vi "COD主界面（列队使用）.vi"() -> (8 "多列列表框":i32(listbox))   [LabVIEW 2016, in "斯坦道CODMn.lvlib"]
uses:
  <vilib>/Analysis/6fits.llb/Curve Fitting Criteria.ctl
  <vilib>/Utility/miscctls.llb/LVPointTypeDef.ctl
  <vilib>/Utility/config.llb/Read Key (I32).vi
  <vilib>/Utility/config.llb/Read Key (Double).vi
  <vilib>/Utility/config.llb/Read Key (Boolean).vi
  <vilib>/Utility/config.llb/Write Key (I32).vi
  <vilib>/Utility/config.llb/Write Key (Double).vi
  <vilib>/Utility/config.llb/Write Key (Boolean).vi
  <vilib>/Waveform/WDTFileIO.llb/Read Waveform from File.vi
  <vilib>/ptbypt/NI_PtbyPt.lvlib
  <vilib>/Utility/config.llb/NI_LVConfig.lvlib
  <vilib>/Analysis/NI_AALPro.lvlib
panel:
  out "氢氧化钠":dbl
  in  "序列号变更":bool
  out "模块版本号":string
  in  "更新程序":bool
  out "进样无液体告警":bool
  out "校准内容显示":string
  out "60分钟超时报警":bool
  in  "远程校准量程":enum16{"L", "H"}(ring)
  in  "远程自动校准浓度":dbl
  in  "仪器参数":bool
  out "CODMn序列号":string
  out "CODMn软件版本：":string
  in  "标样核查量程选择":enum32{"H", "L", "AUTO"}(ring)=enum."AUTO"
  in  "标样浓度":dbl
  in  "零点核查量程选择":enum32{"H", "L", "AUTO"}(ring)=enum."AUTO"
  in  "零点核查浓度":dbl
  out "序列号":string
  in  "采水泵排液时间/s:":i32
  in  "采水泵润洗时间/s:":i32
  in  "采水泵沉淀时间/s:":i32
  in  "采水泵进样时间/s:":i32
  in  "常规版/认证版":enum16{"常规版-酸性", "常规版-碱性", "认证版", "浮台版"}(ring)
  in  "释放串口":bool
  in  "打开串口":bool
  in  "保存参数":dbl[](array[numeric])
  out "报警数字":i16
  out "CODMn工作状态":T1(ring)
  out "ORP-K":string
  out "ORP-B":string
  out "ORP-A":string
  out "x = y?":bool
  out "稀释倍数解释":string
  in  "跨度量程选择":enum32{"H", "L", "AUTO"}(ring)=enum."AUTO"
  in  "跨度液浓度":dbl
  in  "水样：":dbl
  in  "蒸馏水：":dbl
  in  "标液：":dbl
  in  "零点核查样：":dbl
  in  "加标回收样：":dbl
  in  "草酸钠":dbl
  in  "高锰酸钾":dbl
  in  "硫酸":dbl
  out "量程解释说明":string
  in  "高切低阈值:":dbl
  in  "低切高阈值:":dbl
  in  "水样量程选择:":enum16{"L", "H", "自动切换测一次", "自动切换测两次"}(ring)
  in  "氢氧化钠：":dbl
  in  "标准液浓度":dbl
  in  "温度":dbl
  in  "恒温时间":dbl
  in  "当前量程：":enum16{"L", "H"}(ring)
  in  "CODMn零点核查选择":enum16{"零点核查走纯水管", "零点核查走零漂管"}(ring)
  in  "锁定按钮":bool
  in  "低量程稀释倍数:":i8=1
  in  "高量程稀释倍数:":i8=2
  in  "一键写入":bool
  in  "测量模式(公式)":u16(ring)=1 items=["水样测试"=1, "标样核查"=2, "零点核查"=3, "跨度核查"=4, "空白测试"=5, "平行样"=6, "加标回收"=7]
  out "基本量程(显示)":string
  out "测量模式(显示)":string
  out "数据时间":string
  out "断电排液标记":bool
  out "COM":string
  in  "启用5":bool
  in  "校准5":bool
  in  "泵滴定数5":dbl
  in  "浓度5":dbl
  in  "启用4":bool
  in  "校准4":bool
  in  "泵滴定数4":dbl
  in  "浓度4":dbl
  out "波形时间":timestamp
  in  "历史波形":bool
  out "滴定数-ORP值":u16[](array[numeric]) caption="数组"
  in  "关闭 3":bool
  in  "滴定曲线":bool
  out "ORP滴定曲线":u16[](graph)
  out "空白测试标记":bool
  out "跨度核查标记":bool
  in  "量程选择":enum16{"低量程", "高量程", "0-2量程"}(ring)
  in  "手动控制":bool
  in  "选用水样":enum16{"葡萄糖", "草酸钠"}(ring)
  in  "方程系数":cluster{"K":dbl, "b":dbl, "X^2":dbl} {"X^2" format="%#.6g"; "b" format="%#.6g"; "K" format="%#.6g"}
  out "多项式系数":dbl[](array[numeric])
  out "XY图":cluster{"X Values":dbl[], "Y Values":dbl[]}[](graph)
  in  "模型":enum32{"线性", "多项式"}(ring)
  out "启动时间":timestamp format="%<%Y/%m/%d %H:%M:%S>T"
  in  "关闭 2":bool
  out "r^2":dbl format="%.8g"
  out "拟合公式":string
  out "b":dbl format="%#.4g"
  out "K":dbl format="%#.4f"
  in  "启用3":bool
  in  "启用2":bool
  in  "启用1":bool
  in  "校准3":bool
  in  "校准2":bool
  in  "校准1":bool
  in  "泵滴定数3":dbl
  in  "泵滴定数2":dbl
  in  "泵滴定数1":dbl
  in  "浓度3":dbl
  in  "浓度2":dbl
  in  "浓度1":dbl
  in  "写入":bool
  out "零点核查标记":bool
  out "排液故障":bool
  out "进水样超量程":bool
  out "标样核查标记":bool
  out "平行样测量":bool
  out "加标回收测量":bool
  out "质控样测量":bool
  out "待机":bool
  out "校标错误":bool
  out "校零错误":bool
  out "测量错误":bool
  out "草酸钠报警":bool
  out "高锰酸钾报警":bool
  out "加热故障":bool
  out "温控器故障":bool
  out "ORP故障":bool
  out "排液标记":bool
  out "故障标记":bool
  out "校标标记":bool
  out "校零标记":bool
  out "通讯状态":bool
  out "水样测量":bool
  in  "读取":bool
  in  "返回":bool
  in  "校准配置":bool
  in  "零点泵计量数 2":dbl
  in  "标度泵计量数 2":dbl
  out "标度滴定值":dbl
  out "零点滴定值":dbl
  in  "保存":bool
  in  "关闭":bool
  out "仪器时间":timestamp format="%<%Y/%m/%d %H:%M:%S>T"
  out "秒":u16
  out "分":u16
  out "COD浓度（mg/L)":dbl format="%.2g"
  out "进样管":dbl
  out "高锰酸钾":dbl
  out "草酸钠":dbl
  out "硫酸":dbl
  out "实时ORP":dbl
  out "温度℃":dbl
  out "加热":bool
  out "搅拌":bool
  out "进硫酸":bool
  out "进加标回收样":bool
  out "进零点核查样":bool
  out "进标液":bool
  out "进蒸馏水":bool
  out "进水样":bool
  out "进草酸钠":bool
  out "进高锰酸钾":bool
  out "定时启动":bool
  in  "启动":bool
  in  "故障清除":bool
  in  "参数配置":bool
  in  "停止":bool
  in  "单步启动":bool
  out "系统时间":timestamp
  in  "时间校准":bool
  out "模式（受控）":u16
  # "测试时长："
  # "注：遇到加热故障和排液故障时仪器不能正常启动，\n必须排查故障并点击报警清除按钮方可运行。"
  # "mg/L"
  # "基本参数设置"
  # "校零校标结果"
  # "泵计量参数设置"
  # "校零结果："
  # "校零滴定值："
  # "加热恒温温度(℃):"
  # "高锰酸钾："
  # "校标结果："
  # "标度滴定值："
  # "恒温时间(分钟):"
  # "草酸钠："
  # "零点泵计量值："
  # "标准液浓度(mg/L):"
  # "硫酸："
  # "标度泵计量值："
  # "跨度核查浓度："
  # "跨度量程选择："
  # "零点核查浓度："
  # "标样浓度："
  # "零点量程选择："
  # "标样量程选择："
  # "远程校准配置区"
  # "公式读取写入区"
  # "mg/L"
  # "是否启用"
  # "泵滴定数"
  # "浓度"
  # "辅\n助\n计\n算\n区"
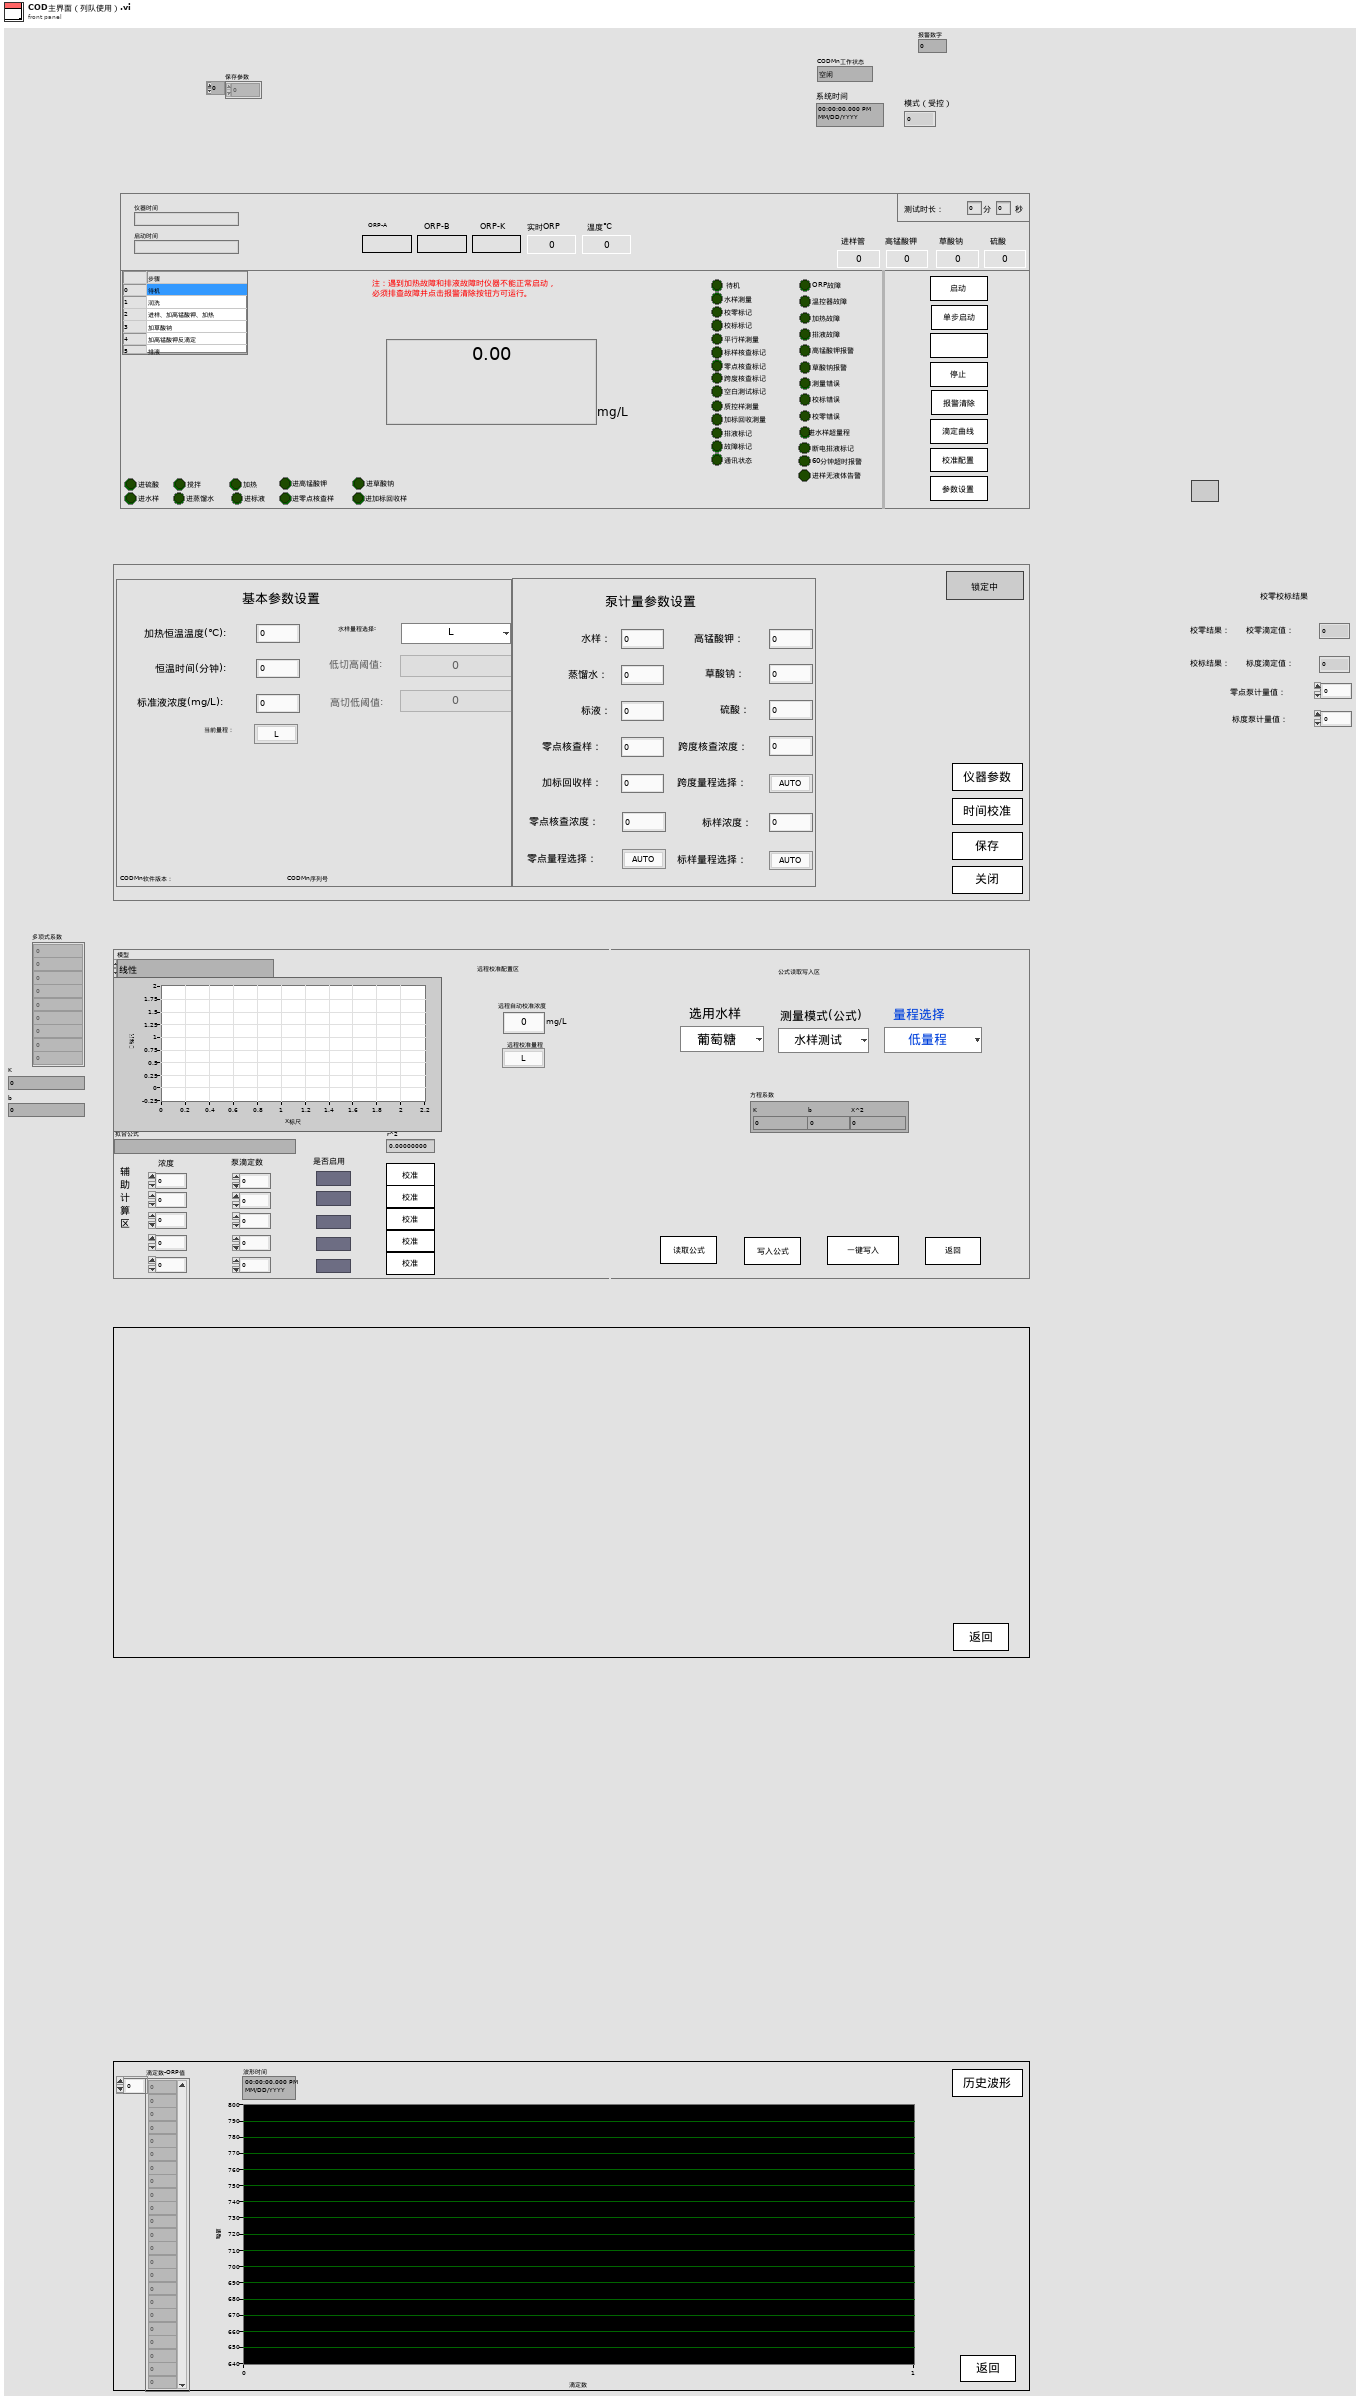
[diagram p1: front panel]
types:
  T1 = enum16{"空闲", "水样测试", "标样核查", "零点核查", "跨度核查", "空白测试", "平行样测试", "质控样", "空白校准", "标样校准", "加标回收"}
  T2 = typedef "LVPointTypeDef.ctl" = cluster{"Horizontal":i16, "Vertical":i16}
  T3 = cluster{"Major":u16, "Minor":u16, "Fix":u16, "Build":u16}
  T4 = typedef "NI_LVConfig.lvlib/Config Data RefNum.ctl" = refnum<k1>
  T5 = cluster{"时间标识":timestamp, "参数":string, "日志信息":string, "流程参数":string}
  T6 = cluster{"时间标识":timestamp, "设备":string, "日志信息":string, "流程参数":string}
  T7 = enum8{"Enabled", "Disabled", "Disabled and Grayed Out"}
  T8 = cluster{"时间":timestamp, "测量模式":string, "数据类型":string, "检测值":sgl, "单位":string, "数据标识":string, "因子编码":string, "标样参考值":sgl, "ORP-A":sgl, "ORP-B":sgl, "ORP-K":sgl, "COD滴定值":sgl, "高锰酸钾滴定数":sgl, "温度":sgl, "量程":sgl, "LastTime":timestamp, "序列号:":string}
  T9 = cluster{"因子编码":u32, "单位":u16, "标样参考值":sgl, "水样数据时间":timestamp, "水样实测值":sgl, "水样数据标识":string, "标样数据时间":timestamp, "标样实测值":sgl, "标样数据标识":string, "空白数据时间":timestamp, "空白实测值":sgl, "空白数据标识":string, "零点核查数据时间":timestamp, "零点核查实测值":sgl, "零点核查数据标识":string, "跨度核查数据时间":timestamp, "跨度核查实测值":sgl, "跨度核查数据标识":string, "加标回收数据时间":timestamp, "加标回收实测值":sgl, "加标回收数据标识":string, "平行样数据时间":timestamp, "平行样实测值":sgl, "平行样数据标识":string}
  T10 = cluster{"控制命令":enum16{"启动测量", "标样核查", "零点核查", "跨度核查", "空白测试", "平行样测试", "加标回收", "空白校准", "标样校准", "初始化（清洗）", "停止测试", "仪器重启", "校时", "模式设置", "测量间隔设置"}, "周期设置类型":enum16{"定点启动", "间隔启动"}, "定时功能启用":bool, "定时间隔":dbl, "24H周期设置":bool[], "零点核查时间":u16, "跨度核查时间":u16, "质控频次":enum16{"关闭", "每天", "星期一", "星期二", "星期三", "星期四", "星期五", "星期六", "星期日"}}
  T11 = cluster{"数组 2[0]":sgl, "数组 2[1]":sgl, "数组 2[2]":sgl, "数组 2[3]":sgl, "数组 2[4]":sgl, "数组 2[5]":sgl, "数组 2[6]":sgl, "数组 2[7]":sgl, "数组 2[8]":sgl, "数组 2[9]":sgl, "数组 2[10]":sgl, "数组 2[11]":sgl, "数组 2[12]":sgl, "数组 2[13]":sgl, "数组 2[14]":sgl, "数组 2[15]":sgl, "数组 2[16]":sgl, "数组 2[17]":sgl, "数组 2[18]":sgl, "数组 2[19]":sgl, "数组 2[20]":sgl, "数组 2[21]":sgl, "数组 2[22]":sgl, "数组 2[23]":sgl, "数组 2[24]":sgl, "数组 2[25]":sgl, "数组 2[26]":sgl, "数组 2[27]":sgl, "数组 2[28]":sgl, "数组 2[29]":sgl, "数组 2[30]":sgl, "数组 2[31]":sgl, "数组 2[32]":sgl, "数组 2[33]":sgl, "数组 2[34]":sgl, "数组 2[35]":sgl, "数组 2[36]":sgl, "数组 2[37]":sgl, "数组 2[38]":sgl, "数组 2[39]":sgl, "数组 2[40]":sgl, "数组 2[41]":sgl}
  T12 = cluster{"ORP故障":bool, "温控器故障":bool, "加热故障":bool, "高锰酸钾报警":bool, "草酸钠报警":bool, "测量错误":bool, "校零错误":bool, "校标错误":bool, " 进水样超量程":bool, "排液阀故障":bool, "60分钟超时报警":bool, "进样无液体报警":bool}
  T13 = cluster{"控制命令":enum16{"启动测量", "标样核查", "零点核查", "跨度核查", "空白测试", "平行样测试", "加标回收", "空白校准", "标样校准", "初始化（清洗）", "停止测试", "仪器重启", "校时", "模式设置", "测量间隔设置"}, "周期设置类型":enum16{"定点启动", "间隔启动"}, "定时功能启用":bool, "定时间隔":dbl, "24H周期设置":bool[], "空白核查时间":u16, "跨度核查时间":u16, "质控频次":enum16{"关闭", "每天", "星期一", "星期二", "星期三", "星期四", "星期五", "星期六", "星期日"}}
  T14 = cluster{"测量量程":dbl, "测量精度":dbl, "测量间隔":dbl, "消解温度":dbl, "消解时长":dbl, "空白校准时间":timestamp, "曲线截距":dbl, "曲线斜率":dbl, "测量检出限":dbl, "测量信号值":dbl, "线性相关系数":dbl, "二次多项式系数":dbl, "标样校准时间":timestamp, "稀释倍数":dbl, "三项式系数":dbl, "空白标定系数":dbl, "量程系数":dbl, "F0/ORPA":dbl, "F1/ORPB":dbl, "F2/ORPK":dbl, "F3":dbl, "F4":dbl, "F5":dbl, "F6":dbl, "F7":dbl, "X0/滴定数":dbl, "量程":dbl}
  T15 = cluster{"确定":bool, "测量量程":dbl, "测量精度":dbl, "测量间隔":dbl, "消解温度":dbl, "消解时长":dbl, "空白校准时间":timestamp, "曲线截距":dbl, "曲线斜率":dbl, "测量检出限":dbl, "测量信号值":dbl, "线性相关系数":dbl, "二次多项式系数":dbl, "标样校准时间":timestamp, "稀释倍数":dbl, "三项式系数":dbl, "空白标定系数":dbl, "量程系数":dbl, "F0/ORPA":dbl, "F1/ORPB":dbl, "F2/ORPK":dbl, "F3":dbl, "F4":dbl, "F5":dbl, "F6":dbl, "F7":dbl, "X0/滴定数":dbl, "量程":dbl}
  T16 = typedef "NI_AALPro.lvlib/Curve Fitting Criteria.ctl" = u16
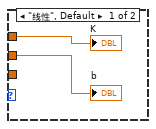
[diagram p5: hidden frame]
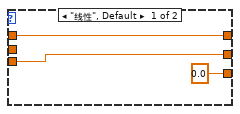
[diagram p7: hidden frame]
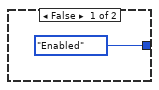
[diagram p8: hidden frame]
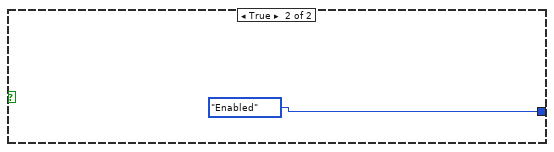
[diagram p9: hidden frame]
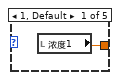
[diagram p14: hidden frame]
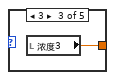
[diagram p15: hidden frame]
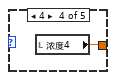
[diagram p16: hidden frame]
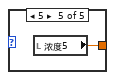
[diagram p17: hidden frame]
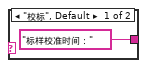
[diagram p18: hidden frame]
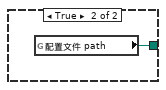
[diagram p19: hidden frame]
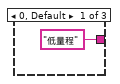
[diagram p20: hidden frame]
diagram:
  n1 = flat-sequence {
    tunnel: w1 -> [_]
    frame #0 {
      w18 = u16 1 items=["水样测试"=1, "标样核查"=2, "零点核查"=3, "跨度核查"=4, "空白测试"=5, "平行样"=6, "加标回收"=7] ("测量模式(公式)")
      n2 = vi-ref "斯坦道CODMn.lvlib:待机状态数据存储写入和切换量程(子VI).vi"() -> (w63:refnum<vi>)
      n3 = vi-ref "斯坦道CODMn.lvlib:定时启动 (子VI).vi"() -> (w50:refnum<vi>)
      n4 = vi-ref "斯坦道CODMn.lvlib:日志报警状态存储 (子VI).vi"() -> (w49:refnum<vi>)
      n5 = vi-ref "斯坦道CODMn.lvlib:高锰酸钾-ORP滴定曲线(子VI).vi"() -> (w36:refnum<vi>)
      n6 = property class="VI"(reference=w50, error in=errorcluster {"status"=FALSE, "code"=0, "source"=""} ("错误输出")) -> ("Name"=w51:string)  [unwired: 2 out]
      n7 = property class="VI"(reference=w49, error in=errorcluster {"status"=FALSE, "code"=0, "source"=""} ("错误输出")) -> ("Name"=w48:string)  [unwired: 2 out]
      n8 = property class="VI"(reference=w36, error in=errorcluster {"status"=FALSE, "code"=0, "source"=""} ("错误输出")) -> ("Name"=w37:string)  [unwired: 2 out]
      n9 = Open VI Reference(type specifier VI Refnum (for type only)=refnum<vi> refnum, vi path=w51, options=128 ("选项")) -> (vi reference=w31:refnum<vi>, error out=w53:errorcluster)  [unwired: 3 in]
      n10 = property class="VI"(reference=w63, error in=errorcluster {"status"=FALSE, "code"=0, "source"=""} ("错误输出")) -> ("Name"=w62:string)  [unwired: 2 out]
      n11 = call-by-ref "?"(reference=w31, error in=w53) -> (reference out=w55:refnum<vi>, error out=w54:errorcluster)  [unwired: 12 in]
      n12 = Open VI Reference(type specifier VI Refnum (for type only)=refnum<vi> refnum, vi path=w48, options=128 ("选项")) -> (vi reference=w32:refnum<vi>, error out=w46:errorcluster)  [unwired: 3 in]
      n13 = Open VI Reference(type specifier VI Refnum (for type only)=refnum<vi> refnum, vi path=w37, options=128 ("选项")) -> (vi reference=w35:refnum<vi>, error out=w39:errorcluster)  [unwired: 3 in]
      n14 = call-by-ref "?"(reference=w32, error in=w46) -> (reference out=w44:refnum<vi>, error out=w45:errorcluster)  [unwired: 12 in]
      n15 = Close Reference(reference=w55, error in (no error)=w54) -> ()  [unwired: 1 out]
      n16 = call-by-ref "?"(reference=w35, error in=w39) -> (reference out=w41:refnum<vi>, error out=w40:errorcluster)  [unwired: 12 in]
      n17 = Open VI Reference(type specifier VI Refnum (for type only)=refnum<vi> refnum, vi path=w62, options=128 ("选项")) -> (vi reference=w28:refnum<vi>, error out=w60:errorcluster)  [unwired: 3 in]
      n18 = Close Reference(reference=w44, error in (no error)=w45) -> ()  [unwired: 1 out]
      n19 = call-by-ref "?"(reference=w28, error in=w60) -> (reference out=w58:refnum<vi>, error out=w59:errorcluster)  [unwired: 12 in]
      n20 = Close Reference(reference=w41, error in (no error)=w40) -> ()  [unwired: 1 out]
      n21 = Close Reference(reference=w58, error in (no error)=w59) -> ()  [unwired: 1 out]
      n22 = vi-ref "斯坦道CODMn.lvlib:关键参数交互.vi"() -> (w25:refnum<vi>)
      n23 = property class="VI"(reference=w25, error in=errorcluster {"status"=FALSE, "code"=0, "source"=""} ("错误输出")) -> ("Name"=w24:string)  [unwired: 2 out]
      n24 = Open VI Reference(type specifier VI Refnum (for type only)=refnum<vi> refnum, vi path=w24, options=128 ("选项")) -> (vi reference=w26:refnum<vi>, error out=w22:errorcluster)  [unwired: 3 in]
      n25 = call-by-ref "?"(reference=w26, error in=w22, "量程选择"=enum16{"低量程", "高量程", "0-2量程"}."低量程", "测量模式(公式)"=w18, "模型"=enum32{"线性", "多项式"}."线性") -> (reference out=w20:refnum<vi>, error out=w21:errorcluster)  [unwired: 9 in]
      n26 = Close Reference(reference=w20, error in (no error)=w21) -> ()  [unwired: 1 out]
    }
  }
  n27 = flat-sequence {
    tunnel: [w66] -> w3
    tunnel: [errorcluster {"status"=FALSE, "code"=0, "source"=""} ("错误输出")] -> w1
    tunnel: [w68] -> w2
    frame #0 {
      w90 = "192.168.1.100" ("名称")
      n28 = global write "COD内部交互全局.vi" "量程切换次数"(u8 0 ("量程切换次数")) -> ()
      n29 = global write "COD内部交互全局.vi" "切换量程连续测两次"(FALSE ("切换量程连续测两次")) -> ()
      n30 = global read "COD内部交互全局.vi" "序列号:"() -> (w97:string)
      n31 = property on="窗格" class="Pane"("Origin"=T2 {"Horizontal"=0, "Vertical"=0} ("原点")) -> ()  [unwired: 2 in, 2 out]
      n32 = Empty String/Path?(string/path=w97) -> (empty?=w65:bool)
      n33 = case shown="真" w65 {
        tunnel: w97 -> [w112 _]
        tunnel: [w111 "data\\CODMnSet.ini" ("名称或相对路径")] -> w78
        frame False {
          # "与生产用上位机交互"
          n34 = Concatenate Strings("data\\" ("字符串"), "序列号" ("字符串"), w112, "Set.ini" ("名称或相对路径")) -> (w111:string)
        }
        frame True {
        }
      }
      n35 = String To IP(1:w90) -> (0:w83:u32)
      n36 = IP To String(2:w83) -> (0:w86:string)  [unwired: 1 in]
      n37 = Not Equal?(x=w90, y=w86) -> (x != y?=w91:bool)
      n38 = Concatenate Strings("\\\\" ("字符串"), w86) -> (w85:string)
      n39 = global write "CODMN外部API.vi" "ping"(w91) -> ()
      n40 = String To Path(string=w85) -> (path=w92:path)
      n41 = Build Path(base path=w92, name or relative path=w78) -> (appended path=w87:path)
      n42 = local write "量程选择"(enum16{"低量程", "高量程", "0-2量程"}."低量程" ("量程选择")) -> ()
      n43 = local write "选用水样"(enum16{"葡萄糖", "草酸钠"}."葡萄糖" ("选用水样")) -> ()
      n44 = global write "COD内部交互全局.vi" "配置文件ini"(w78) -> ()
      n45 = case shown="真" w91 {
        tunnel: w87 -> [w102 w106]
        tunnel: [w102 w105] -> w88
        tunnel: [FALSE w104] -> w89
        frame False {
        }
        frame True {
          n46 = call <vilib>:"Check if File or Folder Exists.vi"("path"=w106) -> ("file or folder exists?"=w104:bool, "dup path"=w105:path)  [unwired: 8 in, 1 out]
        }
      }
      n47 = control-ref of="本VI"() -> (w77:refnum<vi>)
      n48 = case shown="假" w89 {
        tunnel: w88 -> [_ w110]
        tunnel: [w108 w110] -> w69
        tunnel: w78 -> [w107 _]
        frame False {
          # "本地文件地址"
          n49 = call <vilib>:"Application Directory.vi"() -> ("Application Directory"=w109:path)
          n50 = Build Path(base path=w109, name or relative path=w107) -> (appended path=w108:path)
        }
        frame True {
          # "网络共享地址"
        }
      }
      n51 = property class="VI"(reference=w77) -> ("Library.Version"=w76:T3)  [unwired: 1 in, 2 out]
      n52 = Unbundle By Name(w76) -> ("Major"=w74:u16, "Minor"=w73:u16, "Fix"=w72:u16, "Build"=w71:u16)
      n53 = Format Into String(format string="模块版本号：%d.%d.%d.%d" ("格式字符串"), w74, w73, w72, w71) -> (resulting string=→"模块版本号":string)  [unwired: 2 in, 1 out]
      n54 = global write "CODMN外部API.vi" "配置文件 path"(w69) -> ()
      n55 = call <vilib>:"Open Config Data.vi"("configuration file path"=w69) -> ("error out"=w79:errorcluster, "refnum"=w80:T4)  [unwired: 8 in, 1 out]
      n56 = vi-ref "斯坦道CODMn.lvlib:CODMn断电保存全局变量.vi"() -> (w93:refnum<vi>)
      n57 = call <userlib>:"Read Panel from INI__ogtk.vi"("error in (no error)"=w79, "VI ref"=w93, "refnum"=w80) -> ("error out"=w81:errorcluster, "refnum out"=w82:T4)  [unwired: 7 in]
      n58 = call <vilib>:"Close Config Data.vi"("error in (no error)"=w81, "refnum"=w82) -> ("error out"=w67:errorcluster)  [unwired: 8 in, 1 out]
      n59 = call <vilib>:"Clear Errors.vi"("error in (no error)"=w67) -> ("error out"=w64:errorcluster)  [unwired: 5 in, 1 out]
      n60 = Read from Text File(file (use dialog)=w69, error in=w64) -> (text=w68:string, error out=w66:errorcluster)  [unwired: 2 in, 2 out]
      "稀释倍数解释" <- "稀释倍数解释：\n稀释倍数选择1，表示不稀释\n默认低量程系数倍数1，高量程系数倍数2\n则低量程为0~8，高量程为0~16" ("稀释倍数解释")
    }
  }
  n61 = Obtain Queue(name (unnamed)="CODMn" ("名称（未命名）"), element data type=cluster{"命令":string} {"命令"="启用模块"} ("元素")) -> (queue out=w13:refnum<queue>, error out=w12:errorcluster)  [unwired: 3 in, 1 out]
  n62 = while {
    tunnel: [w123] -> _
    shift-right: [w121] -> _
    shift-left: w2 -> [w120]
    tunnel: w3 -> [_]
    stop <- FALSE stop-if-true
    n63 = global read "CODMN外部API.vi" "配置文件 path"() -> (w117:path)
    n64 = Wait (ms)(milliseconds to wait=u32 1000 ("等待时间（毫秒）")) -> ()  [unwired: 1 out]
    n65 = Read from Text File(file (use dialog)=w117) -> (text=w121:string, error out=w118:errorcluster)  [unwired: 3 in, 2 out]
    n66 = Not Equal?(x=w121, y=w120) -> (x != y?=w119:bool)
    n67 = case shown="真" w119 {
      tunnel: [w125 w132] -> w123
      tunnel: w117 -> [_ w126]
      tunnel: w118 -> [w125 _]
      frame False {
      }
      frame True {
        # "文件发生改变进行更新，远端和本地都更新"
        n68 = vi-ref "斯坦道CODMn.lvlib:CODMn断电保存全局变量.vi"() -> (w127:refnum<vi>)
        n69 = call <vilib>:"Open Config Data.vi"("configuration file path"=w126) -> ("error out"=w131:errorcluster, "refnum"=w130:T4)  [unwired: 8 in, 1 out]
        n70 = call <userlib>:"Read Panel from INI__ogtk.vi"("error in (no error)"=w131, "VI ref"=w127, "refnum"=w130) -> ("error out"=w129:errorcluster, "refnum out"=w128:T4)  [unwired: 7 in]
        n71 = call <vilib>:"Close Config Data.vi"("error in (no error)"=w129, "refnum"=w128) -> ("error out"=w132:errorcluster)  [unwired: 8 in, 1 out]
      }
    }
  }
  n72 = vi-ref "CODMn通讯.vi"() -> (w4:refnum<vi>)
  n73 = while {
    stop <- FALSE stop-if-true
    # "相差60秒自动校时"
    n74 = global read "运行时序全局变量.vi" "多列列表框"() -> (w134:i32)
    n75 = local read "仪器时间"() -> (w141:timestamp)
    n76 = local read "系统时间"() -> (w142:timestamp)
    n77 = Wait (ms)(milliseconds to wait=u32 1000 ("等待时间（毫秒）")) -> ()  [unwired: 1 out]
    n78 = Build Array(w141) -> (w140:timestamp[])
    n79 = Build Array(w142) -> (w159:timestamp[])
    n80 = Equal?(x=w134, y=u16 5) -> (x = y?=w136:bool)
    n81 = call <vilib>:"Boolean Crossing PtByPt.vi"("direction"=enum16{"either", "false-true", "true-false"}."false-true", "input"=w136) -> ("crossing"=w133:bool)  [unwired: 1 in]
    n82 = call "DateToHex.vi"("DATE"=w140) -> ("数组"=w153:u16[])  [unwired: 10 in]
    n83 = call "DateToHex.vi"("DATE"=w159) -> ("数组"=w158:u16[])  [unwired: 10 in]
    n84 = case shown="真" w133 {
      frame False {
      }
      frame True {
        # "校准结束后自动更新曲线泵滴定数"
        n85 = global read "COD测量模式全局.vi" "测量模式文字实时"() -> (w160:string)
        n86 = global read "COD测量模式全局.vi" "测量模式文字实时"() -> (w165:string)
        n87 = global read "CODMN外部API.vi" "远程反控校准CODMn"() -> (w164:bool)
        n88 = global read "COD内部交互全局.vi" "高锰酸钾"() -> (w168:dbl)
        n89 = Equal?(x=w160, y="校零") -> (x = y?=w161:bool)
        n90 = Equal?(x=w165, y="校标") -> (x = y?=w167:bool)
        n91 = Or(x=w161, y=w167) -> (x .or. y?=w163:bool)
        n92 = case shown="真" w163 {
          tunnel: w168 -> [_ w175]
          tunnel: w160 -> [_ w172]
          frame False {
          }
          frame True {
            w199 = "量程选择" ("section")
            n93 = global read "CODMN外部API.vi" "ping"() -> (w210:bool)
            n94 = case shown="\"校零\"" w172 {
              tunnel: ["标样校准时间：" "空白校准时间："] -> w178
              frame "校标", Default {
              }
              frame "校零" {
              }
            }
            n95 = case shown="假" w210 {
              tunnel: [w219 w222] -> w211
              frame False {
                n96 = global read "COD内部交互全局.vi" "配置文件ini"() -> (w221:string)
                n97 = call <vilib>:"Application Directory.vi"() -> ("Application Directory"=w220:path)
                n98 = Build Path(base path=w220, name or relative path=w221) -> (appended path=w219:path)
              }
              frame True {
                n99 = global read "CODMN外部API.vi" "配置文件 path"() -> (w222:path)
              }
            }
            n100 = Number To Fractional String(number=w175) -> (F-format string=w180:string)  [unwired: 3 in]
            n101 = call <vilib>:"Open Config Data.vi"("configuration file path"=w211) -> ("error out"=w198:errorcluster, "refnum"=w197:T4)  [unwired: 8 in, 1 out]
            n102 = Get Date/Time In Seconds() -> (seconds since 1Jan1904=w176:timestamp)
            n103 = Format Date/Time String(time format string (%c)="%Y/%m/%d %H:%M:%S" ("时间格式字符串(%c)"), seconds (now)=w176) -> (date/time string=w177:string)  [unwired: 1 in]
            n104 = call-poly <vilib>:"Read Key.vi"("section"="标线选择", "error in (no error)"=w198, "key"="选用水样", "refnum"=w197) -> ("error out"=w200:errorcluster, "value"=w193:i32, "refnum out"=w201:T4)  [unwired: 4 in, 1 out]
            n105 = local write "选用水样"(w193) -> ()
            n106 = call-poly <vilib>:"Read Key.vi"("section"=w199, "error in (no error)"=w200, "key"=w199, "refnum"=w201) -> ("error out"=w194:errorcluster, "value"=w196:i32, "refnum out"=w195:T4)  [unwired: 4 in, 1 out]
            n107 = case shown="1" w193 {
              tunnel: ["葡萄糖标线" ("section") "草酸钠标线" ("section")] -> w208
              frame 0, Default {
              }
              frame 1 {
              }
            }
            n108 = local write "量程选择"(w196) -> ()
            n109 = case shown="2" w196 {
              tunnel: ["低量程" "高量程" "0-2量程"] -> w207
              frame 0, Default {
              }
              frame 1 {
              }
              frame 2 {
              }
            }
            n110 = Concatenate Strings(w208, w207) -> (w209:string)
            n111 = call-poly <vilib>:"Read Key.vi"("section"=w209, "error in (no error)"=w194, "key"="当前选用的校准" ("section"), "refnum"=w195) -> ("error out"=w206:errorcluster, "value"=w171:i32, "refnum out"=w205:T4)  [unwired: 4 in, 1 out]
            n112 = call <vilib>:"Close Config Data.vi"("error in (no error)"=w206, "refnum"=w205) -> ()  [unwired: 8 in, 2 out]
            n113 = case shown="2" w171 {
              tunnel: [w212 w213 w214 w215 w216] -> w170
              frame 1, Default {
                n114 = local read "浓度1"() -> (w212:dbl)
              }
              frame 2 {
                n115 = local read "浓度2"() -> (w213:dbl)
              }
              frame 3 {
                n116 = local read "浓度3"() -> (w214:dbl)
              }
              frame 4 {
                n117 = local read "浓度4"() -> (w215:dbl)
              }
              frame 5 {
                n118 = local read "浓度5"() -> (w216:dbl)
              }
            }
            n119 = Number To Fractional String(number=w170) -> (F-format string=w182:string)  [unwired: 3 in]
            n120 = Concatenate Strings("信息：校准结果：\n", "校准浓度：", w182, "滴定数：", w180, w178, w177) -> (w174:string)
            n121 = Bundle(cluster=T5 {"时间标识"=timestamp(0 s since 1904-01-01), "参数"="", "日志信息"="", "流程参数"=""} ("data in"), "时间标识"=w176, "参数"="CODMn" ("table输入"), "日志信息"=w174, "流程参数"="" ("table输入")) -> (w186:T5)
            n122 = call "流程日志字段定义.vi"("table输入"="校准记录", "data in"=w186) -> ("table输出"=w190:string, "columns"=w191:string[], "data out"=w192:T6)  [unwired: 7 in]
            n123 = call "插入数据.vi"("data"=w192, "columns"=w191, "database"="database3.mdb", "table"=w190) -> ()  [unwired: 7 in, 1 out]
            n124 = global write "COD内部交互全局.vi" "当前校准"(w171) -> ()
            n125 = case shown="1, 默认" w171 {
              tunnel: w175 -> [w228 w229 w230 w231 w232]
              frame 1, Default {
                n126 = property on="泵滴定数1" class="DigNum (严格)"("Val(Sgnl)"=w228) -> ()  [unwired: 2 in, 2 out]
              }
              frame 2 {
                n127 = property on="泵滴定数2" class="DigNum (严格)"("Val(Sgnl)"=w229) -> ()  [unwired: 2 in, 2 out]
              }
              frame 3 {
                n128 = property on="泵滴定数3" class="DigNum (严格)"("Val(Sgnl)"=w230) -> ()  [unwired: 2 in, 2 out]
              }
              frame 4 {
                n129 = property on="泵滴定数4" class="DigNum (严格)"("Val(Sgnl)"=w231) -> ()  [unwired: 2 in, 2 out]
              }
              frame 5 {
                n130 = property on="泵滴定数5" class="DigNum (严格)"("Val(Sgnl)"=w232) -> ()  [unwired: 2 in, 2 out]
              }
            }
          }
        }
        n131 = case shown="真" w164 {
          frame False {
          }
          frame True {
            # "校准完自动写入公式"
            n132 = global write "CODMN外部API.vi" "远程反控校准CODMn"(FALSE ("远程反控校准CODMn")) -> ()
          }
        }
      }
    }
    n133 = Index Array(array=w153, index=2 ("索引")) -> (element=w155:u16)
    n134 = Index Array(array=w158, index=2 ("索引")) -> (element=w156:u16)
    n135 = Split Number(x=w155) -> (hi(x)=w149:u8)  [unwired: 1 out]
    n136 = Split Number(x=w156) -> (hi(x)=w152:u8)  [unwired: 1 out]
    n137 = To Byte Integer(number=w149) -> (8bit integer=w148:i8)
    n138 = To Byte Integer(number=w152) -> (8bit integer=w151:i8)
    n139 = Subtract(x=w148, y=w151) -> (x-y=w150:i8)
    n140 = Absolute Value(x=w150) -> (abs(x)=w147:i8)
    n141 = local read "通讯状态"() -> (w144:bool)
    n142 = Greater Or Equal?(x=w147, y=i8 5) -> (x >= y?=w145:bool)
    n143 = And(x=w145, y=w144) -> (x .and. y?=w143:bool)
    n144 = case shown="真" w143 {
      frame False {
      }
      frame True {
        # "相差60秒时间自动校准"
        n145 = flat-sequence {
          frame #0 {
            n146 = property on="时间校准" class="Bool (严格)"("Val(Sgnl)"=TRUE ("值(信号)")) -> ()  [unwired: 2 in, 2 out]
          }
          frame #1 {
            n147 = Wait (ms)(milliseconds to wait=u32 500 ("等待时间（毫秒）")) -> ()  [unwired: 1 out]
          }
          frame #2 {
            n148 = property on="时间校准" class="Bool (严格)"("Val(Sgnl)"=FALSE ("值(信号)")) -> ()  [unwired: 2 in, 2 out]
          }
        }
      }
    }
  }
  n149 = while {
    tunnel: w3 -> [_]
    stop <- FALSE stop-if-true
    # "赋值循环"
    n150 = flat-sequence {
      frame #0 {
        # "测量数据区"
        n151 = global read "COD内部交互全局.vi" "data"() -> (w480:T8)
        n152 = global read "COD测量模式全局.vi" "测量模式文字实时"() -> (w466:string)
        "测量模式(显示)" <- w466
        n153 = global read "CODMn断电保存全局变量.vi" "测量数据区"() -> (w475:T9)
        n154 = Unbundle By Name(w480) -> ("时间"=w479:timestamp, "检测值"=w478:sgl, "数据标识"=w477:string)
        n155 = case shown="\"水样测试\"" w466 {
          tunnel: w475 -> [w481 w486 w491 w496 w501 w506 w511 w516 w521 w526]
          tunnel: [w481 w485 w490 w492 w500 w505 w510 w515 w517 w525] -> w476
          tunnel: w479 -> [_ w484 w489 w495 w499 w504 w509 w514 w520 w524]
          tunnel: w478 -> [_ w483 w488 w494 w498 w503 w508 w513 w519 w523]
          tunnel: w477 -> [_ w482 w487 w493 w497 w502 w507 w512 w518 w522]
          frame "", Default {
          }
          frame "水样测试" {
            n156 = Bundle By Name(cluster=w486, "水样数据时间"=w484, "水样实测值"=w483, "水样数据标识"=w482) -> (w485:T9)
          }
          frame "标样核查" {
            n157 = Bundle By Name(cluster=w491, "标样数据时间"=w489, "标样实测值"=w488, "标样数据标识"=w487) -> (w490:T9)
          }
          frame "跨度核查" {
            n158 = Bundle By Name(cluster=w496, "跨度核查数据时间"=w495, "跨度核查实测值"=w494, "跨度核查数据标识"=w493) -> (w492:T9)
          }
          frame "零点核查" {
            n159 = Bundle By Name(cluster=w501, "零点核查数据时间"=w499, "零点核查实测值"=w498, "零点核查数据标识"=w497) -> (w500:T9)
          }
          frame "空白测试" {
            n160 = Bundle By Name(cluster=w506, "空白数据时间"=w504, "空白实测值"=w503, "空白数据标识"=w502) -> (w505:T9)
          }
          frame "加标回收" {
            n161 = Bundle By Name(cluster=w511, "加标回收数据时间"=w509, "加标回收实测值"=w508, "加标回收数据标识"=w507) -> (w510:T9)
          }
          frame "平行样" {
            n162 = Bundle By Name(cluster=w516, "平行样数据时间"=w514, "平行样实测值"=w513, "平行样数据标识"=w512) -> (w515:T9)
          }
          frame "校零" {
            n163 = Bundle By Name(cluster=w521, "空白数据时间"=w520, "空白实测值"=w519, "空白数据标识"=w518) -> (w517:T9)
          }
          frame "校标" {
            n164 = Bundle By Name(cluster=w526, "标样数据时间"=w524, "标样实测值"=w523, "标样数据标识"=w522) -> (w525:T9)
          }
        }
        n165 = Unbundle By Name(w475) -> ("水样实测值"=w472:sgl)
        n166 = feedback-in #1(w475) -> ()
        n167 = feedback #1(w475) -> (w474:T9)
        n168 = global read "CODMn断电保存全局变量.vi" "水样测试量程"() -> (w468:enum16{"L", "H"})
        n169 = Unbundle By Name(w474) -> ("水样实测值"=w473:sgl)
        n170 = feedback #2(w468) -> (w469:enum16{"L", "H"})
        n171 = feedback-in #2(w468) -> ()
        n172 = Not Equal?(x=w469, y=w468) -> (x != y?=w467:bool)
        n173 = Not Equal?(x=w472, y=w473) -> (x != y?=w471:bool)
        n174 = global write "CODMn断电保存全局变量.vi" "测量数据区"(w476) -> ()
        n175 = Or(x=w471, y=w467) -> (x .or. y?=w470:bool)
        n176 = case shown="真" w470 {
          frame False {
          }
          frame True {
            # "水样值发送改变存储本地"
            n177 = call "配置文件保存.vi"() -> ()  [unwired: 12 in]
          }
        }
      }
    }
    n178 = flat-sequence {
      frame #0 {
        # "局部变量给内部交互用全局变量"
        n179 = local read "温度℃"() -> (w262:dbl)
        n180 = local read "COD浓度（mg/L)"() -> (w268:dbl)
        n181 = local read "CODMn工作状态"() -> (w271:T1)
        n182 = local read "多列列表框"() -> (w269:i32)
        n183 = local read "标准液浓度"() -> (w267:dbl)
        n184 = local read "高锰酸钾报警"() -> (w265:bool)
        n185 = local read "断电排液标记"() -> (w264:bool)
        n186 = local read "实时ORP"() -> (w261:dbl)
        n187 = local read "故障标记"() -> (w270:bool)
        n188 = local read "高锰酸钾"() -> (w263:dbl)
        n189 = global write "COD内部交互全局.vi" "实时温度"(w262) -> ()
        n190 = local read "待机"() -> (w266:bool)
        n191 = global write "运行时序全局变量.vi" "多列列表框"(w269) -> ()
        n192 = global write "COD内部交互全局.vi" "故障标记"(w270) -> ()
        n193 = global write "COD内部交互全局.vi" "ORP显示"(w261) -> ()
        n194 = global write "COD浓度全局变量.vi" "标准液浓度"(w267) -> ()
        n195 = global write "COD内部交互全局.vi" "高锰酸钾"(w263) -> ()
        n196 = global write "COD内部交互全局.vi" "待机"(w266) -> ()
        n197 = global write "COD测量模式全局.vi" "CODMn工作状态"(w271) -> ()
        n198 = global write "COD内部交互全局.vi" "高锰酸钾报警"(w265) -> ()
        n199 = global write "COD内部交互全局.vi" "断电排液标记"(w264) -> ()
        n200 = global write "COD浓度全局变量.vi" "COD浓度（mg/L)"(w268) -> ()
      }
    }
    n201 = flat-sequence {
      frame #0 {
        # "断电保存全局给局部变量"
        n202 = global read "CODMn断电保存全局变量.vi" "高切低阈值:"() -> (w541:dbl)
        n203 = global read "CODMn断电保存全局变量.vi" "低切高阈值:"() -> (w540:dbl)
        n204 = global read "CODMn断电保存全局变量.vi" "跨度液浓度"() -> (w538:dbl)
        n205 = global read "COD内部交互全局.vi" "波形时间"() -> (→"波形时间":timestamp)
        n206 = global read "CODMn断电保存全局变量.vi" "启动时间"() -> (→"启动时间":timestamp)
        n207 = global read "CODMn断电保存全局变量.vi" "标样浓度"() -> (w536:dbl)
        n208 = global read "CODMn断电保存全局变量.vi" "定时控制"() -> (w531:T10)
        n209 = global read "CODMn断电保存全局变量.vi" "CODMn跨度量程选择"() -> (w542:enum32{"H", "L", "AUTO"})
        n210 = global read "CODMn断电保存全局变量.vi" "标样核查量程选择"() -> (w533:enum32{"H", "L", "AUTO"})
        n211 = global read "CODMn断电保存全局变量.vi" "零点核查量程选择"() -> (w535:enum32{"H", "L", "AUTO"})
        n212 = global read "CODMn断电保存全局变量.vi" "测量模式(公式)"() -> (w543:u16)
        n213 = global read "COD内部交互全局.vi" "滴定数-ORP值"() -> (→"滴定数-ORP值":u16[])
        n214 = global read "CODMn断电保存全局变量.vi" "常规版/认证版"() -> (w537:enum16{"常规版-酸性", "常规版-碱性", "认证版", "浮台版"})
        n215 = global read "CODMn断电保存全局变量.vi" "自动切换量程:"() -> (w539:enum16{"L", "H", "自动切换测一次", "自动切换测两次"})
        n216 = global read "CODMn断电保存全局变量.vi" "零点核查浓度"() -> (w534:dbl)
        n217 = global read "COD内部交互全局.vi" "ORP滴定曲线"() -> (→"ORP滴定曲线":u16[])
        n218 = local write "高切低阈值:"(w541) -> ()
        n219 = local write "标样浓度"(w536) -> ()
        n220 = Unbundle By Name(w531) -> ("定时功能启用"=→"定时启动":bool)
        n221 = local write "跨度液浓度"(w538) -> ()
        n222 = local write "低切高阈值:"(w540) -> ()
        n223 = local write "标样核查量程选择"(w533) -> ()
        n224 = local write "水样量程选择:"(w539) -> ()
        n225 = local write "常规版/认证版"(w537) -> ()
        n226 = local write "零点核查浓度"(w534) -> ()
        n227 = local write "零点核查量程选择"(w535) -> ()
        n228 = local write "测量模式(公式)"(w543) -> ()
        n229 = local write "跨度量程选择"(w542) -> ()
      }
    }
    n230 = flat-sequence {
      frame #0 {
        # "保存参数赋值"
        n231 = Multiply(x="温度", y=10.0) -> (x*y=w246:dbl)
        n232 = Multiply(x="标准液浓度", y=100.0) -> (x*y=w243:dbl)
        n233 = Build Array(w246, "恒温时间", w243, "氢氧化钠：", "当前量程：", "水样：", "蒸馏水：", "标液：", "零点核查样：", "加标回收样：", "高锰酸钾", "草酸钠", "硫酸", "零点泵计量数 2", "标度泵计量数 2", "高量程稀释倍数:", "低量程稀释倍数:", "CODMn零点核查选择") -> (w240:dbl[])
        n234 = local write "保存参数"(w240) -> ()
      }
    }
    n235 = flat-sequence {
      frame #0 {
        # "显示量程说明"
        n236 = global read "COD内部交互全局.vi" "通讯状态"() -> (→"通讯状态":bool)
        n237 = global read "CODMn断电保存全局变量.vi" "MB通信方式选择"() -> (w544:enum16{"串口", "TCP"})
        n238 = local read "低量程稀释倍数:"() -> (w558:i8)
        n239 = local read "高量程稀释倍数:"() -> (w548:i8)
        n240 = case shown="\"TCP\"" w544 {
          tunnel: [w561 w562] -> w549
          frame "串口", Default {
            n241 = global read "CODMn断电保存全局变量.vi" "VISA resource name"() -> (w561:refnum<visa-resource-name>)
          }
          frame "TCP" {
            n242 = global read "CODMn断电保存全局变量.vi" "IP"() -> (w562:string)
          }
        }
        "COM" <- w549
        n243 = Multiply(x=w558, y=i8 8) -> (x*y=w550:i8)
        n244 = Multiply(x=w548, y=i8 8) -> (x*y=w546:i8)
        n245 = Number To Decimal String(number=w550) -> (decimal integer string=w555:string)  [unwired: 1 in]
        n246 = Number To Decimal String(number=w546) -> (decimal integer string=w553:string)  [unwired: 1 in]
        n247 = Concatenate Strings("L低量程范围:0~" ("量程解释说明"), w555, "(mg/L)\n\nH高量程范围:" ("量程解释说明"), "0" ("字符串"), "~" ("量程解释说明"), w553, "(mg/L)" ("量程解释说明")) -> (→"量程解释说明":string)
      }
    }
    n248 = flat-sequence {
      frame #0 {
        # "参数赋值（只在读取参数时候改变一次）"
        n249 = global read "COD内部交互全局.vi" "读取浮台参数显示"() -> (w273:bool)
        n250 = global read "COD内部交互全局.vi" "读取浮台参数"() -> (w272:u16[])
        n251 = global read "COD内部交互全局.vi" "读取参数显示"() -> (w274:bool)
        n252 = global read "COD内部交互全局.vi" "读取参数"() -> (w275:u16[])
        n253 = case shown="真" w273 {
          tunnel: w272 -> [_ w281]
          frame False {
          }
          frame True {
            n254 = Index Array(array=w281) -> (element #1=w280:u16, element #2=w279:u16, element #3=w278:u16, element #4=w277:u16)  [unwired: 4 in]
            n255 = global write "COD内部交互全局.vi" "读取浮台参数显示"(FALSE ("读取参数显示")) -> ()
            n256 = local write "采水泵进样时间/s:"(w280) -> ()
            n257 = local write "采水泵润洗时间/s:"(w279) -> ()
            n258 = local write "采水泵沉淀时间/s:"(w278) -> ()
            n259 = local write "采水泵排液时间/s:"(w277) -> ()
          }
        }
        n260 = case shown="真" w274 {
          tunnel: w275 -> [_ w299]
          frame False {
          }
          frame True {
            n261 = Index Array(array=w299) -> (element #1=w308:u16, element #2=w320:u16, element #3=w304:u16, element #4=w282:u16, element #5=w307:u16, element #6=w306:u16, element #7=w319:u16, element #8=w318:u16, element #9=w317:u16, element #10=w316:u16, element #11=w315:u16, element #12=w314:u16, element #13=w313:u16, element #14=w312:u16, element #15=w311:u16, element #16=w302:u16, element #17=w301:u16, element #18=w300:u16, element #19=w297:u16, element #20=w296:u16, element #21=w295:u16, element #22=w294:u16, element #23=w293:u16, element #27=w289:u16, element #28=w288:u16, element #29=w287:u16, element #30=w286:u16, element #31=w285:u16)  [unwired: 31 in, 3 out]
            n262 = global write "COD内部交互全局.vi" "读取参数显示"(FALSE ("读取参数显示")) -> ()
            n263 = local write "水样："(w306) -> ()
            n264 = local write "标液："(w318) -> ()
            n265 = local write "硫酸"(w313) -> ()
            n266 = local write "零点核查样："(w317) -> ()
            n267 = local write "加标回收样："(w316) -> ()
            n268 = local write "当前量程："(w307) -> ()
            n269 = local write "蒸馏水："(w319) -> ()
            n270 = local write "恒温时间"(w320) -> ()
            n271 = local write "高锰酸钾"(w315) -> ()
            n272 = local write "草酸钠"(w314) -> ()
            n273 = local write "零点泵计量数 2"(w312) -> ()
            n274 = local write "标度泵计量数 2"(w311) -> ()
            n275 = local write "高量程稀释倍数:"(w302) -> ()
            n276 = local write "低量程稀释倍数:"(w301) -> ()
            n277 = local write "CODMn零点核查选择"(w300) -> ()
            n278 = Build Array(w297, w296, w295, w294, w293) -> (w292:u16[])
            n279 = Build Array(w289, w288, w287, w286, w285) -> (w284:u16[])
            n280 = Divide(x=w308, y=u16 10) -> (x/y=w309:dbl)
            n281 = Divide(x=w304, y=u16 100) -> (x/y=w303:dbl)
            n282 = local write "氢氧化钠："(w282) -> ()
            n283 = local write "温度"(w309) -> ()
            n284 = local write "标准液浓度"(w303) -> ()
            n285 = call "HexToString.vi"("数组"=w284) -> ("字符串"=w283:string)  [unwired: 10 in]
            "CODMn序列号" <- w283
            "序列号" <- w283
            n286 = call "FATEK_HexToString.vi"("数组"=w292) -> ("STRING"=w291:string[])  [unwired: 10 in]
            n287 = Index Array(array=w291) -> (element=→"CODMn软件版本：":string)  [unwired: 1 in]
            n288 = global write "COD内部交互全局.vi" "序列号:"(w283) -> ()
          }
        }
      }
    }
    n289 = flat-sequence {
      frame #0 {
        # "权限隐藏和显示功能"
        n290 = local read "x = y?"() -> (w564:bool)
        n291 = property on="更新程序" class="Bool (严格)"("Visible"=w564) -> ()  [unwired: 2 in, 2 out]
        n292 = property on="释放串口" class="Bool"("Visible"=w564) -> ()  [unwired: 2 in, 2 out]
        n293 = property on="打开串口" class="Bool"("Visible"=w564) -> ()  [unwired: 2 in, 2 out]
        n294 = property on="序列号变更" class="Bool"("Visible"=w564) -> ()  [unwired: 2 in, 2 out]
        n295 = property on="常规版/认证版" class="Enum (严格)"("Visible"=w564) -> ()  [unwired: 2 in, 2 out]
        n296 = property on="CODMn零点核查选择" class="Enum (严格)"("Visible"=w564) -> ()  [unwired: 2 in, 2 out]
        n297 = property on="低量程稀释倍数:" class="DigNum (严格)"("Visible"=w564) -> ()  [unwired: 2 in, 2 out]
        n298 = property on="稀释倍数解释" class="Str"("Visible"=w564) -> ()  [unwired: 2 in, 2 out]
        n299 = property on="高量程稀释倍数:" class="DigNum (严格)"("Visible"=w564) -> ()  [unwired: 2 in, 2 out]
        n300 = local read "常规版/认证版"() -> (w579:enum16{"常规版-酸性", "常规版-碱性", "认证版", "浮台版"})
        n301 = case shown="\"浮台版\"" w579 {
          tunnel: [T7."Enabled" ("禁用") T7."Enabled" ("禁用") T7."Disabled and Grayed Out" ("禁用") T7."Enabled" ("禁用")] -> w578
          tunnel: [i32[] [2] ("禁用项[]") i32[] [2] ("禁用项[]") i32[] [] ("禁用项[]") i32[] [2] ("禁用项[]")] -> w577
          tunnel: [w588 w593 T7."Disabled and Grayed Out" ("禁用") w604] -> w576
          tunnel: [w587 FALSE FALSE TRUE] -> w575
          tunnel: [w588 w593 T7."Disabled and Grayed Out" ("禁用") w604] -> w565
          tunnel: [w587 TRUE FALSE FALSE] -> w563
          frame "常规版-酸性", Default {
            w587 = FALSE
            w588 = T7."Enabled" ("禁用")
          }
          frame "常规版-碱性" {
            w593 = T7."Enabled" ("禁用")
          }
          frame "认证版" {
            w599 = u16 1 items=["水样测试"=1, "标样核查"=2, "零点核查"=3, "跨度核查"=4, "空白测试"=5, "平行样"=6, "加标回收"=7] ("测量模式(公式)")
            n302 = global write "CODMn断电保存全局变量.vi" "测量模式(公式)"(w599) -> ()
          }
          frame "浮台版" {
            w604 = T7."Enabled" ("禁用")
          }
        }
        n303 = control-ref of="水样："() -> (w574:refnum<vi>)
        n304 = control-ref of="蒸馏水："() -> (w573:refnum<vi>)
        n305 = control-ref of="标液："() -> (w572:refnum<vi>)
        n306 = control-ref of="零点核查样："() -> (w571:refnum<vi>)
        n307 = control-ref of="加标回收样："() -> (w570:refnum<vi>)
        n308 = local read "水样量程选择:"() -> (w581:enum16{"L", "H", "自动切换测一次", "自动切换测两次"})
        n309 = control-ref of="量程解释说明"() -> (w568:refnum<vi>)
        n310 = control-ref of="氢氧化钠："() -> (w569:refnum<vi>)
        n311 = Not Equal To 0?(x=w581) -> (x != 0?=w580:bool)
        n312 = control-ref of="进样管"() -> (w566:refnum<vi>)
        n313 = Build Array(w574, w573, w572, w571, w570, w568, w569, w566) -> (w567:refnum<vi>[])
        n314 = Select(t=T7."Enabled" ("禁用"), s=w580, f=T7."Disabled and Grayed Out" ("禁用")) -> (s? t:f=w582:T7)
        n315 = for {
          tunnel: w567 -> [w586] mode=indexing
          tunnel: w565 -> [w585]
          n316 = property class="Ctl"(reference=w586, "DisabledEnum"=w585) -> ()  [unwired: 1 in, 2 out]
        }
        n317 = property on="低切高阈值:" class="DigNum (严格)"("DisabledEnum"=w582) -> ()  [unwired: 2 in, 2 out]
        n318 = property on="高切低阈值:" class="DigNum (严格)"("DisabledEnum"=w582) -> ()  [unwired: 2 in, 2 out]
        n319 = property on="采水泵润洗时间/s:" class="DigNum (严格)"("Visible"=w575) -> ()  [unwired: 2 in, 2 out]
        n320 = property on="采水泵沉淀时间/s:" class="DigNum (严格)"("Visible"=w575) -> ()  [unwired: 2 in, 2 out]
        n321 = property on="采水泵排液时间/s:" class="DigNum (严格)"("Visible"=w575) -> ()  [unwired: 2 in, 2 out]
        n322 = property on="采水泵进样时间/s:" class="DigNum (严格)"("Visible"=w575) -> ()  [unwired: 2 in, 2 out]
        n323 = property on="一键写入" class="Bool (严格)"("DisabledEnum"=w576) -> ()  [unwired: 2 in, 2 out]
        n324 = property on="量程选择" class="Enum (严格)"("Disabled Items []"=w577) -> ()  [unwired: 2 in, 2 out]
        n325 = property on="测量模式(公式)" class="Ring (严格)"("DisabledEnum"=w578) -> ()  [unwired: 2 in, 2 out]
        n326 = property on="氢氧化钠：" class="DigNum (严格)"("Visible"=w563) -> ()  [unwired: 2 in, 2 out]
        n327 = property on="氢氧化钠" class="DigNum (严格)"("Visible"=w563) -> ()  [unwired: 2 in, 2 out]
      }
    }
    n328 = flat-sequence {
      frame #0 {
        # "公式读取显示（只在读取公式的时候改变一次）"
        n329 = global read "COD内部交互全局.vi" "读取公式显示"() -> (w321:bool)
        n330 = case shown="真" w321 {
          frame False {
          }
          frame True {
            n331 = global write "COD内部交互全局.vi" "读取公式显示"(FALSE ("读取参数显示")) -> ()
            n332 = global read "COD内部交互全局.vi" "读取公式"() -> (w331:u16[])
            n333 = Array Subset(array=w331, index=10 ("索引"), length=84 ("长度")) -> (w326:u16[])
            n334 = One Button Dialog(message="公式读取成功！" ("消息")) -> ()  [unwired: 1 in, 1 out]
            n335 = local read "测量模式(公式)"() -> (w329:u16)
            n336 = call "浮点CDAB转换COD.vi"("数组"=w326) -> ("数组 2"=w327:sgl[])  [unwired: 10 in]
            n337 = Array To Cluster(array=w327) -> (cluster=w330:T11)
            n338 = case shown="6" w329 {
              tunnel: [cluster{"X":dbl, "b":dbl, "X^2":dbl} {"X"=999.0, "b"=999.0, "X^2"=999.0} ("方程系数") w334 w353 w372 w391 w410 w429 w448] -> w328
              tunnel: w330 -> [_ w333 w352 w371 w390 w409 w428 w447]
              frame 0, Default {
              }
              frame 1 {
                n339 = local read "量程选择"() -> (w336:enum16{"低量程", "高量程", "0-2量程"})
                n340 = case shown="\"低量程\", 默认" w336 {
                  tunnel: w333 -> [w343 w347 w351]
                  tunnel: [w342 w346 w350] -> w339
                  tunnel: [w341 w345 w349] -> w338
                  tunnel: [w340 w344 w348] -> w337
                  frame "低量程", Default {
                    n341 = Unbundle By Name(w343) -> ("数组 2[0]"=w342:sgl, "数组 2[1]"=w341:sgl, "数组 2[2]"=w340:sgl)
                  }
                  frame "高量程" {
                    n342 = Unbundle By Name(w347) -> ("数组 2[3]"=w346:sgl, "数组 2[4]"=w345:sgl, "数组 2[5]"=w344:sgl)
                  }
                  frame "0-2量程" {
                    n343 = Unbundle By Name(w351) -> ("数组 2[6]"=w350:sgl, "数组 2[7]"=w349:sgl, "数组 2[8]"=w348:sgl)
                  }
                }
                n344 = Bundle By Name(cluster=cluster{"X":dbl, "b":dbl, "X^2":dbl} {"X"=0.0, "b"=0.0, "X^2"=0.0} ("方程系数"), "X"=w339, "b"=w338, "X^2"=w337) -> (w334:cluster{"X":dbl, "b":dbl, "X^2":dbl})
              }
              frame 2 {
                n345 = local read "量程选择"() -> (w355:enum16{"低量程", "高量程", "0-2量程"})
                n346 = case shown="\"高量程\"" w355 {
                  tunnel: w352 -> [w362 w366 w370]
                  tunnel: [w361 w365 w369] -> w358
                  tunnel: [w360 w364 w368] -> w357
                  tunnel: [w359 w363 w367] -> w356
                  frame "低量程", Default {
                    n347 = Unbundle By Name(w362) -> ("数组 2[6]"=w361:sgl, "数组 2[7]"=w360:sgl, "数组 2[8]"=w359:sgl)
                  }
                  frame "高量程" {
                    n348 = Unbundle By Name(w366) -> ("数组 2[9]"=w365:sgl, "数组 2[10]"=w364:sgl, "数组 2[11]"=w363:sgl)
                  }
                  frame "0-2量程" {
                    n349 = Unbundle By Name(w370) -> ("数组 2[6]"=w369:sgl, "数组 2[7]"=w368:sgl, "数组 2[8]"=w367:sgl)
                  }
                }
                n350 = Bundle By Name(cluster=cluster{"X":dbl, "b":dbl, "X^2":dbl} {"X"=0.0, "b"=0.0, "X^2"=0.0} ("方程系数"), "X"=w358, "b"=w357, "X^2"=w356) -> (w353:cluster{"X":dbl, "b":dbl, "X^2":dbl})
              }
              frame 3 {
                n351 = local read "量程选择"() -> (w374:enum16{"低量程", "高量程", "0-2量程"})
                n352 = case shown="\"高量程\"" w374 {
                  tunnel: w371 -> [w381 w385 w389]
                  tunnel: [w380 w384 w388] -> w377
                  tunnel: [w379 w383 w387] -> w376
                  tunnel: [w378 w382 w386] -> w375
                  frame "低量程", Default {
                    n353 = Unbundle By Name(w381) -> ("数组 2[12]"=w380:sgl, "数组 2[13]"=w379:sgl, "数组 2[14]"=w378:sgl)
                  }
                  frame "高量程" {
                    n354 = Unbundle By Name(w385) -> ("数组 2[15]"=w384:sgl, "数组 2[16]"=w383:sgl, "数组 2[17]"=w382:sgl)
                  }
                  frame "0-2量程" {
                    n355 = Unbundle By Name(w389) -> ("数组 2[6]"=w388:sgl, "数组 2[7]"=w387:sgl, "数组 2[8]"=w386:sgl)
                  }
                }
                n356 = Bundle By Name(cluster=cluster{"X":dbl, "b":dbl, "X^2":dbl} {"X"=0.0, "b"=0.0, "X^2"=0.0} ("方程系数"), "X"=w377, "b"=w376, "X^2"=w375) -> (w372:cluster{"X":dbl, "b":dbl, "X^2":dbl})
              }
              frame 4 {
                n357 = local read "量程选择"() -> (w393:enum16{"低量程", "高量程", "0-2量程"})
                n358 = case shown="\"高量程\"" w393 {
                  tunnel: w390 -> [w400 w404 w408]
                  tunnel: [w399 w403 w407] -> w396
                  tunnel: [w398 w402 w406] -> w395
                  tunnel: [w397 w401 w405] -> w394
                  frame "低量程", Default {
                    n359 = Unbundle By Name(w400) -> ("数组 2[18]"=w399:sgl, "数组 2[19]"=w398:sgl, "数组 2[20]"=w397:sgl)
                  }
                  frame "高量程" {
                    n360 = Unbundle By Name(w404) -> ("数组 2[21]"=w403:sgl, "数组 2[22]"=w402:sgl, "数组 2[23]"=w401:sgl)
                  }
                  frame "0-2量程" {
                    n361 = Unbundle By Name(w408) -> ("数组 2[6]"=w407:sgl, "数组 2[7]"=w406:sgl, "数组 2[8]"=w405:sgl)
                  }
                }
                n362 = Bundle By Name(cluster=cluster{"X":dbl, "b":dbl, "X^2":dbl} {"X"=0.0, "b"=0.0, "X^2"=0.0} ("方程系数"), "X"=w396, "b"=w395, "X^2"=w394) -> (w391:cluster{"X":dbl, "b":dbl, "X^2":dbl})
              }
              frame 5 {
                n363 = local read "量程选择"() -> (w412:enum16{"低量程", "高量程", "0-2量程"})
                n364 = case shown="\"高量程\"" w412 {
                  tunnel: w409 -> [w419 w423 w427]
                  tunnel: [w418 w422 w426] -> w415
                  tunnel: [w417 w421 w425] -> w414
                  tunnel: [w416 w420 w424] -> w413
                  frame "低量程", Default {
                    n365 = Unbundle By Name(w419) -> ("数组 2[24]"=w418:sgl, "数组 2[25]"=w417:sgl, "数组 2[26]"=w416:sgl)
                  }
                  frame "高量程" {
                    n366 = Unbundle By Name(w423) -> ("数组 2[27]"=w422:sgl, "数组 2[28]"=w421:sgl, "数组 2[29]"=w420:sgl)
                  }
                  frame "0-2量程" {
                    n367 = Unbundle By Name(w427) -> ("数组 2[6]"=w426:sgl, "数组 2[7]"=w425:sgl, "数组 2[8]"=w424:sgl)
                  }
                }
                n368 = Bundle By Name(cluster=cluster{"X":dbl, "b":dbl, "X^2":dbl} {"X"=0.0, "b"=0.0, "X^2"=0.0} ("方程系数"), "X"=w415, "b"=w414, "X^2"=w413) -> (w410:cluster{"X":dbl, "b":dbl, "X^2":dbl})
              }
              frame 6 {
                n369 = local read "量程选择"() -> (w431:enum16{"低量程", "高量程", "0-2量程"})
                n370 = case shown="\"高量程\"" w431 {
                  tunnel: w428 -> [w438 w442 w446]
                  tunnel: [w437 w441 w445] -> w434
                  tunnel: [w436 w440 w444] -> w433
                  tunnel: [w435 w439 w443] -> w432
                  frame "低量程", Default {
                    n371 = Unbundle By Name(w438) -> ("数组 2[30]"=w437:sgl, "数组 2[31]"=w436:sgl, "数组 2[32]"=w435:sgl)
                  }
                  frame "高量程" {
                    n372 = Unbundle By Name(w442) -> ("数组 2[33]"=w441:sgl, "数组 2[34]"=w440:sgl, "数组 2[35]"=w439:sgl)
                  }
                  frame "0-2量程" {
                    n373 = Unbundle By Name(w446) -> ("数组 2[6]"=w445:sgl, "数组 2[7]"=w444:sgl, "数组 2[8]"=w443:sgl)
                  }
                }
                n374 = Bundle By Name(cluster=cluster{"X":dbl, "b":dbl, "X^2":dbl} {"X"=0.0, "b"=0.0, "X^2"=0.0} ("方程系数"), "X"=w434, "b"=w433, "X^2"=w432) -> (w429:cluster{"X":dbl, "b":dbl, "X^2":dbl})
              }
              frame 7 {
                n375 = local read "量程选择"() -> (w450:enum16{"低量程", "高量程", "0-2量程"})
                n376 = case shown="\"高量程\"" w450 {
                  tunnel: w447 -> [w457 w461 w465]
                  tunnel: [w456 w460 w464] -> w453
                  tunnel: [w455 w459 w463] -> w452
                  tunnel: [w454 w458 w462] -> w451
                  frame "低量程", Default {
                    n377 = Unbundle By Name(w457) -> ("数组 2[36]"=w456:sgl, "数组 2[37]"=w455:sgl, "数组 2[38]"=w454:sgl)
                  }
                  frame "高量程" {
                    n378 = Unbundle By Name(w461) -> ("数组 2[39]"=w460:sgl, "数组 2[40]"=w459:sgl, "数组 2[41]"=w458:sgl)
                  }
                  frame "0-2量程" {
                    n379 = Unbundle By Name(w465) -> ("数组 2[6]"=w464:sgl, "数组 2[7]"=w463:sgl, "数组 2[8]"=w462:sgl)
                  }
                }
                n380 = Bundle By Name(cluster=cluster{"X":dbl, "b":dbl, "X^2":dbl} {"X"=0.0, "b"=0.0, "X^2"=0.0} ("方程系数"), "X"=w453, "b"=w452, "X^2"=w451) -> (w448:cluster{"X":dbl, "b":dbl, "X^2":dbl})
              }
            }
            n381 = local write "方程系数"(w328) -> ()
          }
        }
      }
    }
    n382 = Wait (ms)(milliseconds to wait=u32 1000 ("等待时间（毫秒）")) -> ()  [unwired: 1 out]
  }
  n383 = while {
    tunnel: w13 -> [w617]
    tunnel: w12 -> [w616]
    tunnel: w3 -> [_]
    stop <- FALSE stop-if-true
    # "主循环界面显示"
    n384 = flat-sequence {
      frame #0 {
        # "A，B，K"
        # "CODMn读取状态"
        n385 = global read "COD内部交互全局.vi" "ORP、时间"() -> (w746:u16[])
        n386 = To Word Integer(number=w746) -> (16bit integer=w767:i16[])
        n387 = Split 1D Array(array=w767, index=3 ("索引")) -> (first subarray=w748:i16[], second subarray=w766:i16[])
        n388 = Index Array(array=w748) -> (element #1=w752:i16, element #2=w751:i16, element #3=w750:i16)  [unwired: 3 in]
        n389 = Index Array(array=w766) -> (element #1=w761:i16, element #2=w765:i16, element #3=w764:i16, element #4=w763:i16)  [unwired: 4 in]
        n390 = To Single Precision Float(number=w763) -> (single precision float=w754:sgl)
        n391 = Build Array(w752, w751, w750) -> (w749:i16[])
        n392 = To Single Precision Float(number=w761) -> (single precision float=w760:sgl)
        n393 = To Single Precision Float(number=w765) -> (single precision float=w759:sgl)
        n394 = To Single Precision Float(number=w764) -> (single precision float=w755:sgl)
        n395 = call "HexToDate.vi"("数组"=w749) -> ("DATE"=w753:timestamp[])  [unwired: 10 in]
        n396 = Number To Decimal String(number=w759) -> (decimal integer string=→"ORP-A":string)  [unwired: 1 in]
        n397 = Number To Decimal String(number=w755) -> (decimal integer string=→"ORP-B":string)  [unwired: 1 in]
        n398 = Number To Decimal String(number=w754) -> (decimal integer string=→"ORP-K":string)  [unwired: 1 in]
        n399 = Divide(x=w760, y=sgl 100.0) -> (x/y=→"COD浓度（mg/L)":sgl)
        n400 = Index Array(array=w753) -> (element=w747:timestamp)  [unwired: 1 in]
        n401 = Format Date/Time String(seconds (now)=w747) -> (date/time string=→"数据时间":string)  [unwired: 2 in]
      }
    }
    n402 = flat-sequence {
      frame #0 {
        # "测量状态显示"
        n403 = global read "COD内部交互全局.vi" "测量状态"() -> (w666:u16[])
        n404 = To Word Integer(number=w666) -> (16bit integer=w676:i16[])
        n405 = Index Array(array=w676, index #1=0 ("索引"), index #4=3 ("索引"), index #14=13 ("索引"), index #15=14 ("索引"), index #21=20 ("索引"), index #32=31 ("索引")) -> (element #1=w680:i16, element #2=w679:i16, element #3=w678:i16, element #4=w662:i16, element #5=→"模式（受控）":i16, element #6=→"进样管":i16, element #7=→"高锰酸钾":i16, element #8=→"草酸钠":i16, element #9=→"硫酸":i16, element #10=w675:i16, element #11=w695:i16, element #12=w671:i16, element #13=→"报警数字":i16, element #14=w701:i16, element #15=w686:i16, element #16=→"多列列表框":i16, element #20=→"氢氧化钠":i16, element #21=w659:i16, element #33=→"分":i16, element #34=→"秒":i16)  [unwired: 28 in, 14 out]
        "CODMn工作状态" <- w662
        n406 = global write "COD内部交互全局.vi" "基本量程实时读取"(w659) -> ()
        n407 = Build Array(w680, w679, w678) -> (w681:i16[])
        n408 = To Single Precision Float(number=w675) -> (single precision float=→"实时ORP":sgl)
        n409 = Number To Decimal String(number=w659) -> (decimal integer string=→"基本量程(显示)":string)  [unwired: 1 in]
        n410 = Equal?(x=w671, y=u16 1) -> (x = y?=→"排液标记":bool)
        n411 = Equal?(x=w671, y=u16 2) -> (x = y?=→"断电排液标记":bool)
        n412 = Divide(x=w695, y=u16 10) -> (x/y=→"温度℃":dbl)
        n413 = Divide(x=w701, y=u16 1000) -> (x/y=→"零点滴定值":dbl)
        n414 = Divide(x=w686, y=u16 1000) -> (x/y=→"标度滴定值":dbl)
        n415 = Equal?(x=w662, y=T1."水样测试" ("CODMn工作状态")) -> (x = y?=w660:bool)
        n416 = call "HexToDate.vi"("数组"=w681) -> ("DATE"=w677:timestamp[])  [unwired: 10 in]
        n417 = case shown="真" w660 {
          tunnel: w659 -> [_ w704]
          frame False {
          }
          frame True {
            n418 = global write "CODMn断电保存全局变量.vi" "水样测试量程"(w704) -> ()
          }
        }
        n419 = Index Array(array=w677) -> (element=→"仪器时间":timestamp)  [unwired: 1 in]
      }
    }
    n420 = flat-sequence {
      frame #0 {
        # "报警状态显示"
        n421 = global read "COD内部交互全局.vi" "报警点位"() -> (w719:bool[])
        n422 = Index Array(array=w719, index #1=0 ("索引")) -> (element #1=w716:bool, element #2=w715:bool, element #3=w714:bool, element #4=w713:bool, element #5=w712:bool, element #6=w711:bool, element #7=w710:bool, element #8=w709:bool, element #9=w708:bool, element #11=w707:bool, element #13=w706:bool, element #14=w705:bool)  [unwired: 13 in, 2 out]
        "ORP故障" <- w716
        "温控器故障" <- w715
        "加热故障" <- w708
        "高锰酸钾报警" <- w710
        "草酸钠报警" <- w709
        "测量错误" <- w714
        "校零错误" <- w713
        "校标错误" <- w712
        "进水样超量程" <- w711
        "排液故障" <- w707
        "60分钟超时报警" <- w706
        "进样无液体告警" <- w705
        n423 = Compound Arithmetic op=OR ("复合运算")(w716, w715, w708, w710, w709, w714, w712, w713, w711, w707, w706) -> (→"故障标记":bool)
        n424 = Bundle By Name(cluster=T12 {"ORP故障"=FALSE, "温控器故障"=FALSE, "加热故障"=FALSE, "高锰酸钾报警"=FALSE, "草酸钠报警"=FALSE, "测量错误"=FALSE, "校零错误"=FALSE, "校标错误"=FALSE, " 进水样超量程"=FALSE, "排液阀故障"=FALSE, "60分钟超时报警"=FALSE, "进样无液体报警"=FALSE} ("报警簇"), "ORP故障"=w716, "温控器故障"=w715, "加热故障"=w708, "高锰酸钾报警"=w710, "草酸钠报警"=w709, "测量错误"=w714, "校零错误"=w713, "校标错误"=w712, "进水样超量程"=w711, "排液阀故障"=w707, "60分钟超时报警"=w706, "进样无液体报警"=w705) -> (w717:T12)
        n425 = global write "COD内部交互全局.vi" "报警簇"(w717) -> ()
      }
    }
    n426 = flat-sequence {
      frame #0 {
        # "CODMn读取状态"
        n427 = global read "COD内部交互全局.vi" "温度"() -> (w743:bool[])
        n428 = global read "COD内部交互全局.vi" "M输出点"() -> (w742:bool[])
        n429 = Index Array(array=w743) -> (element=→"加热":bool)  [unwired: 1 in]
        n430 = Index Array(array=w742) -> (element #1=→"搅拌":bool, element #4=→"进水样":bool, element #5=→"进蒸馏水":bool, element #6=→"进标液":bool, element #7=→"进零点核查样":bool, element #8=→"进加标回收样":bool, element #9=→"进高锰酸钾":bool, element #10=→"进草酸钠":bool, element #11=→"进硫酸":bool)  [unwired: 11 in, 2 out]
      }
    }
    n431 = flat-sequence {
      frame #0 {
        # "工作状态显示"
        n432 = local read "CODMn工作状态"() -> (w627:T1)
        n433 = case shown="\"标样校准\"" w627 {
          tunnel: [_ u16 0 ("y") u16 1 ("y") u16 2 ("y") u16 3 ("y") u16 4 ("y") u16 6 ("y") _ u16 7 ("y") u16 8 ("y") u16 5 ("y")] -> w626
          frame "空闲", Default {
          }
          frame "水样测试" {
          }
          frame "标样核查" {
          }
          frame "零点核查" {
          }
          frame "跨度核查" {
          }
          frame "空白测试" {
          }
          frame "平行样测试" {
          }
          frame "质控样" {
          }
          frame "空白校准" {
          }
          frame "标样校准" {
          }
          frame "加标回收" {
          }
        }
        n434 = Equal?(x=w627, y=u16 8) -> (x = y?=→"校零标记":bool)
        n435 = Equal?(x=w627, y=u16 4) -> (x = y?=→"跨度核查标记":bool)
        n436 = Equal?(x=w627, y=u16 0) -> (x = y?=→"待机":bool)
        n437 = Equal?(x=w627, y=u16 3) -> (x = y?=→"零点核查标记":bool)
        n438 = Equal?(x=w627, y=u16 7) -> (x = y?=→"质控样测量":bool)
        n439 = Equal?(x=w627, y=u16 1) -> (x = y?=→"水样测量":bool)
        n440 = Equal?(x=w627, y=u16 2) -> (x = y?=→"标样核查标记":bool)
        n441 = Equal?(x=w627, y=u16 6) -> (x = y?=→"平行样测量":bool)
        n442 = Equal?(x=w627, y=u16 9) -> (x = y?=→"校标标记":bool)
        n443 = Equal?(x=w627, y=u16 5) -> (x = y?=→"空白测试标记":bool)
        n444 = Equal?(x=w627, y=u16 10) -> (x = y?=→"加标回收测量":bool)
        n445 = global write "COD内部交互全局.vi" "测量模式数字"(w626) -> ()
      }
    }
    n446 = Get Date/Time In Seconds() -> (seconds since 1Jan1904=→"系统时间":timestamp)
    n447 = First Call?() -> (First Call?: T/F=w615:bool)
    n448 = Wait (ms)(milliseconds to wait=u32 1000 ("等待时间（毫秒）")) -> ()  [unwired: 1 out]
    n449 = case shown="真" w615 {
      tunnel: w617 -> [w723 w728]
      tunnel: w616 -> [w722 w727]
      tunnel: [w723 w726] -> w613
      tunnel: [w722 w725] -> w612
      frame False {
      }
      frame True {
        n450 = Bundle By Name(cluster=cluster{"命令":string} {"命令"=""} ("元素"), "命令"="CODMn读取参数" ("名称（未命名）")) -> (w731:cluster{"命令":string})
        n451 = Enqueue Element(queue=w728, element=w731, timeout in ms (-1)=1000 ("超时毫秒(-1)"), error in (no error)=w727) -> (queue out=w726:refnum<queue>, error out=w725:errorcluster)  [unwired: 1 out]
      }
    }
    n452 = Get Queue Status(queue=w613, error in (no error)=w612) -> (queue out=w609:refnum<queue>, error out=w608:errorcluster, # elements in queue=w611:i32)  [unwired: 1 in, 5 out]
    n453 = Equal To 0?(x=w611) -> (x = 0?=w610:bool)
    n454 = case shown="真" w610 {
      tunnel: w609 -> [_ w621]
      tunnel: w608 -> [_ w620]
      frame False {
      }
      frame True {
        n455 = Bundle By Name(cluster=cluster{"命令":string} {"命令"=""} ("元素"), "命令"="CODMn读取" ("名称（未命名）")) -> (w623:cluster{"命令":string})
        n456 = Enqueue Element(queue=w621, element=w623, timeout in ms (-1)=1000 ("超时毫秒(-1)"), error in (no error)=w620) -> ()  [unwired: 3 out]
      }
    }
  }
  n457 = while {
    stop <- FALSE stop-if-true
    # "数字键盘输入"
    n458 = event shown="[23] \"泵滴定数1\": 鼠标按下" {
      selector: _ -> [_ _ _ _ _ _ _ _ _ _ _ _ _ _ _ _ _ _ _ _ _ _ _ _ _ _ _ _ _ _]
      dyn-events: _ -> [_ _ _ _ _ _ _ _ _ _ _ _ _ _ _ _ _ _ _ _ _ _ _ _ _ _ _ _ _ _]
      timeout: _ -> [_ _ _ _ _ _ _ _ _ _ _ _ _ _ _ _ _ _ _ _ _ _ _ _ _ _ _ _ _ _]
      event Timeout {
        n459 = event-data() -> ()  [unwired: 1 in, 3 out]
      }
      event "温度": Mouse Down {
        n460 = event-data() -> ()  [unwired: 1 in, 8 out]
        n461 = local read "温度"() -> (w771:dbl)
        n462 = call "数字键盘.vi"("OldNumber"=w771) -> ("NewNumber"=w770:sgl)
        n463 = local write "温度"(w770) -> ()
      }
      event "恒温时间": Mouse Down {
        n464 = event-data() -> ()  [unwired: 1 in, 8 out]
        n465 = local read "恒温时间"() -> (w772:dbl)
        n466 = call "数字键盘.vi"("OldNumber"=w772) -> ("NewNumber"=w773:sgl)
        n467 = local write "恒温时间"(w773) -> ()
      }
      event "标准液浓度": Mouse Down {
        n468 = event-data() -> ()  [unwired: 1 in, 8 out]
        n469 = local read "标准液浓度"() -> (w775:dbl)
        n470 = call "数字键盘.vi"("OldNumber"=w775) -> ("NewNumber"=w774:sgl)
        n471 = local write "标准液浓度"(w774) -> ()
      }
      event "氢氧化钠：": Mouse Down {
        n472 = event-data() -> ()  [unwired: 1 in, 8 out]
        n473 = local read "氢氧化钠："() -> (w776:dbl)
        n474 = call "数字键盘.vi"("OldNumber"=w776) -> ("NewNumber"=w777:sgl)
        n475 = local write "氢氧化钠："(w777) -> ()
      }
      event "水样：": Mouse Down {
        n476 = event-data() -> ()  [unwired: 1 in, 8 out]
        n477 = local read "水样："() -> (w778:dbl)
        n478 = call "数字键盘.vi"("OldNumber"=w778) -> ("NewNumber"=w779:sgl)
        n479 = local write "水样："(w779) -> ()
      }
      event "蒸馏水：": Mouse Down {
        n480 = event-data() -> ()  [unwired: 1 in, 8 out]
        n481 = local read "蒸馏水："() -> (w780:dbl)
        n482 = call "数字键盘.vi"("OldNumber"=w780) -> ("NewNumber"=w781:sgl)
        n483 = local write "蒸馏水："(w781) -> ()
      }
      event "标液：": Mouse Down {
        n484 = event-data() -> ()  [unwired: 1 in, 8 out]
        n485 = local read "标液："() -> (w782:dbl)
        n486 = call "数字键盘.vi"("OldNumber"=w782) -> ("NewNumber"=w783:sgl)
        n487 = local write "标液："(w783) -> ()
      }
      event "零点核查样：": Mouse Down {
        n488 = event-data() -> ()  [unwired: 1 in, 8 out]
        n489 = local read "零点核查样："() -> (w784:dbl)
        n490 = call "数字键盘.vi"("OldNumber"=w784) -> ("NewNumber"=w785:sgl)
        n491 = local write "零点核查样："(w785) -> ()
      }
      event "加标回收样：": Mouse Down {
        n492 = event-data() -> ()  [unwired: 1 in, 8 out]
        n493 = local read "加标回收样："() -> (w786:dbl)
        n494 = call "数字键盘.vi"("OldNumber"=w786) -> ("NewNumber"=w787:sgl)
        n495 = local write "加标回收样："(w787) -> ()
      }
      event "草酸钠": Mouse Down {
        n496 = event-data() -> ()  [unwired: 1 in, 8 out]
        n497 = local read "草酸钠"() -> (w788:dbl)
        n498 = call "数字键盘.vi"("OldNumber"=w788) -> ("NewNumber"=w789:sgl)
        n499 = local write "草酸钠"(w789) -> ()
      }
      event "高锰酸钾": Mouse Down {
        n500 = event-data() -> ()  [unwired: 1 in, 8 out]
        n501 = local read "高锰酸钾"() -> (w790:dbl)
        n502 = call "数字键盘.vi"("OldNumber"=w790) -> ("NewNumber"=w791:sgl)
        n503 = local write "高锰酸钾"(w791) -> ()
      }
      event "硫酸": Mouse Down {
        n504 = event-data() -> ()  [unwired: 1 in, 8 out]
        n505 = local read "硫酸"() -> (w792:dbl)
        n506 = call "数字键盘.vi"("OldNumber"=w792) -> ("NewNumber"=w793:sgl)
        n507 = local write "硫酸"(w793) -> ()
      }
      event "零点泵计量数 2": Mouse Down {
        n508 = event-data() -> ()  [unwired: 1 in, 8 out]
        n509 = local read "零点泵计量数 2"() -> (w794:dbl)
        n510 = call "数字键盘.vi"("OldNumber"=w794) -> ("NewNumber"=w795:sgl)
        n511 = local write "零点泵计量数 2"(w795) -> ()
      }
      event "标度泵计量数 2": Mouse Down {
        n512 = event-data() -> ()  [unwired: 1 in, 8 out]
        n513 = local read "标度泵计量数 2"() -> (w796:dbl)
        n514 = call "数字键盘.vi"("OldNumber"=w796) -> ("NewNumber"=w797:sgl)
        n515 = local write "标度泵计量数 2"(w797) -> ()
      }
      event "高量程稀释倍数:": Mouse Down {
        n516 = event-data() -> ()  [unwired: 1 in, 8 out]
        n517 = local read "高量程稀释倍数:"() -> (w799:i8)
        n518 = call "数字键盘.vi"("OldNumber"=w799) -> ("NewNumber"=w798:sgl)
        n519 = local write "高量程稀释倍数:"(w798) -> ()
      }
      event "低量程稀释倍数:": Mouse Down {
        n520 = event-data() -> ()  [unwired: 1 in, 8 out]
        n521 = local read "低量程稀释倍数:"() -> (w801:i8)
        n522 = call "数字键盘.vi"("OldNumber"=w801) -> ("NewNumber"=w800:sgl)
        n523 = local write "低量程稀释倍数:"(w800) -> ()
      }
      event "浓度1": Mouse Down {
        n524 = event-data() -> ()  [unwired: 1 in, 8 out]
        n525 = local read "浓度1"() -> (w803:dbl)
        n526 = call "数字键盘.vi"("OldNumber"=w803) -> ("NewNumber"=w802:sgl)
        n527 = property on="浓度1" class="DigNum (严格)"("Val(Sgnl)"=w802) -> ()  [unwired: 2 in, 2 out]
      }
      event "浓度2": Mouse Down {
        n528 = event-data() -> ()  [unwired: 1 in, 8 out]
        n529 = local read "浓度2"() -> (w805:dbl)
        n530 = call "数字键盘.vi"("OldNumber"=w805) -> ("NewNumber"=w804:sgl)
        n531 = property on="浓度2" class="DigNum (严格)"("Val(Sgnl)"=w804) -> ()  [unwired: 2 in, 2 out]
      }
      event "浓度3": Mouse Down {
        n532 = event-data() -> ()  [unwired: 1 in, 8 out]
        n533 = local read "浓度3"() -> (w807:dbl)
        n534 = call "数字键盘.vi"("OldNumber"=w807) -> ("NewNumber"=w806:sgl)
        n535 = property on="浓度3" class="DigNum (严格)"("Val(Sgnl)"=w806) -> ()  [unwired: 2 in, 2 out]
      }
      event "浓度4": Mouse Down {
        n536 = event-data() -> ()  [unwired: 1 in, 8 out]
        n537 = local read "浓度4"() -> (w809:dbl)
        n538 = call "数字键盘.vi"("OldNumber"=w809) -> ("NewNumber"=w808:sgl)
        n539 = property on="浓度4" class="DigNum (严格)"("Val(Sgnl)"=w808) -> ()  [unwired: 2 in, 2 out]
      }
      event "浓度5": Mouse Down {
        n540 = event-data() -> ()  [unwired: 1 in, 8 out]
        n541 = local read "浓度5"() -> (w811:dbl)
        n542 = call "数字键盘.vi"("OldNumber"=w811) -> ("NewNumber"=w810:sgl)
        n543 = property on="浓度5" class="DigNum (严格)"("Val(Sgnl)"=w810) -> ()  [unwired: 2 in, 2 out]
      }
      event "跨度液浓度", "零点核查浓度", "标样浓度": Mouse Down {
        n544 = event-data() -> ("CtlRef"=w815:refnum<vi>)  [unwired: 1 in, 7 out]
        n545 = property class="DigNum (严格)"(reference=w815) -> (reference out=w812:refnum<vi>, "Value"=w814:dbl)  [unwired: 1 in, 1 out]
        n546 = call "数字键盘.vi"("OldNumber"=w814) -> ("NewNumber"=w813:sgl)
        n547 = property class="DigNum (严格)"(reference=w812, "Val(Sgnl)"=w813) -> ()  [unwired: 1 in, 2 out]
      }
      event "泵滴定数1": Mouse Down {
        n548 = event-data() -> ()  [unwired: 1 in, 8 out]
        n549 = local read "泵滴定数1"() -> (w817:dbl)
        n550 = call "数字键盘.vi"("OldNumber"=w817) -> ("NewNumber"=w816:sgl)
        n551 = property on="泵滴定数1" class="DigNum (严格)"("Val(Sgnl)"=w816) -> ()  [unwired: 2 in, 2 out]
      }
      event "泵滴定数2": Mouse Down {
        n552 = event-data() -> ()  [unwired: 1 in, 8 out]
        n553 = local read "泵滴定数2"() -> (w819:dbl)
        n554 = call "数字键盘.vi"("OldNumber"=w819) -> ("NewNumber"=w818:sgl)
        n555 = property on="泵滴定数2" class="DigNum (严格)"("Val(Sgnl)"=w818) -> ()  [unwired: 2 in, 2 out]
      }
      event "泵滴定数3": Mouse Down {
        n556 = event-data() -> ()  [unwired: 1 in, 8 out]
        n557 = local read "泵滴定数3"() -> (w821:dbl)
        n558 = call "数字键盘.vi"("OldNumber"=w821) -> ("NewNumber"=w820:sgl)
        n559 = property on="泵滴定数3" class="DigNum (严格)"("Val(Sgnl)"=w820) -> ()  [unwired: 2 in, 2 out]
      }
      event "泵滴定数4": Mouse Down {
        n560 = event-data() -> ()  [unwired: 1 in, 8 out]
        n561 = local read "泵滴定数4"() -> (w823:dbl)
        n562 = call "数字键盘.vi"("OldNumber"=w823) -> ("NewNumber"=w822:sgl)
        n563 = property on="泵滴定数4" class="DigNum (严格)"("Val(Sgnl)"=w822) -> ()  [unwired: 2 in, 2 out]
      }
      event "泵滴定数5": Mouse Down {
        n564 = event-data() -> ()  [unwired: 1 in, 8 out]
        n565 = local read "泵滴定数5"() -> (w825:dbl)
        n566 = call "数字键盘.vi"("OldNumber"=w825) -> ("NewNumber"=w824:sgl)
        n567 = property on="泵滴定数5" class="DigNum (严格)"("Val(Sgnl)"=w824) -> ()  [unwired: 2 in, 2 out]
      }
      event "低切高阈值:", "高切低阈值:": Mouse Down {
        n568 = event-data() -> ("CtlRef"=w829:refnum<vi>)  [unwired: 1 in, 7 out]
        n569 = property class="DigNum (严格)"(reference=w829) -> (reference out=w828:refnum<vi>, "Value"=w827:dbl)  [unwired: 1 in, 1 out]
        n570 = call "数字键盘.vi"("OldNumber"=w827) -> ("NewNumber"=w826:sgl)
        n571 = property class="DigNum (严格)"(reference=w828, "Val(Sgnl)"=w826) -> ()  [unwired: 1 in, 2 out]
      }
      event "远程自动校准浓度": Mouse Down {
        n572 = event-data() -> ("CtlRef"=w830:refnum<vi>)  [unwired: 1 in, 7 out]
        n573 = One Button Dialog(message="请输入其中一个在拟合公式中的非零浓度，用于远程校标！" ("消息")) -> (true=w832:bool)  [unwired: 1 in]
        n574 = case shown="真" w832 {
          tunnel: w830 -> [_ w839]
          frame False {
          }
          frame True {
            n575 = property class="DigNum (严格)"(reference=w839) -> (reference out=w834:refnum<vi>, "Value"=w840:dbl)  [unwired: 1 in, 1 out]
            n576 = global read "COD内部交互全局.vi" "启用的浓度数组"() -> (w836:dbl[])
            n577 = call "数字键盘.vi"("OldNumber"=w840) -> ("NewNumber"=w833:sgl)
            n578 = Search 1D Array(1D array=w836, element=w833) -> (index of element=w837:i32)  [unwired: 1 in]
            n579 = Equal?(x=w837, y=-1) -> (x = y?=w835:bool)
            n580 = case shown="真" w835 {
              tunnel: w834 -> [w842 _]
              tunnel: w833 -> [w841 _]
              frame False {
                n581 = property class="DigNum (严格)"(reference=w842, "Val(Sgnl)"=w841) -> ()  [unwired: 1 in, 2 out]
              }
              frame True {
                n582 = One Button Dialog(message="该浓度不属于校准浓度范围，请重新输入！" ("消息")) -> ()  [unwired: 1 in, 1 out]
              }
            }
          }
        }
      }
    }
  }
  n583 = while {
    tunnel: w13 -> [w845]
    tunnel: w12 -> [w844]
    stop <- FALSE stop-if-true
    # "主线事件"
    n584 = event shown="[27] \"一键写入\": 值改变" {
      selector: _ -> [_ _ _ _ _ _ _ _ _ _ _ _ _ _ _ _ _ _ _ _ _ _ _ _ _ _ _ _ _ _ _ _ _ _ _]
      dyn-events: _ -> [_ _ _ _ _ _ _ _ _ _ _ _ _ _ _ _ _ _ _ _ _ _ _ _ _ _ _ _ _ _ _ _ _ _ _]
      timeout: _ -> [_ _ _ _ _ _ _ _ _ _ _ _ _ _ _ _ _ _ _ _ _ _ _ _ _ _ _ _ _ _ _ _ _ _ _]
      tunnel: w845 -> [_ _ _ _ _ w934 _ _ _ _ _ _ _ _ _ _ _ _ _ _ _ w1376 _ _ _ w1588 _ _ _ _ w1878 w1885 w1907 w1950 _]
      tunnel: w844 -> [_ _ _ _ _ w933 _ _ _ _ _ _ _ _ _ _ _ _ _ _ _ w1373 _ _ _ w1587 _ _ _ _ w1877 w1884 w1906 w1949 _]
      event "单步启动": Value Change {
        n585 = event-data() -> ()  [unwired: 1 in, 6 out]
        n586 = call "CODMn手动控制框.vi"() -> ()  [unwired: 12 in]
      }
      event "启动": Mouse Down {
        n587 = event-data() -> ()  [unwired: 1 in, 8 out]
        n588 = global read "COD内部交互全局.vi" "基本量程实时读取"() -> (w849:enum16{"L", "H", "AUTO"})
        n589 = call "启动测量模式选择对话框.vi"("量程选择"=w849) -> ("标样浓度输出"=w847:dbl, "量程选择输出"=w848:enum16{"L", "H", "AUTO"}, "启动选择输出"=w853:u16)  [unwired: 8 in]
        n590 = Not Equal?(x=w853, y=u16 8) -> (x != y?=w850:bool)
        n591 = Not Equal?(x=w853, y=u16 7) -> (x != y?=w851:bool)
        n592 = And(x=w851, y=w850) -> (x .and. y?=w855:bool)
        n593 = case shown="真" w855 {
          tunnel: w853 -> [_ w868]
          tunnel: w848 -> [_ w859]
          tunnel: w847 -> [_ w857]
          frame False {
            n594 = One Button Dialog(message="请到校准配置里面进行校准操作！" ("消息")) -> ()  [unwired: 1 in, 1 out]
          }
          frame True {
            n595 = Not Equal?(x=w868, y=u16 9) -> (x != y?=w863:bool)
            n596 = case shown="\"AUTO\"" w859 {
              tunnel: [w869 w873 errorcluster {"status"=FALSE, "code"=0, "source"=""} ("error out")] -> w858
              frame "L", Default {
                n597 = call "CODMnMB_api.vi"("STEP"=enum16{"open", "read", "write", "close"}."write", "values"=u16[] [0], "starting address"=u16 4276) -> ("error out"=w869:errorcluster)  [unwired: 6 in, 2 out]
              }
              frame "H" {
                n598 = call "CODMnMB_api.vi"("STEP"=enum16{"open", "read", "write", "close"}."write", "values"=u16[] [1], "starting address"=u16 4276) -> ("error out"=w873:errorcluster)  [unwired: 6 in, 2 out]
              }
              frame "AUTO" {
              }
            }
            n599 = global write "CODMN外部API.vi" "手动启动CODMn"(w863) -> ()
            n600 = case shown="1" w868 {
              tunnel: [u16 4608 ("address") u16 4608 ("address") u16 4608 ("address") u16 4608 ("address") u16 4608 ("address") u16 4608 ("address") u16 4608 ("address") u16 4608 ("address") u16 4608 ("address") u16 4608 ("address")] -> w861
              tunnel: [u16 1 ("address") u16 2 ("address") u16 3 ("address") u16 4 ("address") u16 5 ("address") u16 7 ("address") u16 6 ("address") u16 8 ("address") u16 9 ("address") u16 0 ("address")] -> w865
              tunnel: w857 -> [_ w881 _ _ _ _ _ _ _ _]
              frame 0 {
              }
              frame 1 {
                n601 = property on="标样浓度" class="DigNum (严格)"("Val(Sgnl)"=w881) -> ()  [unwired: 2 in, 2 out]
              }
              frame 2 {
              }
              frame 3 {
              }
              frame 4 {
              }
              frame 5 {
              }
              frame 6 {
              }
              frame 7 {
              }
              frame 8 {
              }
              frame 9, Default {
              }
            }
            n602 = Insert Into Array(array=u16[] [] ("values"), index=0 ("索引"), new element=w865) -> (w860:u16[])
            n603 = call "CODMnMB_api.vi"("STEP"=enum16{"open", "read", "write", "close"}."write", "Error in"=w858, "values"=w860, "starting address"=w861) -> ()  [unwired: 5 in, 3 out]
          }
        }
      }
      event "停止": Value Change {
        n604 = event-data() -> ()  [unwired: 1 in, 6 out]
        n605 = Two Button Dialog(message="确认是否停止？" ("消息"), 1:"否" ("F按钮名称（“取消”）"), 2:"是" ("T按钮名称（“确定”）")) -> (T button?=w901:bool)
        n606 = case shown="真" w901 {
          frame False {
          }
          frame True {
            n607 = Obtain Notifier(name (unnamed)="CODMn" ("名称（未命名）"), notification data type=FALSE) -> (notifier out=w907:refnum<notifier>, error out=w905:errorcluster)  [unwired: 2 in, 1 out]
            n608 = Send Notification(notification=TRUE ("通知"), notifier=w907, error in (no error)=w905) -> (notifier out=w904:refnum<notifier>, error out=w903:errorcluster)
            n609 = Release Notifier(notifier=w904, error in (no error)=w903) -> ()  [unwired: 1 in, 3 out]
            n610 = call "CODMnMB_api.vi"("STEP"=enum16{"open", "read", "write", "close"}."write", "values"=u16[] [11], "starting address"=u16 4608) -> ()  [unwired: 6 in, 3 out]
          }
        }
      }
      event "手动控制": Value Change {
        n611 = event-data() -> ()  [unwired: 1 in, 6 out]
        n612 = call "数字密码键盘.vi"() -> ("NewNumber"=w913:sgl)  [unwired: 1 in]
        n613 = Equal?(x=w913, y=8.0) -> (x = y?=w914:bool)
        n614 = case shown="假" w914 {
          frame False {
            n615 = call "窗口弹出对话框(子VI).vi"("消息"="密码错误") -> ()  [unwired: 10 in, 1 out]
          }
          frame True {
          }
        }
      }
      event "锁定按钮": Mouse Down {
        n616 = event-data() -> ("CtlRef"=w919:refnum<vi>)  [unwired: 1 in, 7 out]
        n617 = property class="Bool (严格)"(reference=w919) -> ("Value"=w918:bool)  [unwired: 1 in, 2 out]
        n618 = case shown="真" w918 {
          selector: w918 -> [w920 _]
          tunnel: [w920 w924] -> w917
          frame False {
          }
          frame True {
            n619 = call "数字密码键盘.vi"() -> ("NewNumber"=w921:sgl)  [unwired: 1 in]
            n620 = Equal?(x=w921, y=23506.0) -> (x = y?=w925:bool)
            n621 = Equal?(x=w921, y=8.0) -> (x = y?=w922:bool)
            n622 = Or(x=w925, y=w922) -> (x .or. y?=w924:bool)
            n623 = case shown="假" w924 {
              selector: w924 -> [w928 _]
              frame False {
                n624 = local write "锁定按钮"(w928) -> ()
                n625 = One Button Dialog(message="密码错误!" ("消息")) -> ()  [unwired: 1 in, 1 out]
              }
              frame True {
                n626 = One Button Dialog(message="解锁成功!" ("消息")) -> ()  [unwired: 1 in, 1 out]
              }
            }
          }
        }
        "x = y?" <- w917
      }
      event "参数配置": Value Change {
        (unwired) u16 20 ("number of holding registers")
        (unwired) u16 4272 ("starting address")
        n627 = event-data() -> ()  [unwired: 1 in, 6 out]
        n628 = global read "CODMN外部API.vi" "ping"() -> (w932:bool)
        n629 = property on="窗格" class="Pane"("Origin"=T2 {"Horizontal"=0, "Vertical"=650} ("原点")) -> ()  [unwired: 2 in, 2 out]
        n630 = case shown="假" w932 {
          tunnel: [w944 w947] -> w931
          frame False {
            n631 = global read "COD内部交互全局.vi" "配置文件ini"() -> (w946:string)
            n632 = call <vilib>:"Application Directory.vi"() -> ("Application Directory"=w945:path)
            n633 = Build Path(base path=w945, name or relative path=w946) -> (appended path=w944:path)
          }
          frame True {
            n634 = global read "CODMN外部API.vi" "配置文件 path"() -> (w947:path)
          }
        }
        n635 = Bundle By Name(cluster=cluster{"命令":string} {"命令"=""} ("元素"), "命令"="CODMn读取参数" ("名称（未命名）")) -> (w935:cluster{"命令":string})
        n636 = call <vilib>:"Open Config Data.vi"("configuration file path"=w931) -> ("error out"=w941:errorcluster, "refnum"=w938:T4)  [unwired: 8 in, 1 out]
        n637 = Enqueue Element(queue=w934, element=w935, error in (no error)=w933) -> ()  [unwired: 1 in, 3 out]
        n638 = vi-ref "斯坦道CODMn.lvlib:CODMn断电保存全局变量.vi"() -> (w939:refnum<vi>)
        n639 = call <userlib>:"Read Panel from INI__ogtk.vi"("error in (no error)"=w941, "VI ref"=w939, "refnum"=w938) -> ("error out"=w942:errorcluster, "refnum out"=w940:T4)  [unwired: 7 in]
        n640 = call <vilib>:"Close Config Data.vi"("error in (no error)"=w942, "refnum"=w940) -> ("error out"=w930:errorcluster)  [unwired: 8 in, 1 out]
        n641 = call <vilib>:"Clear Errors.vi"("error in (no error)"=w930) -> ()  [unwired: 5 in, 2 out]
      }
      event "保存": Mouse Down {
        n642 = event-data() -> ()  [unwired: 1 in, 8 out]
        n643 = local read "通讯状态"() -> (w948:bool)
        n644 = Two Button Dialog(message="确定保存参数，保存参数将会替换原有参数！" ("消息")) -> (T button?=w950:bool)  [unwired: 2 in]
        n645 = case shown="真" w950 {
          tunnel: w948 -> [_ w951]
          frame False {
          }
          frame True {
            n646 = case shown="真" w951 {
              frame False {
                n647 = One Button Dialog(message="保存失败，当前无通讯！" ("消息")) -> ()  [unwired: 1 in, 1 out]
              }
              frame True {
                n648 = One Button Dialog(message="参数保存成功！" ("消息")) -> ()  [unwired: 1 in, 1 out]
                n649 = Build Array("采水泵进样时间/s:", "采水泵润洗时间/s:", "采水泵沉淀时间/s:", "采水泵排液时间/s:") -> (w954:i32[])
                n650 = call "CODMnMB_api.vi"("STEP"=enum16{"open", "read", "write", "close"}."write", "values"="保存参数", "starting address"=u16 4272) -> ("error out"=w960:errorcluster)  [unwired: 6 in, 2 out]
                n651 = call "CODMnMB_api.vi"("STEP"=enum16{"open", "read", "write", "close"}."write", "Error in"=w960, "values"=w954, "starting address"=u16 5596) -> ()  [unwired: 5 in, 3 out]
              }
            }
          }
        }
      }
      event "常规版/认证版": Value Change {
        n652 = event-data() -> ()  [unwired: 1 in, 6 out]
        n653 = flat-sequence {
          frame #0 {
            n654 = global write "CODMn断电保存全局变量.vi" "常规版/认证版"("常规版/认证版") -> ()
          }
          frame #1 {
            n655 = call "配置文件保存.vi"() -> ()  [unwired: 12 in]
          }
        }
      }
      event "校准配置": Value Change {
        w975 = "量程选择" ("section")
        n656 = event-data() -> ()  [unwired: 1 in, 6 out]
        n657 = global read "CODMN外部API.vi" "ping"() -> (w979:bool)
        n658 = property on="窗格" class="Pane"("Origin"=T2 {"Horizontal"=0, "Vertical"=1300} ("原点")) -> ()  [unwired: 2 in, 2 out]
        n659 = case shown="假" w979 {
          tunnel: [w1057 w1060] -> w978
          frame False {
            n660 = global read "COD内部交互全局.vi" "配置文件ini"() -> (w1059:string)
            n661 = call <vilib>:"Application Directory.vi"() -> ("Application Directory"=w1058:path)
            n662 = Build Path(base path=w1058, name or relative path=w1059) -> (appended path=w1057:path)
          }
          frame True {
            n663 = global read "CODMN外部API.vi" "配置文件 path"() -> (w1060:path)
          }
        }
        n664 = call <vilib>:"Open Config Data.vi"("configuration file path"=w978) -> ("error out"=w996:errorcluster, "refnum"=w997:T4)  [unwired: 8 in, 1 out]
        n665 = call-poly <vilib>:"Read Key.vi"("section"="CODMn模型选择" ("key"), "error in (no error)"=w996, "key"="线性和多项式", "refnum"=w997) -> ("error out"=w993:errorcluster, "value"=w995:i32, "refnum out"=w994:T4)  [unwired: 4 in, 1 out]
        n666 = local write "模型"(w995) -> ()
        n667 = call-poly <vilib>:"Read Key.vi"("section"="标线选择", "error in (no error)"=w993, "key"="选用水样", "refnum"=w994) -> ("error out"=w976:errorcluster, "value"=w980:i32, "refnum out"=w977:T4)  [unwired: 4 in, 1 out]
        n668 = local write "选用水样"(w980) -> ()
        n669 = case shown="0, 默认" w980 {
          tunnel: ["葡萄糖标线" ("section") "草酸钠标线" ("section")] -> w1002
          frame 0, Default {
          }
          frame 1 {
          }
        }
        n670 = call-poly <vilib>:"Read Key.vi"("section"=w975, "error in (no error)"=w976, "key"=w975, "refnum"=w977) -> ("error out"=w973:errorcluster, "value"=w972:i32, "refnum out"=w974:T4)  [unwired: 4 in, 1 out]
        n671 = local write "量程选择"(w972) -> ()
        n672 = case shown="2" w972 {
          tunnel: ["低量程" "高量程" "0-2量程"] -> w1001
          frame 0, Default {
          }
          frame 1 {
          }
          frame 2 {
          }
        }
        n673 = Concatenate Strings(w1002, w1001) -> (w1000:string)
        n674 = call-poly <vilib>:"Read Key.vi"("section"=w1000, "error in (no error)"=w973, "key"="浓度1", "refnum"=w974) -> ("error out"=w1027:errorcluster, "value"=w1025:dbl, "refnum out"=w1026:T4)  [unwired: 4 in, 1 out]
        n675 = local write "浓度1"(w1025) -> ()
        n676 = call-poly <vilib>:"Read Key.vi"("section"=w1000, "error in (no error)"=w1027, "key"="浓度2", "refnum"=w1026) -> ("error out"=w1041:errorcluster, "value"=w1028:dbl, "refnum out"=w1040:T4)  [unwired: 4 in, 1 out]
        n677 = local write "浓度2"(w1028) -> ()
        n678 = call-poly <vilib>:"Read Key.vi"("section"=w1000, "error in (no error)"=w1041, "key"="浓度3", "refnum"=w1040) -> ("error out"=w1042:errorcluster, "value"=w1030:dbl, "refnum out"=w1039:T4)  [unwired: 4 in, 1 out]
        n679 = local write "浓度3"(w1030) -> ()
        n680 = call-poly <vilib>:"Read Key.vi"("section"=w1000, "error in (no error)"=w1042, "key"="泵滴定数1", "refnum"=w1039) -> ("error out"=w1043:errorcluster, "value"=w1032:dbl, "refnum out"=w1038:T4)  [unwired: 4 in, 1 out]
        n681 = local write "泵滴定数1"(w1032) -> ()
        n682 = call-poly <vilib>:"Read Key.vi"("section"=w1000, "error in (no error)"=w1043, "key"="泵滴定数2", "refnum"=w1038) -> ("error out"=w1037:errorcluster, "value"=w1035:dbl, "refnum out"=w1044:T4)  [unwired: 4 in, 1 out]
        n683 = local write "泵滴定数2"(w1035) -> ()
        n684 = call-poly <vilib>:"Read Key.vi"("section"=w1000, "error in (no error)"=w1037, "key"="泵滴定数3", "refnum"=w1044) -> ("error out"=w1049:errorcluster, "value"=w1048:dbl, "refnum out"=w1045:T4)  [unwired: 4 in, 1 out]
        n685 = local write "泵滴定数3"(w1048) -> ()
        n686 = call-poly <vilib>:"Read Key.vi"("section"=w1000, "error in (no error)"=w1049, "key"="浓度4", "refnum"=w1045) -> ("error out"=w1050:errorcluster, "value"=w986:dbl, "refnum out"=w1046:T4)  [unwired: 4 in, 1 out]
        n687 = local write "浓度4"(w986) -> ()
        n688 = call-poly <vilib>:"Read Key.vi"("section"=w1000, "error in (no error)"=w1050, "key"="浓度5", "refnum"=w1046) -> ("error out"=w991:errorcluster, "value"=w985:dbl, "refnum out"=w992:T4)  [unwired: 4 in, 1 out]
        n689 = local write "浓度5"(w985) -> ()
        n690 = call-poly <vilib>:"Read Key.vi"("section"=w1000, "error in (no error)"=w991, "key"="泵滴定数4", "refnum"=w992) -> ("error out"=w1051:errorcluster, "value"=w984:dbl, "refnum out"=w1047:T4)  [unwired: 4 in, 1 out]
        n691 = local write "泵滴定数4"(w984) -> ()
        n692 = call-poly <vilib>:"Read Key.vi"("section"=w1000, "error in (no error)"=w1051, "key"="泵滴定数5", "refnum"=w1047) -> ("error out"=w989:errorcluster, "value"=w983:dbl, "refnum out"=w990:T4)  [unwired: 4 in, 1 out]
        n693 = local write "泵滴定数5"(w983) -> ()
        n694 = call-poly <vilib>:"Read Key.vi"("section"=w1000, "error in (no error)"=w989, "key"="当前选用的校准", "refnum"=w990) -> ("error out"=w1021:errorcluster, "refnum out"=w1022:T4)  [unwired: 4 in, 2 out]
        n695 = call-poly <vilib>:"Read Key.vi"("section"=w1000, "error in (no error)"=w1021, "key"="启用1", "refnum"=w1022) -> ("error out"=w1018:errorcluster, "value"=w1007:bool, "refnum out"=w1019:T4)  [unwired: 4 in, 1 out]
        n696 = local write "启用1"(w1007) -> ()
        n697 = call-poly <vilib>:"Read Key.vi"("section"=w1000, "error in (no error)"=w1018, "key"="启用2", "refnum"=w1019) -> ("error out"=w1016:errorcluster, "value"=w1006:bool, "refnum out"=w1017:T4)  [unwired: 4 in, 1 out]
        n698 = local write "启用2"(w1006) -> ()
        n699 = call-poly <vilib>:"Read Key.vi"("section"=w1000, "error in (no error)"=w1016, "key"="启用3", "refnum"=w1017) -> ("error out"=w1014:errorcluster, "value"=w1005:bool, "refnum out"=w1015:T4)  [unwired: 4 in, 1 out]
        n700 = local write "启用3"(w1005) -> ()
        n701 = call-poly <vilib>:"Read Key.vi"("section"=w1000, "error in (no error)"=w1014, "key"="启用4", "refnum"=w1015) -> ("error out"=w1012:errorcluster, "value"=w982:bool, "refnum out"=w1013:T4)  [unwired: 4 in, 1 out]
        n702 = local write "启用4"(w982) -> ()
        n703 = call-poly <vilib>:"Read Key.vi"("section"=w1000, "error in (no error)"=w1012, "key"="启用5", "refnum"=w1013) -> ("error out"=w987:errorcluster, "value"=w981:bool, "refnum out"=w988:T4)  [unwired: 4 in, 1 out]
        n704 = local write "启用5"(w981) -> ()
        n705 = call <vilib>:"Close Config Data.vi"("error in (no error)"=w987, "refnum"=w988) -> ("error out"=w966:errorcluster, "file path"=w967:path)  [unwired: 8 in]
        n706 = Open/Create/Replace File(file path (use dialog)=w967, error in=w966) -> (refnum out=w969:refnum<file>, error out=w968:errorcluster)  [unwired: 4 in, 1 out]
        n707 = Flush File(refnum=w969, error in=w968) -> (refnum out=w970:refnum<file>, error out=w971:errorcluster)
        n708 = Close File(refnum=w970, error in=w971) -> ()  [unwired: 2 out]
      }
      event "选用水样": Value Change {
        (unwired) "浓度6" ("key")
        n709 = event-data() -> ()  [unwired: 1 in, 6 out]
        n710 = local read "量程选择"() -> (w1094:enum16{"低量程", "高量程", "0-2量程"})
        n711 = property on="窗格" class="Pane"("Origin"=T2 {"Horizontal"=0, "Vertical"=1300} ("原点")) -> ()  [unwired: 2 in, 2 out]
        n712 = case shown="\"葡萄糖\", 默认" "选用水样" {
          tunnel: ["葡萄糖标线" ("section") "草酸钠标线" ("section")] -> w1096
          frame "葡萄糖", Default {
          }
          frame "草酸钠" {
          }
        }
        n713 = global read "CODMN外部API.vi" "ping"() -> (w1080:bool)
        n714 = case shown="\"0-2量程\"" w1094 {
          tunnel: ["低量程" "高量程" "0-2量程"] -> w1095
          frame "低量程", Default {
          }
          frame "高量程" {
          }
          frame "0-2量程" {
          }
        }
        n715 = case shown="假" w1080 {
          tunnel: [w1149 w1152] -> w1079
          frame False {
            n716 = global read "COD内部交互全局.vi" "配置文件ini"() -> (w1151:string)
            n717 = call <vilib>:"Application Directory.vi"() -> ("Application Directory"=w1150:path)
            n718 = Build Path(base path=w1150, name or relative path=w1151) -> (appended path=w1149:path)
          }
          frame True {
            n719 = global read "CODMN外部API.vi" "配置文件 path"() -> (w1152:path)
          }
        }
        n720 = Concatenate Strings(w1096, w1095) -> (w1093:string)
        n721 = call <vilib>:"Open Config Data.vi"("configuration file path"=w1079) -> ("error out"=w1075:errorcluster, "refnum"=w1076:T4)  [unwired: 8 in, 1 out]
        n722 = call-poly <vilib>:"Write Key.vi"("section"="标线选择", "error in (no error)"=w1075, "value"="选用水样", "key"="选用水样", "refnum"=w1076) -> ("error out"=w1072:errorcluster, "refnum out"=w1073:T4)  [unwired: 4 in, 1 out]
        n723 = call-poly <vilib>:"Read Key.vi"("section"=w1093, "error in (no error)"=w1072, "key"="浓度1", "refnum"=w1073) -> ("error out"=w1119:errorcluster, "value"=w1117:dbl, "refnum out"=w1118:T4)  [unwired: 4 in, 1 out]
        n724 = local write "浓度1"(w1117) -> ()
        n725 = call-poly <vilib>:"Read Key.vi"("section"=w1093, "error in (no error)"=w1119, "key"="浓度2", "refnum"=w1118) -> ("error out"=w1133:errorcluster, "value"=w1120:dbl, "refnum out"=w1132:T4)  [unwired: 4 in, 1 out]
        n726 = local write "浓度2"(w1120) -> ()
        n727 = call-poly <vilib>:"Read Key.vi"("section"=w1093, "error in (no error)"=w1133, "key"="浓度3", "refnum"=w1132) -> ("error out"=w1134:errorcluster, "value"=w1122:dbl, "refnum out"=w1131:T4)  [unwired: 4 in, 1 out]
        n728 = local write "浓度3"(w1122) -> ()
        n729 = call-poly <vilib>:"Read Key.vi"("section"=w1093, "error in (no error)"=w1134, "key"="泵滴定数1", "refnum"=w1131) -> ("error out"=w1135:errorcluster, "value"=w1124:dbl, "refnum out"=w1130:T4)  [unwired: 4 in, 1 out]
        n730 = local write "泵滴定数1"(w1124) -> ()
        n731 = call-poly <vilib>:"Read Key.vi"("section"=w1093, "error in (no error)"=w1135, "key"="泵滴定数2", "refnum"=w1130) -> ("error out"=w1129:errorcluster, "value"=w1127:dbl, "refnum out"=w1136:T4)  [unwired: 4 in, 1 out]
        n732 = local write "泵滴定数2"(w1127) -> ()
        n733 = call-poly <vilib>:"Read Key.vi"("section"=w1093, "error in (no error)"=w1129, "key"="泵滴定数3", "refnum"=w1136) -> ("error out"=w1141:errorcluster, "value"=w1140:dbl, "refnum out"=w1137:T4)  [unwired: 4 in, 1 out]
        n734 = local write "泵滴定数3"(w1140) -> ()
        n735 = call-poly <vilib>:"Read Key.vi"("section"=w1093, "error in (no error)"=w1141, "key"="浓度4", "refnum"=w1137) -> ("error out"=w1142:errorcluster, "value"=w1088:dbl, "refnum out"=w1138:T4)  [unwired: 4 in, 1 out]
        n736 = local write "浓度4"(w1088) -> ()
        n737 = call-poly <vilib>:"Read Key.vi"("section"=w1093, "error in (no error)"=w1142, "key"="浓度5", "refnum"=w1138) -> ("error out"=w1091:errorcluster, "value"=w1087:dbl, "refnum out"=w1092:T4)  [unwired: 4 in, 1 out]
        n738 = local write "浓度5"(w1087) -> ()
        n739 = call-poly <vilib>:"Read Key.vi"("section"=w1093, "error in (no error)"=w1091, "key"="泵滴定数4", "refnum"=w1092) -> ("error out"=w1143:errorcluster, "value"=w1086:dbl, "refnum out"=w1139:T4)  [unwired: 4 in, 1 out]
        n740 = local write "泵滴定数4"(w1086) -> ()
        n741 = call-poly <vilib>:"Read Key.vi"("section"=w1093, "error in (no error)"=w1143, "key"="泵滴定数5", "refnum"=w1139) -> ("error out"=w1089:errorcluster, "value"=w1085:dbl, "refnum out"=w1090:T4)  [unwired: 4 in, 1 out]
        n742 = local write "泵滴定数5"(w1085) -> ()
        n743 = call-poly <vilib>:"Read Key.vi"("section"=w1093, "error in (no error)"=w1089, "key"="当前选用的校准", "refnum"=w1090) -> ("error out"=w1113:errorcluster, "refnum out"=w1114:T4)  [unwired: 4 in, 2 out]
        n744 = call-poly <vilib>:"Read Key.vi"("section"=w1093, "error in (no error)"=w1113, "key"="启用1", "refnum"=w1114) -> ("error out"=w1110:errorcluster, "value"=w1099:bool, "refnum out"=w1111:T4)  [unwired: 4 in, 1 out]
        n745 = local write "启用1"(w1099) -> ()
        n746 = call-poly <vilib>:"Read Key.vi"("section"=w1093, "error in (no error)"=w1110, "key"="启用2", "refnum"=w1111) -> ("error out"=w1108:errorcluster, "value"=w1098:bool, "refnum out"=w1109:T4)  [unwired: 4 in, 1 out]
        n747 = local write "启用2"(w1098) -> ()
        n748 = call-poly <vilib>:"Read Key.vi"("section"=w1093, "error in (no error)"=w1108, "key"="启用3", "refnum"=w1109) -> ("error out"=w1106:errorcluster, "value"=w1097:bool, "refnum out"=w1107:T4)  [unwired: 4 in, 1 out]
        n749 = local write "启用3"(w1097) -> ()
        n750 = call-poly <vilib>:"Read Key.vi"("section"=w1093, "error in (no error)"=w1106, "key"="启用4", "refnum"=w1107) -> ("error out"=w1104:errorcluster, "value"=w1082:bool, "refnum out"=w1105:T4)  [unwired: 4 in, 1 out]
        n751 = local write "启用4"(w1082) -> ()
        n752 = call-poly <vilib>:"Read Key.vi"("section"=w1093, "error in (no error)"=w1104, "key"="启用5", "refnum"=w1105) -> ("error out"=w1083:errorcluster, "value"=w1081:bool, "refnum out"=w1084:T4)  [unwired: 4 in, 1 out]
        n753 = local write "启用5"(w1081) -> ()
        n754 = call <vilib>:"Close Config Data.vi"("error in (no error)"=w1083, "refnum"=w1084) -> ("error out"=w1066:errorcluster, "file path"=w1067:path)  [unwired: 8 in]
        n755 = Open/Create/Replace File(file path (use dialog)=w1067, error in=w1066) -> (refnum out=w1069:refnum<file>, error out=w1068:errorcluster)  [unwired: 4 in, 1 out]
        n756 = Flush File(refnum=w1069, error in=w1068) -> (refnum out=w1070:refnum<file>, error out=w1071:errorcluster)
        n757 = Close File(refnum=w1070, error in=w1071) -> ()  [unwired: 2 out]
      }
      event "量程选择": Value Change {
        w1169 = "量程选择" ("section")
        n758 = event-data() -> ()  [unwired: 1 in, 6 out]
        n759 = local read "选用水样"() -> (w1187:enum16{"葡萄糖", "草酸钠"})
        n760 = property on="窗格" class="Pane"("Origin"=T2 {"Horizontal"=0, "Vertical"=1300} ("原点")) -> ()  [unwired: 2 in, 2 out]
        n761 = case shown="\"葡萄糖\", 默认" w1187 {
          tunnel: ["葡萄糖标线" ("section") "草酸钠标线" ("section")] -> w1186
          frame "葡萄糖", Default {
          }
          frame "草酸钠" {
          }
        }
        n762 = case shown="\"0-2量程\"" "量程选择" {
          tunnel: ["低量程" "高量程" "0-2量程"] -> w1184
          frame "低量程", Default {
          }
          frame "高量程" {
          }
          frame "0-2量程" {
          }
        }
        n763 = global read "CODMN外部API.vi" "ping"() -> (w1171:bool)
        n764 = case shown="假" w1171 {
          tunnel: [w1240 w1243] -> w1170
          frame False {
            n765 = global read "COD内部交互全局.vi" "配置文件ini"() -> (w1242:string)
            n766 = call <vilib>:"Application Directory.vi"() -> ("Application Directory"=w1241:path)
            n767 = Build Path(base path=w1241, name or relative path=w1242) -> (appended path=w1240:path)
          }
          frame True {
            n768 = global read "CODMN外部API.vi" "配置文件 path"() -> (w1243:path)
          }
        }
        n769 = Concatenate Strings(w1186, w1184) -> (w1185:string)
        n770 = call <vilib>:"Open Config Data.vi"("configuration file path"=w1170) -> ("error out"=w1168:errorcluster, "refnum"=w1167:T4)  [unwired: 8 in, 1 out]
        n771 = call-poly <vilib>:"Write Key.vi"("section"=w1169, "error in (no error)"=w1168, "value"="量程选择", "key"=w1169, "refnum"=w1167) -> ("error out"=w1164:errorcluster, "refnum out"=w1166:T4)  [unwired: 4 in, 1 out]
        n772 = call-poly <vilib>:"Read Key.vi"("section"=w1185, "error in (no error)"=w1164, "key"="浓度1", "refnum"=w1166) -> ("error out"=w1210:errorcluster, "value"=w1208:dbl, "refnum out"=w1209:T4)  [unwired: 4 in, 1 out]
        n773 = local write "浓度1"(w1208) -> ()
        n774 = call-poly <vilib>:"Read Key.vi"("section"=w1185, "error in (no error)"=w1210, "key"="浓度2", "refnum"=w1209) -> ("error out"=w1224:errorcluster, "value"=w1211:dbl, "refnum out"=w1223:T4)  [unwired: 4 in, 1 out]
        n775 = local write "浓度2"(w1211) -> ()
        n776 = call-poly <vilib>:"Read Key.vi"("section"=w1185, "error in (no error)"=w1224, "key"="浓度3", "refnum"=w1223) -> ("error out"=w1225:errorcluster, "value"=w1213:dbl, "refnum out"=w1222:T4)  [unwired: 4 in, 1 out]
        n777 = local write "浓度3"(w1213) -> ()
        n778 = call-poly <vilib>:"Read Key.vi"("section"=w1185, "error in (no error)"=w1225, "key"="泵滴定数1", "refnum"=w1222) -> ("error out"=w1226:errorcluster, "value"=w1215:dbl, "refnum out"=w1221:T4)  [unwired: 4 in, 1 out]
        n779 = local write "泵滴定数1"(w1215) -> ()
        n780 = call-poly <vilib>:"Read Key.vi"("section"=w1185, "error in (no error)"=w1226, "key"="泵滴定数2", "refnum"=w1221) -> ("error out"=w1220:errorcluster, "value"=w1218:dbl, "refnum out"=w1227:T4)  [unwired: 4 in, 1 out]
        n781 = local write "泵滴定数2"(w1218) -> ()
        n782 = call-poly <vilib>:"Read Key.vi"("section"=w1185, "error in (no error)"=w1220, "key"="泵滴定数3", "refnum"=w1227) -> ("error out"=w1232:errorcluster, "value"=w1231:dbl, "refnum out"=w1228:T4)  [unwired: 4 in, 1 out]
        n783 = local write "泵滴定数3"(w1231) -> ()
        n784 = call-poly <vilib>:"Read Key.vi"("section"=w1185, "error in (no error)"=w1232, "key"="浓度4", "refnum"=w1228) -> ("error out"=w1233:errorcluster, "value"=w1175:dbl, "refnum out"=w1229:T4)  [unwired: 4 in, 1 out]
        n785 = local write "浓度4"(w1175) -> ()
        n786 = call-poly <vilib>:"Read Key.vi"("section"=w1185, "error in (no error)"=w1233, "key"="浓度5", "refnum"=w1229) -> ("error out"=w1182:errorcluster, "value"=w1174:dbl, "refnum out"=w1183:T4)  [unwired: 4 in, 1 out]
        n787 = local write "浓度5"(w1174) -> ()
        n788 = call-poly <vilib>:"Read Key.vi"("section"=w1185, "error in (no error)"=w1182, "key"="泵滴定数4", "refnum"=w1183) -> ("error out"=w1234:errorcluster, "value"=w1173:dbl, "refnum out"=w1230:T4)  [unwired: 4 in, 1 out]
        n789 = local write "泵滴定数4"(w1173) -> ()
        n790 = call-poly <vilib>:"Read Key.vi"("section"=w1185, "error in (no error)"=w1234, "key"="泵滴定数5", "refnum"=w1230) -> ("error out"=w1180:errorcluster, "value"=w1172:dbl, "refnum out"=w1181:T4)  [unwired: 4 in, 1 out]
        n791 = local write "泵滴定数5"(w1172) -> ()
        n792 = call-poly <vilib>:"Read Key.vi"("section"=w1185, "error in (no error)"=w1180, "key"="当前选用的校准", "refnum"=w1181) -> ("error out"=w1204:errorcluster, "refnum out"=w1205:T4)  [unwired: 4 in, 2 out]
        n793 = call-poly <vilib>:"Read Key.vi"("section"=w1185, "error in (no error)"=w1204, "key"="启用1", "refnum"=w1205) -> ("error out"=w1201:errorcluster, "value"=w1190:bool, "refnum out"=w1202:T4)  [unwired: 4 in, 1 out]
        n794 = local write "启用1"(w1190) -> ()
        n795 = call-poly <vilib>:"Read Key.vi"("section"=w1185, "error in (no error)"=w1201, "key"="启用2", "refnum"=w1202) -> ("error out"=w1199:errorcluster, "value"=w1189:bool, "refnum out"=w1200:T4)  [unwired: 4 in, 1 out]
        n796 = local write "启用2"(w1189) -> ()
        n797 = call-poly <vilib>:"Read Key.vi"("section"=w1185, "error in (no error)"=w1199, "key"="启用3", "refnum"=w1200) -> ("error out"=w1197:errorcluster, "value"=w1188:bool, "refnum out"=w1198:T4)  [unwired: 4 in, 1 out]
        n798 = local write "启用3"(w1188) -> ()
        n799 = call-poly <vilib>:"Read Key.vi"("section"=w1185, "error in (no error)"=w1197, "key"="启用4", "refnum"=w1198) -> ("error out"=w1195:errorcluster, "value"=w1177:bool, "refnum out"=w1196:T4)  [unwired: 4 in, 1 out]
        n800 = local write "启用4"(w1177) -> ()
        n801 = call-poly <vilib>:"Read Key.vi"("section"=w1185, "error in (no error)"=w1195, "key"="启用5", "refnum"=w1196) -> ("error out"=w1178:errorcluster, "value"=w1176:bool, "refnum out"=w1179:T4)  [unwired: 4 in, 1 out]
        n802 = local write "启用5"(w1176) -> ()
        n803 = call <vilib>:"Close Config Data.vi"("error in (no error)"=w1178, "refnum"=w1179) -> ("error out"=w1158:errorcluster, "file path"=w1159:path)  [unwired: 8 in]
        n804 = Open/Create/Replace File(file path (use dialog)=w1159, error in=w1158) -> (refnum out=w1161:refnum<file>, error out=w1160:errorcluster)  [unwired: 4 in, 1 out]
        n805 = Flush File(refnum=w1161, error in=w1160) -> (refnum out=w1162:refnum<file>, error out=w1163:errorcluster)
        n806 = Close File(refnum=w1162, error in=w1163) -> ()  [unwired: 2 out]
      }
      event "返回": Value Change {
        w1270 = "CODMn" ("section")
        n807 = event-data() -> ()  [unwired: 1 in, 6 out]
        n808 = property on="窗格" class="Pane"("Origin"=T2 {"Horizontal"=0, "Vertical"=0} ("原点")) -> ()  [unwired: 2 in, 2 out]
        n809 = global read "CODMN外部API.vi" "ping"() -> (w1256:bool)
        n810 = case shown="假" w1256 {
          tunnel: [w1321 w1324] -> w1255
          frame False {
            n811 = global read "COD内部交互全局.vi" "配置文件ini"() -> (w1323:string)
            n812 = call <vilib>:"Application Directory.vi"() -> ("Application Directory"=w1322:path)
            n813 = Build Path(base path=w1322, name or relative path=w1323) -> (appended path=w1321:path)
          }
          frame True {
            n814 = global read "CODMN外部API.vi" "配置文件 path"() -> (w1324:path)
          }
        }
        n815 = call <vilib>:"Open Config Data.vi"("configuration file path"=w1255) -> ("error out"=w1319:errorcluster, "refnum"=w1320:T4)  [unwired: 8 in, 1 out]
        n816 = local read "浓度1"() -> (w1317:dbl)
        n817 = call-poly <vilib>:"Write Key.vi"("section"=w1270, "error in (no error)"=w1319, "value"=w1317, "key"="浓度1", "refnum"=w1320) -> ("error out"=w1316:errorcluster, "refnum out"=w1315:T4)  [unwired: 4 in, 1 out]
        n818 = local read "浓度2"() -> (w1301:dbl)
        n819 = call-poly <vilib>:"Write Key.vi"("section"=w1270, "error in (no error)"=w1316, "value"=w1301, "key"="浓度2", "refnum"=w1315) -> ("error out"=w1314:errorcluster, "refnum out"=w1313:T4)  [unwired: 4 in, 1 out]
        n820 = local read "浓度3"() -> (w1297:dbl)
        n821 = local read "泵滴定数1"() -> (w1295:dbl)
        n822 = call-poly <vilib>:"Write Key.vi"("section"=w1270, "error in (no error)"=w1314, "value"=w1297, "key"="浓度3", "refnum"=w1313) -> ("error out"=w1312:errorcluster, "refnum out"=w1311:T4)  [unwired: 4 in, 1 out]
        n823 = local read "泵滴定数2"() -> (w1293:dbl)
        n824 = call-poly <vilib>:"Write Key.vi"("section"=w1270, "error in (no error)"=w1312, "value"=w1295, "key"="泵滴定数1", "refnum"=w1311) -> ("error out"=w1310:errorcluster, "refnum out"=w1309:T4)  [unwired: 4 in, 1 out]
        n825 = local read "泵滴定数3"() -> (w1291:dbl)
        n826 = call-poly <vilib>:"Write Key.vi"("section"=w1270, "error in (no error)"=w1310, "value"=w1293, "key"="泵滴定数2", "refnum"=w1309) -> ("error out"=w1308:errorcluster, "refnum out"=w1307:T4)  [unwired: 4 in, 1 out]
        n827 = call-poly <vilib>:"Write Key.vi"("section"=w1270, "error in (no error)"=w1308, "value"=w1291, "key"="泵滴定数3", "refnum"=w1307) -> ("error out"=w1306:errorcluster, "refnum out"=w1305:T4)  [unwired: 4 in, 1 out]
        n828 = local read "浓度4"() -> (w1258:dbl)
        n829 = call-poly <vilib>:"Write Key.vi"("section"=w1270, "error in (no error)"=w1306, "value"=w1258, "key"="浓度4", "refnum"=w1305) -> ("error out"=w1299:errorcluster, "refnum out"=w1300:T4)  [unwired: 4 in, 1 out]
        n830 = local read "浓度5"() -> (w1257:dbl)
        n831 = local read "泵滴定数4"() -> (w1259:dbl)
        n832 = call-poly <vilib>:"Write Key.vi"("section"=w1270, "error in (no error)"=w1299, "value"=w1257, "key"="浓度5", "refnum"=w1300) -> ("error out"=w1267:errorcluster, "refnum out"=w1268:T4)  [unwired: 4 in, 1 out]
        n833 = local read "泵滴定数5"() -> (w1260:dbl)
        n834 = call-poly <vilib>:"Write Key.vi"("section"=w1270, "error in (no error)"=w1267, "value"=w1259, "key"="泵滴定数4", "refnum"=w1268) -> ("error out"=w1304:errorcluster, "refnum out"=w1303:T4)  [unwired: 4 in, 1 out]
        n835 = call-poly <vilib>:"Write Key.vi"("section"=w1270, "error in (no error)"=w1304, "value"=w1260, "key"="泵滴定数5", "refnum"=w1303) -> ("error out"=w1265:errorcluster, "refnum out"=w1266:T4)  [unwired: 4 in, 1 out]
        n836 = local read "启用1"() -> (w1279:bool)
        n837 = call-poly <vilib>:"Write Key.vi"("section"=w1270, "error in (no error)"=w1265, "value"=w1279, "key"="启用1", "refnum"=w1266) -> ("error out"=w1275:errorcluster, "refnum out"=w1278:T4)  [unwired: 4 in, 1 out]
        n838 = local read "启用2"() -> (w1276:bool)
        n839 = call-poly <vilib>:"Write Key.vi"("section"=w1270, "error in (no error)"=w1275, "value"=w1276, "key"="启用2", "refnum"=w1278) -> ("error out"=w1286:errorcluster, "refnum out"=w1285:T4)  [unwired: 4 in, 1 out]
        n840 = local read "启用3"() -> (w1274:bool)
        n841 = call-poly <vilib>:"Write Key.vi"("section"=w1270, "error in (no error)"=w1286, "value"=w1274, "key"="启用3", "refnum"=w1285) -> ("error out"=w1284:errorcluster, "refnum out"=w1283:T4)  [unwired: 4 in, 1 out]
        n842 = local read "启用4"() -> (w1262:bool)
        n843 = call-poly <vilib>:"Write Key.vi"("section"=w1270, "error in (no error)"=w1284, "value"=w1262, "key"="启用4", "refnum"=w1283) -> ("error out"=w1282:errorcluster, "refnum out"=w1281:T4)  [unwired: 4 in, 1 out]
        n844 = local read "启用5"() -> (w1261:bool)
        n845 = call-poly <vilib>:"Write Key.vi"("section"=w1270, "error in (no error)"=w1282, "value"=w1261, "key"="启用5", "refnum"=w1281) -> ("error out"=w1263:errorcluster, "refnum out"=w1264:T4)  [unwired: 4 in, 1 out]
        n846 = call <vilib>:"Close Config Data.vi"("error in (no error)"=w1263, "refnum"=w1264) -> ("error out"=w1249:errorcluster, "file path"=w1250:path)  [unwired: 8 in]
        n847 = Open/Create/Replace File(file path (use dialog)=w1250, error in=w1249) -> (refnum out=w1252:refnum<file>, error out=w1251:errorcluster)  [unwired: 4 in, 1 out]
        n848 = Flush File(refnum=w1252, error in=w1251) -> (refnum out=w1253:refnum<file>, error out=w1254:errorcluster)
        n849 = Close File(refnum=w1253, error in=w1254) -> ()  [unwired: 2 out]
      }
      event "关闭", "关闭 2", "关闭 3": Value Change {
        n850 = event-data() -> ()  [unwired: 1 in, 6 out]
        n851 = property on="窗格" class="Pane"("Origin"=T2 {"Horizontal"=0, "Vertical"=0} ("原点")) -> ()  [unwired: 2 in, 2 out]
      }
      event Application Instance Close {
        n852 = event-data() -> ()  [unwired: 1 in, 4 out]
      }
      event "时间校准": Value Change {
        n853 = event-data() -> ()  [unwired: 1 in, 6 out]
        n854 = Get Date/Time In Seconds() -> (seconds since 1Jan1904=w1334:timestamp)
        n855 = Build Array(w1334) -> (w1333:timestamp[])
        n856 = call "DateToHex.vi"("DATE"=w1333) -> ("数组"=w1331:u16[])  [unwired: 10 in]
        n857 = Insert Into Array(array=u16[] [1] ("values"), index=1 ("索引"), new element=w1331) -> (w1327:u16[])
        n858 = call "CODMnMB_api.vi"("STEP"=enum16{"open", "read", "write", "close"}."write", "values"=w1327, "starting address"=u16 4612) -> ("error out"=w1326:errorcluster)  [unwired: 6 in, 2 out]
        n859 = call <vilib>:"Clear Errors.vi"("error in (no error)"=w1326) -> ()  [unwired: 5 in, 2 out]
      }
      event "故障清除": Value Change {
        n860 = event-data() -> ()  [unwired: 1 in, 6 out]
        n861 = call "CODMnMB_api.vi"("STEP"=enum16{"open", "read", "write", "close"}."write", "values"=u16[] [1], "starting address"=u16 4611) -> ()  [unwired: 6 in, 3 out]
      }
      event "定时启动": Mouse Down {
        n862 = event-data() -> ()  [unwired: 1 in, 8 out]
        n863 = flat-sequence {
          frame #0 {
            n864 = global read "CODMn断电保存全局变量.vi" "间隔已启动次数"() -> (w1339:dbl)
            n865 = global read "CODMn断电保存全局变量.vi" "间隔设定次数"() -> (w1338:dbl)
            n866 = global read "CODMn断电保存全局变量.vi" "定时控制"() -> (w1341:T10)
            n867 = call "周期设置.vi"("间隔已启动次数"=w1339, "间隔设定启动次数"=w1338, "定时控制输入"=w1341) -> ("定时控制输出"=w1340:T13)  [unwired: 8 in]
            n868 = global write "CODMn断电保存全局变量.vi" "定时控制"(w1340) -> ()
          }
          frame #1 {
            n869 = call "配置文件保存.vi"() -> ()  [unwired: 12 in]
          }
        }
      }
      event "仪器参数": Value Change {
        n870 = event-data() -> ()  [unwired: 1 in, 6 out]
        n871 = global read "CODMn断电保存全局变量.vi" "CODMn仪器参数"() -> (w1342:T14)
        n872 = call "仪器参数设置.vi"("氨氮仪器参数"=w1342) -> ("仪器参数设置输出"=w1343:T15)  [unwired: 10 in]
        n873 = Unbundle By Name(w1343) -> ("确定"=w1344:bool)
        n874 = case shown="真" w1344 {
          tunnel: w1343 -> [_ w1346]
          tunnel: w1342 -> [_ w1345]
          frame False {
          }
          frame True {
            n875 = flat-sequence {
              tunnel: w1346 -> [w1363]
              tunnel: w1345 -> [w1362]
              frame #0 {
                n876 = Unbundle By Name(w1363) -> ("测量量程"=w1361:dbl, "测量精度"=w1360:dbl, "测量间隔"=w1359:dbl, "消解温度"=w1358:dbl, "消解时长"=w1357:dbl, "空白校准时间"=w1356:timestamp, "曲线截距"=w1355:dbl, "曲线斜率"=w1354:dbl, "测量检出限"=w1353:dbl, "测量信号值"=w1352:dbl, "线性相关系数"=w1351:dbl, "二次多项式系数"=w1350:dbl, "标样校准时间"=w1349:timestamp, "稀释倍数"=w1348:dbl)
                n877 = Bundle By Name(cluster=w1362, "测量量程"=w1361, "测量精度"=w1360, "测量间隔"=w1359, "消解温度"=w1358, "消解时长"=w1357, "空白校准时间"=w1356, "曲线截距"=w1355, "曲线斜率"=w1354, "测量检出限"=w1353, "测量信号值"=w1352, "线性相关系数"=w1351, "二次多项式系数"=w1350, "标样校准时间"=w1349, "稀释倍数"=w1348) -> (w1347:T14)
                n878 = global write "CODMn断电保存全局变量.vi" "CODMn仪器参数"(w1347) -> ()
              }
              frame #1 {
                n879 = call "配置文件保存.vi"() -> ()  [unwired: 12 in]
              }
            }
          }
        }
      }
      event "远程自动校准浓度", "远程校准量程": Value Change {
        n880 = event-data() -> ()  [unwired: 1 in, 6 out]
        n881 = flat-sequence {
          frame #0 {
            n882 = global write "CODMn断电保存全局变量.vi" "远程校准量程"("远程校准量程") -> ()
            n883 = global write "CODMn断电保存全局变量.vi" "远程自动校准浓度"("远程自动校准浓度") -> ()
          }
          frame #1 {
            n884 = call "配置文件保存.vi"() -> ()  [unwired: 12 in]
          }
        }
      }
      event "测量模式(公式)": Value Change {
        n885 = event-data() -> ()  [unwired: 1 in, 6 out]
        n886 = flat-sequence {
          frame #0 {
            n887 = global write "CODMn断电保存全局变量.vi" "测量模式(公式)"("测量模式(公式)") -> ()
          }
          frame #1 {
            n888 = call "配置文件保存.vi"() -> ()  [unwired: 12 in]
          }
        }
      }
      event "跨度量程选择", "跨度液浓度", "零点核查量程选择", "零点核查浓度", "标样浓度", "标样核查量程选择": Value Change {
        n889 = event-data() -> ()  [unwired: 1 in, 6 out]
        n890 = flat-sequence {
          frame #0 {
            n891 = global write "CODMn断电保存全局变量.vi" "标样浓度"("标样浓度") -> ()
            n892 = global write "CODMn断电保存全局变量.vi" "零点核查浓度"("零点核查浓度") -> ()
            n893 = global write "CODMn断电保存全局变量.vi" "跨度液浓度"("跨度液浓度") -> ()
            n894 = global write "CODMn断电保存全局变量.vi" "CODMn跨度量程选择"("跨度量程选择") -> ()
            n895 = global write "CODMn断电保存全局变量.vi" "标样核查量程选择"("标样核查量程选择") -> ()
            n896 = global write "CODMn断电保存全局变量.vi" "零点核查量程选择"("零点核查量程选择") -> ()
          }
          frame #1 {
            n897 = call "配置文件保存.vi"() -> ()  [unwired: 12 in]
          }
        }
      }
      event "校准1", "校准2", "校准3", "校准4", "校准5": Value Change {
        n898 = event-data() -> ()  [unwired: 1 in, 6 out]
        n899 = flat-sequence {
          tunnel: w1376 -> [w1385]
          tunnel: [w1385] -> w1378
          tunnel: w1373 -> [w1384]
          tunnel: [w1384] -> w1375
          tunnel: w1378 -> [w1421]
          tunnel: [w1421] -> w1377
          tunnel: w1375 -> [w1420]
          tunnel: [w1420] -> w1374
          tunnel: w1377 -> [w1448]
          tunnel: w1374 -> [w1447]
          frame #0 {
            n900 = Build Array("校准1", "校准2", "校准3", "校准4", "校准5") -> (w1388:bool[])
            n901 = for {
              tunnel: w1388 -> [w1403] mode=indexing
              tunnel: [w1395] -> w1379
              i -> [w1396]
              n902 = case shown="4" w1396 {
                tunnel: ["浓度1" "浓度2" "浓度3" "浓度4" "浓度5"] -> w1399
                frame 0, Default {
                }
                frame 1 {
                }
                frame 2 {
                }
                frame 3 {
                }
                frame 4 {
                }
              }
              n903 = Multiply(x=w1399, y=100.0) -> (x*y=w1397:dbl)
              n904 = Insert Into Array(array=u16[] [] ("values"), index=0 ("索引"), new element=w1397) -> (w1400:u16[])
              n905 = case shown="真" w1403 {
                tunnel: w1400 -> [_ w1412]
                tunnel: w1396 -> [_ w1414]
                tunnel: [_ w1409] -> w1395
                frame False {
                }
                frame True {
                  n906 = Increment(x=w1414) -> (x+1=w1410:i32)
                  n907 = global write "COD内部交互全局.vi" "当前校准"(w1410) -> ()
                  n908 = call "CODMnMB_api.vi"("STEP"=enum16{"open", "read", "write", "close"}."write", "values"=w1412, "starting address"=u16 4274) -> ("error out"=w1409:errorcluster)  [unwired: 6 in, 2 out]
                }
              }
            }
            n909 = local read "量程选择"() -> (w1381:enum16{"低量程", "高量程", "0-2量程"})
            n910 = case shown="\"高量程\"" w1381 {
              tunnel: [u16[] [0] ("values") u16[] [1] ("values") u16[] [0] ("values")] -> w1380
              frame "低量程", Default {
              }
              frame "高量程" {
              }
              frame "0-2量程" {
              }
            }
            n911 = call "CODMnMB_api.vi"("STEP"=enum16{"open", "read", "write", "close"}."write", "Error in"=w1379, "values"=w1380, "starting address"=u16 4276) -> ()  [unwired: 5 in, 3 out]
          }
          frame #1 {
            n912 = global read "COD内部交互全局.vi" "当前校准"() -> (w1422:i32)
            n913 = case shown="5" w1422 {
              tunnel: [w1430 w1431 w1432 w1433 w1434] -> w1418
              frame 1, Default {
                n914 = local read "浓度1"() -> (w1430:dbl)
              }
              frame 2 {
                n915 = local read "浓度2"() -> (w1431:dbl)
              }
              frame 3 {
                n916 = local read "浓度3"() -> (w1432:dbl)
              }
              frame 4 {
                n917 = local read "浓度4"() -> (w1433:dbl)
              }
              frame 5 {
                n918 = local read "浓度5"() -> (w1434:dbl)
              }
            }
            n919 = Number To Decimal String(number=w1418) -> (decimal integer string=w1417:string)  [unwired: 1 in]
            n920 = Concatenate Strings("仪器校准中!\n当前校准浓度为:", w1417, "mg/L" ("字符串")) -> (w1415:string)
            n921 = Not Equal To 0?(x=w1418) -> (x != 0?=w1426:bool)
            n922 = global write "COD内部交互全局.vi" "校准内容显示"(w1415) -> ()
            n923 = case shown="真" w1426 {
              tunnel: [u16 8 ("address") u16 9 ("address")] -> w1429
              tunnel: ["校零" ("测量模式") "校标" ("测量模式")] -> _
              frame False {
              }
              frame True {
              }
            }
            n924 = Insert Into Array(array=u16[] [] ("values"), index=0 ("索引"), new element=w1429) -> (w1423:u16[])
            n925 = call "CODMnMB_api.vi"("STEP"=enum16{"open", "read", "write", "close"}."write", "values"=w1423, "starting address"=u16 4608 ("address")) -> ()  [unwired: 6 in, 3 out]
          }
          frame #2 {
            n926 = local read "选用水样"() -> (w1456:enum16{"葡萄糖", "草酸钠"})
            n927 = global read "CODMN外部API.vi" "ping"() -> (w1446:bool)
            n928 = case shown="假" w1446 {
              tunnel: [w1464 w1467] -> w1445
              frame False {
                n929 = global read "COD内部交互全局.vi" "配置文件ini"() -> (w1466:string)
                n930 = call <vilib>:"Application Directory.vi"() -> ("Application Directory"=w1465:path)
                n931 = Build Path(base path=w1465, name or relative path=w1466) -> (appended path=w1464:path)
              }
              frame True {
                n932 = global read "CODMN外部API.vi" "配置文件 path"() -> (w1467:path)
              }
            }
            n933 = local read "量程选择"() -> (w1455:enum16{"低量程", "高量程", "0-2量程"})
            n934 = case shown="\"葡萄糖\", 默认" w1456 {
              tunnel: ["葡萄糖标线" ("section") "草酸钠标线" ("section")] -> w1457
              frame "葡萄糖", Default {
              }
              frame "草酸钠" {
              }
            }
            n935 = Bundle By Name(cluster=cluster{"命令":string} {"命令"=""} ("元素"), "命令"="CODMn读取参数" ("名称（未命名）")) -> (w1452:cluster{"命令":string})
            n936 = case shown="\"0-2量程\"" w1455 {
              tunnel: ["低量程" "高量程" "0-2量程"] -> w1458
              frame "低量程", Default {
              }
              frame "高量程" {
              }
              frame "0-2量程" {
              }
            }
            n937 = global read "COD内部交互全局.vi" "当前校准"() -> (w1453:i32)
            n938 = Enqueue Element(queue=w1448, element=w1452, timeout in ms (-1)=1000 ("超时毫秒(-1)"), error in (no error)=w1447) -> ()  [unwired: 3 out]
            n939 = Concatenate Strings(w1457, w1458) -> (w1454:string)
            n940 = call <vilib>:"Open Config Data.vi"("configuration file path"=w1445) -> ("error out"=w1462:errorcluster, "refnum"=w1463:T4)  [unwired: 8 in, 1 out]
            n941 = call-poly <vilib>:"Write Key.vi"("section"=w1454, "error in (no error)"=w1462, "value"=w1453, "key"="当前选用的校准" ("section"), "refnum"=w1463) -> ("error out"=w1459:errorcluster, "refnum out"=w1460:T4)  [unwired: 4 in, 1 out]
            n942 = call <vilib>:"Close Config Data.vi"("error in (no error)"=w1459, "refnum"=w1460) -> ("error out"=w1439:errorcluster, "file path"=w1440:path)  [unwired: 8 in]
            n943 = Open/Create/Replace File(file path (use dialog)=w1440, error in=w1439) -> (refnum out=w1442:refnum<file>, error out=w1441:errorcluster)  [unwired: 4 in, 1 out]
            n944 = Flush File(refnum=w1442, error in=w1441) -> (refnum out=w1443:refnum<file>, error out=w1444:errorcluster)
            n945 = Close File(refnum=w1443, error in=w1444) -> ()  [unwired: 2 out]
          }
        }
      }
      event "水样量程选择:", "低切高阈值:", "高切低阈值:": Value Change {
        n946 = event-data() -> ()  [unwired: 1 in, 6 out]
        n947 = flat-sequence {
          frame #0 {
            n948 = global write "CODMn断电保存全局变量.vi" "高切低阈值:"("高切低阈值:") -> ()
            n949 = global write "CODMn断电保存全局变量.vi" "自动切换量程:"("水样量程选择:") -> ()
            n950 = global write "CODMn断电保存全局变量.vi" "低切高阈值:"("低切高阈值:") -> ()
          }
          frame #1 {
            n951 = call "配置文件保存.vi"() -> ()  [unwired: 12 in]
          }
        }
      }
      event "模型": Value Change {
        n952 = event-data() -> ()  [unwired: 1 in, 6 out]
        n953 = global read "CODMN外部API.vi" "ping"() -> (w1483:bool)
        n954 = case shown="假" w1483 {
          tunnel: [w1491 w1494] -> w1482
          frame False {
            n955 = global read "COD内部交互全局.vi" "配置文件ini"() -> (w1493:string)
            n956 = call <vilib>:"Application Directory.vi"() -> ("Application Directory"=w1492:path)
            n957 = Build Path(base path=w1492, name or relative path=w1493) -> (appended path=w1491:path)
          }
          frame True {
            n958 = global read "CODMN外部API.vi" "配置文件 path"() -> (w1494:path)
          }
        }
        n959 = call <vilib>:"Open Config Data.vi"("configuration file path"=w1482) -> ("error out"=w1489:errorcluster, "refnum"=w1490:T4)  [unwired: 8 in, 1 out]
        n960 = local read "模型"() -> (w1484:enum32{"线性", "多项式"})
        n961 = call-poly <vilib>:"Write Key.vi"("section"="CODMn模型选择" ("key"), "error in (no error)"=w1489, "value"=w1484, "key"="线性和多项式", "refnum"=w1490) -> ("error out"=w1485:errorcluster, "refnum out"=w1486:T4)  [unwired: 4 in, 1 out]
        n962 = call <vilib>:"Close Config Data.vi"("error in (no error)"=w1485, "refnum"=w1486) -> ("error out"=w1476:errorcluster, "file path"=w1477:path)  [unwired: 8 in]
        n963 = Open/Create/Replace File(file path (use dialog)=w1477, error in=w1476) -> (refnum out=w1479:refnum<file>, error out=w1478:errorcluster)  [unwired: 4 in, 1 out]
        n964 = Flush File(refnum=w1479, error in=w1478) -> (refnum out=w1480:refnum<file>, error out=w1481:errorcluster)
        n965 = Close File(refnum=w1480, error in=w1481) -> ()  [unwired: 2 out]
      }
      event "浓度1", "浓度2", "浓度3", "泵滴定数1", "泵滴定数2", "泵滴定数3", "启用1", "启用2", "启用3", "浓度4", "浓度5", "泵滴定数4", "泵滴定数5", "启用4", "启用5": Value Change {
        n966 = event-data() -> ()  [unwired: 1 in, 6 out]
        n967 = local read "选用水样"() -> (w1518:enum16{"葡萄糖", "草酸钠"})
        n968 = local read "量程选择"() -> (w1517:enum16{"低量程", "高量程", "0-2量程"})
        n969 = case shown="\"葡萄糖\", 默认" w1518 {
          tunnel: ["葡萄糖标线" ("section") "草酸钠标线" ("section")] -> w1524
          frame "葡萄糖", Default {
          }
          frame "草酸钠" {
          }
        }
        n970 = case shown="\"0-2量程\"" w1517 {
          tunnel: ["低量程" "高量程" "0-2量程"] -> w1515
          frame "低量程", Default {
          }
          frame "高量程" {
          }
          frame "0-2量程" {
          }
        }
        n971 = global read "CODMN外部API.vi" "ping"() -> (w1502:bool)
        n972 = case shown="假" w1502 {
          tunnel: [w1575 w1578] -> w1501
          frame False {
            n973 = global read "COD内部交互全局.vi" "配置文件ini"() -> (w1577:string)
            n974 = call <vilib>:"Application Directory.vi"() -> ("Application Directory"=w1576:path)
            n975 = Build Path(base path=w1576, name or relative path=w1577) -> (appended path=w1575:path)
          }
          frame True {
            n976 = global read "CODMN外部API.vi" "配置文件 path"() -> (w1578:path)
          }
        }
        n977 = Concatenate Strings(w1524, w1515) -> (w1516:string)
        n978 = call <vilib>:"Open Config Data.vi"("configuration file path"=w1501) -> ("error out"=w1573:errorcluster, "refnum"=w1574:T4)  [unwired: 8 in, 1 out]
        n979 = local read "浓度1"() -> (w1571:dbl)
        n980 = call-poly <vilib>:"Write Key.vi"("section"=w1516, "error in (no error)"=w1573, "value"=w1571, "key"="浓度1", "refnum"=w1574) -> ("error out"=w1570:errorcluster, "refnum out"=w1569:T4)  [unwired: 4 in, 1 out]
        n981 = local read "浓度2"() -> (w1555:dbl)
        n982 = call-poly <vilib>:"Write Key.vi"("section"=w1516, "error in (no error)"=w1570, "value"=w1555, "key"="浓度2", "refnum"=w1569) -> ("error out"=w1568:errorcluster, "refnum out"=w1567:T4)  [unwired: 4 in, 1 out]
        n983 = local read "浓度3"() -> (w1551:dbl)
        n984 = local read "泵滴定数1"() -> (w1549:dbl)
        n985 = call-poly <vilib>:"Write Key.vi"("section"=w1516, "error in (no error)"=w1568, "value"=w1551, "key"="浓度3", "refnum"=w1567) -> ("error out"=w1566:errorcluster, "refnum out"=w1565:T4)  [unwired: 4 in, 1 out]
        n986 = local read "泵滴定数2"() -> (w1547:dbl)
        n987 = call-poly <vilib>:"Write Key.vi"("section"=w1516, "error in (no error)"=w1566, "value"=w1549, "key"="泵滴定数1", "refnum"=w1565) -> ("error out"=w1564:errorcluster, "refnum out"=w1563:T4)  [unwired: 4 in, 1 out]
        n988 = local read "泵滴定数3"() -> (w1545:dbl)
        n989 = call-poly <vilib>:"Write Key.vi"("section"=w1516, "error in (no error)"=w1564, "value"=w1547, "key"="泵滴定数2", "refnum"=w1563) -> ("error out"=w1562:errorcluster, "refnum out"=w1561:T4)  [unwired: 4 in, 1 out]
        n990 = call-poly <vilib>:"Write Key.vi"("section"=w1516, "error in (no error)"=w1562, "value"=w1545, "key"="泵滴定数3", "refnum"=w1561) -> ("error out"=w1560:errorcluster, "refnum out"=w1559:T4)  [unwired: 4 in, 1 out]
        n991 = local read "浓度4"() -> (w1514:dbl)
        n992 = call-poly <vilib>:"Write Key.vi"("section"=w1516, "error in (no error)"=w1560, "value"=w1514, "key"="浓度4", "refnum"=w1559) -> ("error out"=w1553:errorcluster, "refnum out"=w1554:T4)  [unwired: 4 in, 1 out]
        n993 = local read "浓度5"() -> (w1513:dbl)
        n994 = local read "泵滴定数4"() -> (w1510:dbl)
        n995 = call-poly <vilib>:"Write Key.vi"("section"=w1516, "error in (no error)"=w1553, "value"=w1513, "key"="浓度5", "refnum"=w1554) -> ("error out"=w1511:errorcluster, "refnum out"=w1512:T4)  [unwired: 4 in, 1 out]
        n996 = local read "泵滴定数5"() -> (w1509:dbl)
        n997 = call-poly <vilib>:"Write Key.vi"("section"=w1516, "error in (no error)"=w1511, "value"=w1510, "key"="泵滴定数4", "refnum"=w1512) -> ("error out"=w1558:errorcluster, "refnum out"=w1557:T4)  [unwired: 4 in, 1 out]
        n998 = call-poly <vilib>:"Write Key.vi"("section"=w1516, "error in (no error)"=w1558, "value"=w1509, "key"="泵滴定数5", "refnum"=w1557) -> ("error out"=w1507:errorcluster, "refnum out"=w1508:T4)  [unwired: 4 in, 1 out]
        n999 = local read "启用1"() -> (w1533:bool)
        n1000 = call-poly <vilib>:"Write Key.vi"("section"=w1516, "error in (no error)"=w1507, "value"=w1533, "key"="启用1", "refnum"=w1508) -> ("error out"=w1529:errorcluster, "refnum out"=w1532:T4)  [unwired: 4 in, 1 out]
        n1001 = local read "启用2"() -> (w1530:bool)
        n1002 = call-poly <vilib>:"Write Key.vi"("section"=w1516, "error in (no error)"=w1529, "value"=w1530, "key"="启用2", "refnum"=w1532) -> ("error out"=w1540:errorcluster, "refnum out"=w1539:T4)  [unwired: 4 in, 1 out]
        n1003 = local read "启用3"() -> (w1528:bool)
        n1004 = call-poly <vilib>:"Write Key.vi"("section"=w1516, "error in (no error)"=w1540, "value"=w1528, "key"="启用3", "refnum"=w1539) -> ("error out"=w1538:errorcluster, "refnum out"=w1537:T4)  [unwired: 4 in, 1 out]
        n1005 = local read "启用4"() -> (w1503:bool)
        n1006 = call-poly <vilib>:"Write Key.vi"("section"=w1516, "error in (no error)"=w1538, "value"=w1503, "key"="启用4", "refnum"=w1537) -> ("error out"=w1536:errorcluster, "refnum out"=w1535:T4)  [unwired: 4 in, 1 out]
        n1007 = local read "启用5"() -> (w1504:bool)
        n1008 = local read "选用水样"() -> (w1523:enum16{"葡萄糖", "草酸钠"})
        n1009 = call-poly <vilib>:"Write Key.vi"("section"=w1516, "error in (no error)"=w1536, "value"=w1504, "key"="启用5", "refnum"=w1535) -> ("error out"=w1505:errorcluster, "refnum out"=w1506:T4)  [unwired: 4 in, 1 out]
        n1010 = call-poly <vilib>:"Write Key.vi"("section"="标线选择", "error in (no error)"=w1505, "value"=w1523, "key"="选用水样", "refnum"=w1506) -> ("error out"=w1520:errorcluster, "refnum out"=w1521:T4)  [unwired: 4 in, 1 out]
        n1011 = call <vilib>:"Close Config Data.vi"("error in (no error)"=w1520, "refnum"=w1521) -> ("error out"=w1495:errorcluster, "file path"=w1496:path)  [unwired: 8 in]
        n1012 = Open/Create/Replace File(file path (use dialog)=w1496, error in=w1495) -> (refnum out=w1498:refnum<file>, error out=w1497:errorcluster)  [unwired: 4 in, 1 out]
        n1013 = Flush File(refnum=w1498, error in=w1497) -> (refnum out=w1499:refnum<file>, error out=w1500:errorcluster)
        n1014 = Close File(refnum=w1499, error in=w1500) -> ()  [unwired: 2 out]
      }
      event "读取": Value Change {
        (unwired) u16 94 ("number of holding registers")
        (unwired) u16 4616 ("starting address")
        n1015 = event-data() -> ()  [unwired: 1 in, 6 out]
        n1016 = Bundle By Name(cluster=cluster{"命令":string} {"命令"=""} ("元素"), "命令"="CODMn读取公式" ("名称（未命名）")) -> (w1584:cluster{"命令":string})
        n1017 = Enqueue Element(queue=w1588, element=w1584, error in (no error)=w1587) -> ()  [unwired: 1 in, 3 out]
      }
      event "写入": Mouse Down {
        n1018 = event-data() -> ()  [unwired: 1 in, 8 out]
        n1019 = Two Button Dialog(message="是否将上方方程系数K、B、X^2的值写入，写入会覆盖原有公式！" ("消息")) -> (T button?=w1589:bool)  [unwired: 2 in]
        n1020 = case shown="真" w1589 {
          frame False {
          }
          frame True {
            n1021 = local read "测量模式(公式)"() -> (w1592:u16)
            n1022 = local read "量程选择"() -> (w1591:enum16{"低量程", "高量程", "0-2量程"})
            n1023 = local read "模型"() -> (w1602:enum32{"线性", "多项式"})
            n1024 = case shown="\"线性\", 默认" w1602 {
              tunnel: [w1645 w1688] -> w1600
              tunnel: [w1644 w1687] -> w1599
              tunnel: w1592 -> [w1643 _]
              tunnel: w1591 -> [w1642 _]
              frame "线性", Default {
                (unwired) "线性" ("table输入")
                n1025 = case shown="1" w1643 {
                  tunnel: [u16 4626 ("starting address") w1652 w1657 w1662 w1667 w1672 w1677 w1682] -> w1645
                  tunnel: w1642 -> [_ w1651 _ _ _ _ _ _]
                  frame 0, Default {
                  }
                  frame 1 {
                    n1026 = case shown="\"低量程\", 默认" w1651 {
                      tunnel: [u16 4626 ("starting address") u16 4632 ("starting address") u16 4638 ("starting address")] -> w1652
                      frame "低量程", Default {
                      }
                      frame "高量程" {
                      }
                      frame "0-2量程" {
                      }
                    }
                  }
                  frame 2 {
                    n1027 = local read "量程选择"() -> (w1656:enum16{"低量程", "高量程", "0-2量程"})
                    n1028 = case shown="\"低量程\", 默认" w1656 {
                      tunnel: [u16 4638 ("starting address") u16 4644 ("starting address") u16 4638 ("starting address")] -> w1657
                      frame "低量程", Default {
                      }
                      frame "高量程" {
                      }
                      frame "0-2量程" {
                      }
                    }
                  }
                  frame 3 {
                    n1029 = local read "量程选择"() -> (w1661:enum16{"低量程", "高量程", "0-2量程"})
                    n1030 = case shown="\"低量程\", 默认" w1661 {
                      tunnel: [u16 4650 ("starting address") u16 4656 ("starting address") u16 4638 ("starting address")] -> w1662
                      frame "低量程", Default {
                      }
                      frame "高量程" {
                      }
                      frame "0-2量程" {
                      }
                    }
                  }
                  frame 4 {
                    n1031 = local read "量程选择"() -> (w1666:enum16{"低量程", "高量程", "0-2量程"})
                    n1032 = case shown="\"低量程\", 默认" w1666 {
                      tunnel: [u16 4662 ("starting address") u16 4668 ("starting address") u16 4638 ("starting address")] -> w1667
                      frame "低量程", Default {
                      }
                      frame "高量程" {
                      }
                      frame "0-2量程" {
                      }
                    }
                  }
                  frame 5 {
                    n1033 = local read "量程选择"() -> (w1671:enum16{"低量程", "高量程", "0-2量程"})
                    n1034 = case shown="\"低量程\", 默认" w1671 {
                      tunnel: [u16 4674 ("starting address") u16 4680 ("starting address") u16 4638 ("starting address")] -> w1672
                      frame "低量程", Default {
                      }
                      frame "高量程" {
                      }
                      frame "0-2量程" {
                      }
                    }
                  }
                  frame 6 {
                    n1035 = local read "量程选择"() -> (w1676:enum16{"低量程", "高量程", "0-2量程"})
                    n1036 = case shown="\"低量程\", 默认" w1676 {
                      tunnel: [u16 4686 ("starting address") u16 4692 ("starting address") u16 4638 ("starting address")] -> w1677
                      frame "低量程", Default {
                      }
                      frame "高量程" {
                      }
                      frame "0-2量程" {
                      }
                    }
                  }
                  frame 7 {
                    n1037 = local read "量程选择"() -> (w1681:enum16{"低量程", "高量程", "0-2量程"})
                    n1038 = case shown="\"低量程\", 默认" w1681 {
                      tunnel: [u16 4698 ("starting address") u16 4704 ("starting address") u16 4638 ("starting address")] -> w1682
                      frame "低量程", Default {
                      }
                      frame "高量程" {
                      }
                      frame "0-2量程" {
                      }
                    }
                  }
                }
                n1039 = local read "K"() -> (w1649:dbl)
                n1040 = local read "b"() -> (w1648:dbl)
                n1041 = Build Array(w1649, w1648, 0.0 ("元素")) -> (w1647:dbl[])
                n1042 = call "浮点转CDAB整形cod.vi"("浮点数"=w1647) -> ("CDAB整形输出"=w1644:u16[])  [unwired: 10 in]
              }
              frame "多项式" {
                (unwired) "多项式" ("table输入")
                # "b,k,c"
                n1043 = local read "多项式系数"() -> (w1693:dbl[])
                n1044 = local read "测量模式(公式)"() -> (w1689:u16)
                n1045 = Index Array(array=w1693) -> (element #1=w1691:dbl, element #2=w1686:dbl, element #3=w1690:dbl)  [unwired: 3 in]
                n1046 = case shown="1" w1689 {
                  tunnel: [u16 4626 ("starting address") w1696 w1701 w1706 w1711 w1716 w1721 w1726] -> w1688
                  frame 0, Default {
                  }
                  frame 1 {
                    n1047 = local read "量程选择"() -> (w1695:enum16{"低量程", "高量程", "0-2量程"})
                    n1048 = case shown="\"低量程\", 默认" w1695 {
                      tunnel: [u16 4626 ("starting address") u16 4632 ("starting address") u16 4638 ("starting address")] -> w1696
                      frame "低量程", Default {
                      }
                      frame "高量程" {
                      }
                      frame "0-2量程" {
                      }
                    }
                  }
                  frame 2 {
                    n1049 = local read "量程选择"() -> (w1700:enum16{"低量程", "高量程", "0-2量程"})
                    n1050 = case shown="\"低量程\", 默认" w1700 {
                      tunnel: [u16 4638 ("starting address") u16 4644 ("starting address") u16 4638 ("starting address")] -> w1701
                      frame "低量程", Default {
                      }
                      frame "高量程" {
                      }
                      frame "0-2量程" {
                      }
                    }
                  }
                  frame 3 {
                    n1051 = local read "量程选择"() -> (w1705:enum16{"低量程", "高量程", "0-2量程"})
                    n1052 = case shown="\"低量程\", 默认" w1705 {
                      tunnel: [u16 4650 ("starting address") u16 4656 ("starting address") u16 4638 ("starting address")] -> w1706
                      frame "低量程", Default {
                      }
                      frame "高量程" {
                      }
                      frame "0-2量程" {
                      }
                    }
                  }
                  frame 4 {
                    n1053 = local read "量程选择"() -> (w1710:enum16{"低量程", "高量程", "0-2量程"})
                    n1054 = case shown="\"低量程\", 默认" w1710 {
                      tunnel: [u16 4662 ("starting address") u16 4668 ("starting address") u16 4638 ("starting address")] -> w1711
                      frame "低量程", Default {
                      }
                      frame "高量程" {
                      }
                      frame "0-2量程" {
                      }
                    }
                  }
                  frame 5 {
                    n1055 = local read "量程选择"() -> (w1715:enum16{"低量程", "高量程", "0-2量程"})
                    n1056 = case shown="\"低量程\", 默认" w1715 {
                      tunnel: [u16 4674 ("starting address") u16 4680 ("starting address") u16 4638 ("starting address")] -> w1716
                      frame "低量程", Default {
                      }
                      frame "高量程" {
                      }
                      frame "0-2量程" {
                      }
                    }
                  }
                  frame 6 {
                    n1057 = local read "量程选择"() -> (w1720:enum16{"低量程", "高量程", "0-2量程"})
                    n1058 = case shown="\"低量程\", 默认" w1720 {
                      tunnel: [u16 4686 ("starting address") u16 4692 ("starting address") u16 4638 ("starting address")] -> w1721
                      frame "低量程", Default {
                      }
                      frame "高量程" {
                      }
                      frame "0-2量程" {
                      }
                    }
                  }
                  frame 7 {
                    n1059 = local read "量程选择"() -> (w1725:enum16{"低量程", "高量程", "0-2量程"})
                    n1060 = case shown="\"低量程\", 默认" w1725 {
                      tunnel: [u16 4698 ("starting address") u16 4704 ("starting address") u16 4638 ("starting address")] -> w1726
                      frame "低量程", Default {
                      }
                      frame "高量程" {
                      }
                      frame "0-2量程" {
                      }
                    }
                  }
                }
                n1061 = Build Array(w1686, w1691, w1690) -> (w1692:dbl[])
                n1062 = call "浮点转CDAB整形cod.vi"("浮点数"=w1692) -> ("CDAB整形输出"=w1687:u16[])  [unwired: 10 in]
              }
            }
            n1063 = local read "多项式系数"() -> (w1596:dbl[])
            n1064 = call "CODMnMB_api.vi"("STEP"=enum16{"open", "read", "write", "close"}."write", "values"=w1599, "starting address"=w1600) -> ("error out"=w1598:errorcluster)  [unwired: 6 in, 2 out]
            n1065 = Index Array(array=w1596) -> (element #1=w1595:dbl, element #2=w1594:dbl, element #3=w1593:dbl)  [unwired: 3 in]
            n1066 = case shown="无错误" w1598 {
              tunnel: ["写入成功！" "写入失败！"] -> w1597
              tunnel: w1595 -> [w1603 _]
              tunnel: w1594 -> [w1604 _]
              tunnel: w1593 -> [w1605 _]
              tunnel: w1592 -> [w1610 _]
              tunnel: w1591 -> [w1609 _]
              frame No Error {
                w1612 = u16 1 items=["水样测试"=1, "标样核查"=2, "零点核查"=3, "跨度核查"=4, "空白测试"=5, "平行样"=6, "加标回收"=7] ("测量模式(公式)")
                n1067 = Number To Fractional String(number=w1603) -> (F-format string=w1614:string)  [unwired: 3 in]
                n1068 = Number To Fractional String(number=w1604) -> (F-format string=w1615:string)  [unwired: 3 in]
                n1069 = Number To Fractional String(number=w1605) -> (F-format string=w1613:string)  [unwired: 3 in]
                n1070 = property on="模型" class="Enum (严格)"() -> ("RingText.Text"=w1625:string)  [unwired: 2 in, 2 out]
                n1071 = property on="测量模式(公式)" class="Ring (严格)"() -> ("RingText.Text"=w1624:string)  [unwired: 2 in, 2 out]
                n1072 = property on="量程选择" class="Enum (严格)"() -> ("RingText.Text"=w1623:string)  [unwired: 2 in, 2 out]
                n1073 = Concatenate Strings("变更后:" ("table输入"), "K:" ("字符串"), w1615, "B:" ("字符串"), w1614, "X^2:" ("字符串"), w1613) -> (w1616:string)
                n1074 = Concatenate Strings(w1625, w1624, w1623, "公式改变" ("日志信息")) -> (w1617:string)
                n1075 = Equal?(x=w1610, y=w1612) -> (x = y?=w1608:bool)
                n1076 = Equal?(x=w1609, y=enum16{"低量程", "高量程", "0-2量程"}."低量程" ("量程选择")) -> (x = y?=w1607:bool)
                n1077 = Compound Arithmetic op=AND ("复合运算")(w1608, w1607) -> (w1606:bool)
                n1078 = case shown="真" w1606 {
                  tunnel: w1604 -> [_ w1638]
                  tunnel: w1603 -> [_ w1637]
                  tunnel: w1605 -> [_ w1636]
                  frame False {
                  }
                  frame True {
                    n1079 = global read "CODMn断电保存全局变量.vi" "CODMn仪器参数"() -> (w1639:T14)
                    n1080 = Bundle By Name(cluster=w1639, "曲线截距"=w1637, "曲线斜率"=w1638, "二次多项式系数"=w1636) -> (w1640:T14)
                    n1081 = global write "CODMn断电保存全局变量.vi" "CODMn仪器参数"(w1640) -> ()
                  }
                }
                n1082 = Get Date/Time In Seconds() -> (seconds since 1Jan1904=w1629:timestamp)
                n1083 = Bundle(cluster=T5 {"时间标识"=timestamp(0 s since 1904-01-01), "参数"="", "日志信息"="", "流程参数"=""} ("data in"), "时间标识"=w1629, "参数"="CODMn" ("table输入"), "日志信息"=w1617, "流程参数"=w1616) -> (w1627:T5)
                n1084 = call "流程日志字段定义.vi"("table输入"="操作日志", "data in"=w1627) -> ("table输出"=w1632:string, "columns"=w1633:string[], "data out"=w1634:T6)  [unwired: 7 in]
                n1085 = call "插入数据.vi"("data"=w1634, "columns"=w1633, "database"="database3.mdb", "table"=w1632) -> ()  [unwired: 7 in, 1 out]
              }
              frame Error {
              }
            }
            n1086 = One Button Dialog(message=w1597) -> ()  [unwired: 1 in, 1 out]
          }
        }
      }
      event "一键写入": Value Change {
        n1087 = event-data() -> ()  [unwired: 1 in, 6 out]
        n1088 = Two Button Dialog(message="确认是否写入公式，写入会覆盖原有公式！" ("消息")) -> (T button?=w1730:bool)  [unwired: 2 in]
        n1089 = case shown="真" w1730 {
          frame False {
          }
          frame True {
            n1090 = local read "模型"() -> (w1734:enum32{"线性", "多项式"})
            n1091 = case shown="\"线性\", 默认" w1734 {
              tunnel: [w1765 w1816] -> w1732
              frame "线性", Default {
                n1092 = property on="测量模式(公式)" class="Ring (严格)"() -> ("NumItems"=w1766:u32)  [unwired: 2 in, 2 out]
                n1093 = for {
                  N: w1766 -> [_]
                  tunnel: [w1767] -> w1765
                  i -> [w1772]
                  n1094 = Increment(x=w1772) -> (x+1=w1771:i32)
                  n1095 = local read "K"() -> (w1776:dbl)
                  n1096 = local read "b"() -> (w1777:dbl)
                  n1097 = case shown="1" w1771 {
                    tunnel: [u16 4626 ("starting address") w1782 w1787 w1792 w1797 w1802 w1807 w1812] -> w1769
                    frame 0, Default {
                    }
                    frame 1 {
                      n1098 = local read "量程选择"() -> (w1781:enum16{"低量程", "高量程", "0-2量程"})
                      n1099 = case shown="\"低量程\", 默认" w1781 {
                        tunnel: [u16 4626 ("starting address") u16 4632 ("starting address") u16 4638 ("starting address")] -> w1782
                        frame "低量程", Default {
                        }
                        frame "高量程" {
                        }
                        frame "0-2量程" {
                        }
                      }
                    }
                    frame 2 {
                      n1100 = local read "量程选择"() -> (w1786:enum16{"低量程", "高量程", "0-2量程"})
                      n1101 = case shown="\"低量程\", 默认" w1786 {
                        tunnel: [u16 4638 ("starting address") u16 4644 ("starting address") u16 4638 ("starting address")] -> w1787
                        frame "低量程", Default {
                        }
                        frame "高量程" {
                        }
                        frame "0-2量程" {
                        }
                      }
                    }
                    frame 3 {
                      n1102 = local read "量程选择"() -> (w1791:enum16{"低量程", "高量程", "0-2量程"})
                      n1103 = case shown="\"低量程\", 默认" w1791 {
                        tunnel: [u16 4650 ("starting address") u16 4656 ("starting address") u16 4638 ("starting address")] -> w1792
                        frame "低量程", Default {
                        }
                        frame "高量程" {
                        }
                        frame "0-2量程" {
                        }
                      }
                    }
                    frame 4 {
                      n1104 = local read "量程选择"() -> (w1796:enum16{"低量程", "高量程", "0-2量程"})
                      n1105 = case shown="\"高量程\"" w1796 {
                        tunnel: [u16 4662 ("starting address") u16 4668 ("starting address") u16 4638 ("starting address")] -> w1797
                        frame "低量程", Default {
                        }
                        frame "高量程" {
                        }
                        frame "0-2量程" {
                        }
                      }
                    }
                    frame 5 {
                      n1106 = local read "量程选择"() -> (w1801:enum16{"低量程", "高量程", "0-2量程"})
                      n1107 = case shown="\"低量程\", 默认" w1801 {
                        tunnel: [u16 4674 ("starting address") u16 4680 ("starting address") u16 4638 ("starting address")] -> w1802
                        frame "低量程", Default {
                        }
                        frame "高量程" {
                        }
                        frame "0-2量程" {
                        }
                      }
                    }
                    frame 6 {
                      n1108 = local read "量程选择"() -> (w1806:enum16{"低量程", "高量程", "0-2量程"})
                      n1109 = case shown="\"低量程\", 默认" w1806 {
                        tunnel: [u16 4686 ("starting address") u16 4692 ("starting address") u16 4638 ("starting address")] -> w1807
                        frame "低量程", Default {
                        }
                        frame "高量程" {
                        }
                        frame "0-2量程" {
                        }
                      }
                    }
                    frame 7 {
                      n1110 = local read "量程选择"() -> (w1811:enum16{"低量程", "高量程", "0-2量程"})
                      n1111 = case shown="\"低量程\", 默认" w1811 {
                        tunnel: [u16 4698 ("starting address") u16 4704 ("starting address") u16 4638 ("starting address")] -> w1812
                        frame "低量程", Default {
                        }
                        frame "高量程" {
                        }
                        frame "0-2量程" {
                        }
                      }
                    }
                  }
                  n1112 = Build Array(w1776, w1777, 0.0 ("元素")) -> (w1778:dbl[])
                  n1113 = call "浮点转CDAB整形cod.vi"("浮点数"=w1778) -> ("CDAB整形输出"=w1775:u16[])  [unwired: 10 in]
                  n1114 = Insert Into Array(array=u16[] [], index=0 ("索引"), new element=w1775) -> (w1768:u16[])
                  n1115 = call "CODMnMB_api.vi"("STEP"=enum16{"open", "read", "write", "close"}."write", "values"=w1768, "starting address"=w1769) -> ("error out"=w1767:errorcluster)  [unwired: 6 in, 2 out]
                }
              }
              frame "多项式" {
                # "b,k,c"
                n1116 = property on="测量模式(公式)" class="Ring (严格)"() -> ("NumItems"=w1817:u32)  [unwired: 2 in, 2 out]
                n1117 = for {
                  N: w1817 -> [_]
                  tunnel: [w1818] -> w1816
                  i -> [w1823]
                  n1118 = Increment(x=w1823) -> (x+1=w1822:i32)
                  n1119 = local read "多项式系数"() -> (w1827:dbl[])
                  n1120 = case shown="2" w1822 {
                    tunnel: [u16 4626 ("starting address") w1834 w1839 w1844 w1849 w1854 w1859 w1864] -> w1819
                    frame 0, Default {
                    }
                    frame 1 {
                      n1121 = local read "量程选择"() -> (w1833:enum16{"低量程", "高量程", "0-2量程"})
                      n1122 = case shown="\"低量程\", 默认" w1833 {
                        tunnel: [u16 4626 ("starting address") u16 4632 ("starting address") u16 4638 ("starting address")] -> w1834
                        frame "低量程", Default {
                        }
                        frame "高量程" {
                        }
                        frame "0-2量程" {
                        }
                      }
                    }
                    frame 2 {
                      n1123 = local read "量程选择"() -> (w1838:enum16{"低量程", "高量程", "0-2量程"})
                      n1124 = case shown="\"低量程\", 默认" w1838 {
                        tunnel: [u16 4638 ("starting address") u16 4644 ("starting address") u16 4638 ("starting address")] -> w1839
                        frame "低量程", Default {
                        }
                        frame "高量程" {
                        }
                        frame "0-2量程" {
                        }
                      }
                    }
                    frame 3 {
                      n1125 = local read "量程选择"() -> (w1843:enum16{"低量程", "高量程", "0-2量程"})
                      n1126 = case shown="\"低量程\", 默认" w1843 {
                        tunnel: [u16 4650 ("starting address") u16 4656 ("starting address") u16 4638 ("starting address")] -> w1844
                        frame "低量程", Default {
                        }
                        frame "高量程" {
                        }
                        frame "0-2量程" {
                        }
                      }
                    }
                    frame 4 {
                      n1127 = local read "量程选择"() -> (w1848:enum16{"低量程", "高量程", "0-2量程"})
                      n1128 = case shown="\"低量程\", 默认" w1848 {
                        tunnel: [u16 4662 ("starting address") u16 4668 ("starting address") u16 4638 ("starting address")] -> w1849
                        frame "低量程", Default {
                        }
                        frame "高量程" {
                        }
                        frame "0-2量程" {
                        }
                      }
                    }
                    frame 5 {
                      n1129 = local read "量程选择"() -> (w1853:enum16{"低量程", "高量程", "0-2量程"})
                      n1130 = case shown="\"低量程\", 默认" w1853 {
                        tunnel: [u16 4674 ("starting address") u16 4680 ("starting address") u16 4638 ("starting address")] -> w1854
                        frame "低量程", Default {
                        }
                        frame "高量程" {
                        }
                        frame "0-2量程" {
                        }
                      }
                    }
                    frame 6 {
                      n1131 = local read "量程选择"() -> (w1858:enum16{"低量程", "高量程", "0-2量程"})
                      n1132 = case shown="\"低量程\", 默认" w1858 {
                        tunnel: [u16 4686 ("starting address") u16 4692 ("starting address") u16 4638 ("starting address")] -> w1859
                        frame "低量程", Default {
                        }
                        frame "高量程" {
                        }
                        frame "0-2量程" {
                        }
                      }
                    }
                    frame 7 {
                      n1133 = local read "量程选择"() -> (w1863:enum16{"低量程", "高量程", "0-2量程"})
                      n1134 = case shown="\"低量程\", 默认" w1863 {
                        tunnel: [u16 4698 ("starting address") u16 4704 ("starting address") u16 4638 ("starting address")] -> w1864
                        frame "低量程", Default {
                        }
                        frame "高量程" {
                        }
                        frame "0-2量程" {
                        }
                      }
                    }
                  }
                  n1135 = Index Array(array=w1827) -> (element #1=w1830:dbl, element #2=w1829:dbl, element #3=w1831:dbl)  [unwired: 3 in]
                  n1136 = Build Array(w1829, w1830, w1831) -> (w1828:dbl[])
                  n1137 = call "浮点转CDAB整形cod.vi"("浮点数"=w1828) -> ("CDAB整形输出"=w1826:u16[])  [unwired: 10 in]
                  n1138 = Insert Into Array(array=u16[] [], index=0 ("索引"), new element=w1826) -> (w1820:u16[])
                  n1139 = call "CODMnMB_api.vi"("STEP"=enum16{"open", "read", "write", "close"}."write", "values"=w1820, "starting address"=w1819) -> ("error out"=w1818:errorcluster)  [unwired: 6 in, 2 out]
                }
              }
            }
            n1140 = case shown="无错误" w1732 {
              tunnel: ["写入成功！" "写入失败！"] -> w1733
              frame No Error {
                n1141 = local read "多项式系数"() -> (w1740:dbl[])
                n1142 = Index Array(array=w1740) -> (element #1=w1737:dbl, element #2=w1736:dbl, element #3=w1735:dbl)  [unwired: 3 in]
                n1143 = Number To Fractional String(number=w1737) -> (F-format string=w1743:string)  [unwired: 3 in]
                n1144 = Number To Fractional String(number=w1736) -> (F-format string=w1744:string)  [unwired: 3 in]
                n1145 = Number To Fractional String(number=w1735) -> (F-format string=w1742:string)  [unwired: 3 in]
                n1146 = property on="模型" class="Enum (严格)"() -> ("RingText.Text"=w1753:string)  [unwired: 2 in, 2 out]
                n1147 = property on="量程选择" class="Enum (严格)"() -> ("RingText.Text"=w1752:string)  [unwired: 2 in, 2 out]
                n1148 = Concatenate Strings("变更后:" ("table输入"), "K:" ("字符串"), w1744, "B:" ("字符串"), w1743, "X^2:" ("字符串"), w1742) -> (w1745:string)
                n1149 = global read "CODMn断电保存全局变量.vi" "CODMn仪器参数"() -> (w1738:T14)
                n1150 = Concatenate Strings(w1753, "【一键写入全部模式】" ("日志信息"), w1752, "公式改变" ("日志信息")) -> (w1746:string)
                n1151 = Get Date/Time In Seconds() -> (seconds since 1Jan1904=w1757:timestamp)
                n1152 = Bundle By Name(cluster=w1738, "曲线截距"=w1737, "曲线斜率"=w1736, "二次多项式系数"=w1735) -> (w1739:T14)
                n1153 = Bundle(cluster=T5 {"时间标识"=timestamp(0 s since 1904-01-01), "参数"="", "日志信息"="", "流程参数"=""} ("data in"), "时间标识"=w1757, "参数"="CODMn" ("table输入"), "日志信息"=w1746, "流程参数"=w1745) -> (w1755:T5)
                n1154 = global write "CODMn断电保存全局变量.vi" "CODMn仪器参数"(w1739) -> ()
                n1155 = call "流程日志字段定义.vi"("table输入"="操作日志", "data in"=w1755) -> ("table输出"=w1760:string, "columns"=w1761:string[], "data out"=w1762:T6)  [unwired: 7 in]
                n1156 = call "插入数据.vi"("data"=w1762, "columns"=w1761, "database"="database3.mdb", "table"=w1760) -> ()  [unwired: 7 in, 1 out]
              }
              frame Error {
              }
            }
            n1157 = One Button Dialog(message=w1733) -> ()  [unwired: 1 in, 1 out]
          }
        }
      }
      event "滴定曲线": Value Change {
        n1158 = event-data() -> ()  [unwired: 1 in, 6 out]
        n1159 = property on="窗格" class="Pane"("Origin"=T2 {"Horizontal"=0, "Vertical"=3200} ("原点")) -> ()  [unwired: 2 in, 2 out]
      }
      event "历史波形": Value Change {
        n1160 = event-data() -> ()  [unwired: 1 in, 6 out]
        n1161 = call-poly <vilib>:"Read Waveforms from File.vi"() -> ("error out"=w1869:errorcluster, "first waveform in record"=w1870:waveform(dbl))  [unwired: 6 in, 2 out]
        n1162 = case shown="无错误" w1869 {
          tunnel: w1870 -> [w1873 _]
          frame No Error {
            n1163 = Unbundle By Name(w1873) -> ("t0"=w1871:timestamp, "Y"=w1872:dbl[])  [unwired: 2 out]
            n1164 = global write "COD内部交互全局.vi" "波形时间"(w1871) -> ()
            n1165 = global write "COD内部交互全局.vi" "ORP滴定曲线"(w1872) -> ()
            n1166 = global write "COD内部交互全局.vi" "滴定数-ORP值"(w1872) -> ()
          }
          frame Error {
            n1167 = One Button Dialog(message="打开失败" ("消息")) -> ()  [unwired: 1 in, 1 out]
          }
        }
      }
      event "释放串口": Value Change {
        n1168 = event-data() -> ()  [unwired: 1 in, 6 out]
        n1169 = Two Button Dialog(message="确认是否释放串口，释放串口将导致通信失败！" ("消息")) -> (T button?=w1875:bool)  [unwired: 2 in]
        n1170 = case shown="真" w1875 {
          tunnel: w1878 -> [_ w1880]
          tunnel: w1877 -> [_ w1879]
          frame False {
          }
          frame True {
            n1171 = Bundle By Name(cluster=cluster{"命令":string} {"命令"=""} ("元素"), "命令"="停用模块" ("名称（未命名）")) -> (w1881:cluster{"命令":string})
            n1172 = Enqueue Element(queue=w1880, element=w1881, error in (no error)=w1879) -> ()  [unwired: 1 in, 3 out]
          }
        }
      }
      event "打开串口": Value Change {
        n1173 = event-data() -> ()  [unwired: 1 in, 6 out]
        n1174 = flat-sequence {
          tunnel: w1885 -> [w1893]
          tunnel: w1884 -> [w1892]
          frame #0 {
            n1175 = global read "CODMn断电保存全局变量.vi" "VISA resource name"() -> (w1896:refnum<visa-resource-name>)
            n1176 = global read "CODMn断电保存全局变量.vi" "MB通信方式选择"() -> (w1889:enum16{"串口", "TCP"})
            n1177 = global read "CODMn断电保存全局变量.vi" "PORT"() -> (w1887:string)
            n1178 = global read "CODMn断电保存全局变量.vi" "IP"() -> (w1888:string)
            n1179 = call "串口配置.vi"("PORT"=w1887, "IP"=w1888, "MB通信方式选择"=w1889, "请选择串口:"=w1896) -> ("PORT 2"=w1890:string, "IP 2"=w1891:string, "确认 2"=w1894:bool, "VISA资源名称 2"=w1895:refnum<visa-resource-name>, "MB通信方式选择 2"=w1886:enum16{"串口", "TCP"})  [unwired: 3 in]
            n1180 = case shown="真" w1894 {
              tunnel: w1895 -> [_ w1905]
              tunnel: w1893 -> [_ w1901]
              tunnel: w1892 -> [_ w1900]
              tunnel: w1891 -> [_ w1899]
              tunnel: w1890 -> [_ w1898]
              tunnel: w1886 -> [_ w1897]
              frame False {
              }
              frame True {
                n1181 = global write "CODMn断电保存全局变量.vi" "IP"(w1899) -> ()
                n1182 = global write "CODMn断电保存全局变量.vi" "PORT"(w1898) -> ()
                n1183 = global write "CODMn断电保存全局变量.vi" "VISA resource name"(w1905) -> ()
                n1184 = global write "CODMn断电保存全局变量.vi" "MB通信方式选择"(w1897) -> ()
                n1185 = Bundle By Name(cluster=cluster{"命令":string} {"命令"=""} ("元素"), "命令"="启用模块" ("名称（未命名）")) -> (w1902:cluster{"命令":string})
                n1186 = Enqueue Element(queue=w1901, element=w1902, error in (no error)=w1900) -> ()  [unwired: 1 in, 3 out]
              }
            }
          }
          frame #1 {
            n1187 = call "配置文件保存.vi"() -> ()  [unwired: 12 in]
          }
        }
      }
      event "更新程序": Value Change {
        n1188 = event-data() -> ("CtlRef"=w1908:refnum<vi>, "NewVal"=w1909:bool)  [unwired: 1 in, 4 out]
        n1189 = case shown="真" w1909 {
          tunnel: w1908 -> [_ w1918]
          tunnel: w1907 -> [w1911 w1917]
          tunnel: w1906 -> [w1910 w1916]
          frame False {
            n1190 = Bundle By Name(cluster=cluster{"命令":string} {"命令"=""} ("元素"), "命令"="启用模块" ("名称（未命名）")) -> (w1912:cluster{"命令":string})
            n1191 = Enqueue Element(queue=w1911, element=w1912, error in (no error)=w1910) -> ()  [unwired: 1 in, 3 out]
          }
          frame True {
            n1192 = Two Button Dialog(message="警告，非专业人士请勿进行此操作！！！\n请确认是否继续？" ("消息")) -> (T button?=w1920:bool)  [unwired: 2 in]
            n1193 = case shown="真" w1920 {
              tunnel: w1918 -> [w1936 _]
              tunnel: w1917 -> [_ w1944]
              tunnel: w1916 -> [_ w1943]
              tunnel: [errorcluster {"status"=TRUE, "code"=0, "source"=""} ("error out") w1937] -> w1915
              frame False {
                n1194 = property class="Bool (严格)"(reference=w1936, "Value"=FALSE ("释放串口")) -> ()  [unwired: 1 in, 2 out]
              }
              frame True {
                n1195 = Bundle By Name(cluster=cluster{"命令":string} {"命令"=""} ("元素"), "命令"="CODMn程序更新" ("名称（未命名）")) -> (w1947:cluster{"命令":string})
                n1196 = Enqueue Element(queue=w1944, element=w1947, error in (no error)=w1943) -> (queue out=w1942:refnum<queue>, error out=w1941:errorcluster)  [unwired: 1 in, 1 out]
                n1197 = Bundle By Name(cluster=cluster{"命令":string} {"命令"=""} ("元素"), "命令"="停用模块" ("名称（未命名）")) -> (w1938:cluster{"命令":string})
                n1198 = Enqueue Element(queue=w1942, element=w1938, error in (no error)=w1941) -> (error out=w1937:errorcluster)  [unwired: 1 in, 2 out]
              }
            }
            n1199 = case shown="无错误" w1915 {
              frame No Error {
                n1200 = call "文件对话框"("start path"=path "D:/SRC") -> ("selected path"=w1923:path, "cancelled"=w1921:bool)  [unwired: 11 in, 2 out]
                n1201 = case shown="假" w1921 {
                  tunnel: w1923 -> [w1928 _]
                  frame False {
                    n1202 = Path To String(path=w1928) -> (string=w1925:string)
                    n1203 = Format Into String(format string="  - \"%s\"" ("格式字符串"), initial string="\"C:\\Program Files\\Fatek\\WinProladder\\WProlad.exe\"" ("command line"), w1925) -> (resulting string=w1926:string)  [unwired: 1 in, 1 out]
                    n1204 = call <vilib>:"System Exec.vi"("command line"=w1926) -> ("error out"=w1929:errorcluster)  [unwired: 7 in, 3 out]
                    n1205 = case shown="错误" w1929 {
                      tunnel: w1925 -> [_ w1932]
                      frame No Error {
                      }
                      frame Error {
                        n1206 = Format Into String(format string="  - \"%s\"" ("格式字符串"), initial string="\"C:\\Program Files (x86)\\Fatek\\WinProladder\\WProlad.exe\"" ("command line"), w1932) -> (resulting string=w1930:string)  [unwired: 1 in, 1 out]
                        n1207 = call <vilib>:"System Exec.vi"("command line"=w1930) -> ()  [unwired: 7 in, 4 out]
                      }
                    }
                  }
                  frame True {
                  }
                }
              }
              frame Error {
              }
            }
          }
        }
      }
      event "序列号变更": Value Change {
        n1208 = event-data() -> ()  [unwired: 1 in, 6 out]
        n1209 = local read "CODMn序列号"() -> (w1951:string)
        n1210 = call "序列号写入.vi"("序列号:"=w1951) -> ("确认 2"=w1948:bool, "序列号输出"=w1952:string)  [unwired: 9 in]
        n1211 = case shown="真" w1948 {
          tunnel: w1952 -> [_ w1958]
          tunnel: w1950 -> [_ w1954]
          tunnel: w1949 -> [_ w1953]
          frame False {
          }
          frame True {
            n1212 = global write "COD内部交互全局.vi" "序列号:"(w1958) -> ()
            n1213 = Bundle By Name(cluster=cluster{"命令":string} {"命令"=""} ("元素"), "命令"="CODMn序列号写入" ("名称（未命名）")) -> (w1955:cluster{"命令":string})
            n1214 = Enqueue Element(queue=w1954, element=w1955, error in (no error)=w1953) -> ()  [unwired: 1 in, 3 out]
          }
        }
      }
      event Timeout {
        n1215 = event-data() -> ()  [unwired: 1 in, 3 out]
      }
    }
  }
  n1216 = while {
    stop <- FALSE stop-if-true
    n1217 = global read "COD内部交互全局.vi" "待机"() -> (w1960:bool)
    n1218 = Wait (ms)(milliseconds to wait=u32 1000 ("等待时间（毫秒）")) -> ()  [unwired: 1 out]
    n1219 = case shown="假" w1960 {
      tunnel: [w1977 T7."Enabled" ("禁用")] -> w1962
      tunnel: [w1976 _] -> w1961
      frame False {
        # "运行中"
        n1220 = local read "校标标记"() -> (w1975:bool)
        n1221 = local read "校零标记"() -> (w1974:bool)
        n1222 = Or(x=w1975, y=w1974) -> (x .or. y?=w1978:bool)
        n1223 = case shown="真" w1978 {
          tunnel: [T7."Enabled" ("禁用") T7."Disabled and Grayed Out" ("禁用")] -> w1977
          tunnel: [_ TRUE] -> w1976
          frame False {
          }
          frame True {
          }
        }
      }
      frame True {
      }
    }
    n1224 = control-ref of="量程选择"() -> (w1968:refnum<vi>)
    n1225 = property on="校准内容显示" class="Str"("Visible"=w1961) -> ()  [unwired: 2 in, 2 out]
    n1226 = control-ref of="选用水样"() -> (w1969:refnum<vi>)
    n1227 = control-ref of="校准5"() -> (w1963:refnum<vi>)
    n1228 = control-ref of="校准4"() -> (w1964:refnum<vi>)
    n1229 = control-ref of="校准3"() -> (w1965:refnum<vi>)
    n1230 = control-ref of="校准2"() -> (w1966:refnum<vi>)
    n1231 = control-ref of="校准1"() -> (w1967:refnum<vi>)
    n1232 = Build Array(w1963, w1964, w1965, w1966, w1967, w1969, w1968) -> (w1970:refnum<vi>[])
    n1233 = for {
      tunnel: w1970 -> [w1973] mode=indexing
      tunnel: w1962 -> [w1972]
      n1234 = property class="Ctl"(reference=w1973, "DisabledEnum"=w1972) -> ()  [unwired: 1 in, 2 out]
    }
  }
  n1235 = while {
    stop <- FALSE stop-if-true
    # "滚动显示"
    n1236 = global read "COD内部交互全局.vi" "待机"() -> (w1983:bool)
    n1237 = case shown="假" w1983 {
      frame False {
        # "运行中"
        n1238 = global read "COD内部交互全局.vi" "校准内容显示"() -> (w1986:string)
        n1239 = while {
          shift-right: [w1988] -> _
          shift-left: w1986 -> [w1993]
          stop <- w1987 stop-if-true
          (unwired) "仪器校准中!\n当前校准浓度为:3mg/L" ("校准内容显示")
          n1240 = Wait (ms)(milliseconds to wait=u32 500 ("等待时间（毫秒）")) -> ()  [unwired: 1 out]
          n1241 = Spreadsheet String To Array(delimiter (Tab)="\n" ("分隔符(Tab)"), format string="" ("格式字符串"), spreadsheet string=w1993, array type (2D Dbl)=string[] []) -> (array=w1996:string[])
          n1242 = for {
            tunnel: w1996 -> [w2004] mode=indexing
            tunnel: [w2002] -> _ mode=indexing
            shift-right: [w2000] -> w1991
            shift-left: "" ("格式字符串") -> [w2001]
            n1243 = call "字符串移位显示.vi"("字符框大小"=36, "字符串输入"=w2004) -> ("移位后字符串"=w2002:string)  [unwired: 8 in, 1 out]
            n1244 = Concatenate Strings(w2001, w2002, "\n" ("分隔符(Tab)")) -> (w2000:string)
          }
          n1245 = String Length(string=w1991) -> (length=w1990:i32)
          n1246 = Decrement(x=w1990) -> (x-1=w1989:i32)
          n1247 = String Subset(string=w1991, length (rest)=w1989) -> (substring=w1988:string)  [unwired: 1 in]
          "校准内容显示" <- w1988
          n1248 = global read "COD内部交互全局.vi" "待机"() -> (w1987:bool)
        }
      }
      frame True {
      }
    }
    n1249 = Wait (ms)(milliseconds to wait=u32 1000 ("等待时间（毫秒）")) -> ()  [unwired: 1 out]
  }
  n1250 = while {
    stop <- FALSE stop-if-true
    w2038 = T16 0 items=["最小二乘", "最小绝对残差", "Bisquare"] ("method")
    # "计算线性、多项式公式、远程校准"
    n1251 = local read "浓度1"() -> (w2011:dbl)
    n1252 = local read "浓度2"() -> (w2040:dbl)
    n1253 = local read "浓度3"() -> (w2041:dbl)
    n1254 = local read "浓度4"() -> (w2033:dbl)
    n1255 = local read "浓度5"() -> (w2032:dbl)
    n1256 = Build Array("泵滴定数1", "泵滴定数2", "泵滴定数3", "泵滴定数4", "泵滴定数5") -> (w2039:dbl[])
    n1257 = Build Array(w2011, w2040, w2041, w2033, w2032) -> (w2007:dbl[])
    n1258 = Build Array("启用1", "启用2", "启用3", "启用4", "启用5") -> (w2010:bool[])
    n1259 = global read "CODMN外部API.vi" "远程反控校准CODMn"() -> (w2008:bool)
    n1260 = call "将启用的浓度作为新的浓度数组.vi"("启用布尔数组"=w2010, "输入浓度数组"=w2007) -> ("启用的浓度数组"=w2009:dbl[])  [unwired: 13 in]
    n1261 = Unbundle By Name("方程系数") -> ("K"=w2019:dbl, "b"=w2018:dbl, "X^2"=w2017:dbl)
    n1262 = case shown="\"多项式\"" "模型" {
      tunnel: w2019 -> [w2050 w2053]
      tunnel: w2018 -> [w2049 w2054]
      tunnel: w2017 -> [_ w2052]
      frame "线性", Default {
        "K" <- w2050
        "b" <- w2049
      }
      frame "多项式" {
        n1263 = Build Array(w2054, w2053, w2052) -> (→"多项式系数":dbl[])
      }
    }
    n1264 = call "线性公式CODMn用.vi"("标液浓度"=w2007, "监测浓度"=w2039, "启用"=w2010, "method"=w2038, "模型"="模型", "精度"=6) -> ("拟合方程"=w2025:string, "r^2"=→"r^2":dbl, "slope"=w2023:dbl, "intercept"=w2024:dbl, "XY图"=→"XY图":cluster{"X Values":dbl[], "Y Values":dbl[]}[], "Polynomial Coefficients"=w2034:dbl[])  [unwired: 8 in]
    "拟合公式" <- w2025
    n1265 = call <vilib>:"Boolean Crossing PtByPt.vi"("direction"=enum16{"either", "false-true", "true-false"}."false-true", "input"=w2008) -> ("crossing"=w2006:bool)  [unwired: 1 in]
    n1266 = case shown="真" w2006 {
      tunnel: w2007 -> [_ w2044]
      frame False {
      }
      frame True {
        n1267 = global read "CODMn断电保存全局变量.vi" "远程自动校准浓度"() -> (w2045:dbl)
        n1268 = Search 1D Array(1D array=w2044, element=w2045) -> (index of element=w2046:i32)  [unwired: 1 in]
        n1269 = case shown="0, 默认" w2046 {
          selector: w2046 -> [_ w2048]
          frame -1 {
          }
          frame 0, Default {
            n1270 = Increment(x=w2048) -> (x+1=w2047:i32)
            n1271 = global write "COD内部交互全局.vi" "当前校准"(w2047) -> ()
          }
        }
      }
    }
    n1272 = feedback #3(w2025) -> (w2026:string)
    n1273 = feedback-in #3(w2025) -> ()
    n1274 = Not Equal?(x=w2025, y=w2026) -> (x != y?=w2022:bool)
    n1275 = global write "COD内部交互全局.vi" "启用的浓度数组"(w2009) -> ()
    n1276 = case shown="真" w2022 {
      tunnel: w2034 -> [_ w2058]
      tunnel: w2024 -> [_ w2059]
      tunnel: w2023 -> [_ w2060]
      frame False {
      }
      frame True {
        # "当公式发生改变时赋值到右侧公式"
        n1277 = local read "模型"() -> (w2061:enum32{"线性", "多项式"})
        n1278 = case shown="\"多项式\"" w2061 {
          tunnel: [w2066 w2068] -> w2056
          tunnel: w2060 -> [w2066 _]
          tunnel: w2059 -> [w2065 _]
          tunnel: [w2065 w2069] -> w2057
          tunnel: w2058 -> [_ w2070]
          tunnel: [0.0 ("数值") w2067] -> w2055
          frame "线性", Default {
          }
          frame "多项式" {
            # "B,K,X^2"
            n1279 = Index Array(array=w2070) -> (element #1=w2069:dbl, element #2=w2068:dbl, element #3=w2067:dbl)  [unwired: 3 in]
          }
        }
        n1280 = Bundle By Name(cluster=cluster{"K":dbl, "b":dbl, "X^2":dbl} {"K"=0.0, "b"=0.0, "X^2"=0.0} ("方程系数"), "K"=w2056, "b"=w2057, "X^2"=w2055) -> (w2062:cluster{"K":dbl, "b":dbl, "X^2":dbl})
        n1281 = local write "方程系数"(w2062) -> ()
      }
    }
    n1282 = Wait (ms)(milliseconds to wait=u32 1000 ("等待时间（毫秒）")) -> ()  [unwired: 1 out]
  }
  n1283 = property class="VI"(reference=w4, error in=w1) -> ("Name"=w5:string)  [unwired: 2 out]
  n1284 = Open VI Reference(type specifier VI Refnum (for type only)=refnum<vi> refnum, vi path=w5, options=128 ("选项")) -> (vi reference=w7:refnum<vi>, error out=w9:errorcluster)  [unwired: 3 in]
  n1285 = call-by-ref "?"(reference=w7, error in=w9) -> (reference out=w11:refnum<vi>, error out=w10:errorcluster)  [unwired: 12 in]
  n1286 = Close Reference(reference=w11, error in (no error)=w10) -> ()  [unwired: 1 out]
